vi "Laundry SLB Main.vi"() -> ()   [LabVIEW 2014]
uses:
  type defs/DAQ_States.ctl
  <resource>/objmgr/daqmx.rc
  Utility/Labview GEA2 Toolkit v2.1/GExplorer Support/typedefs/GExplorer_Data_Cluster.ctl
  type defs/ERD_Data_Loop_Control.ctl
  type defs/Error_Command.ctl
  type defs/ERD_Loop_Control_Command.ctl
  <vilib>/DAQmx/write.llb/DAQmx Write (Digital 1D Bool NChan 1Samp 1Line).vi
  <vilib>/DAQmx/write.llb/DAQmx Write (Analog 1D DBL NChan 1Samp).vi
  <vilib>/DAQmx/create/channels.llb/DAQmx Create Channel (CI-Count Edges).vi
  <vilib>/DAQmx/read.llb/DAQmx Read (Counter U32 1Chan 1Samp).vi
  type defs/Cont_Send_States.ctl
  type defs/Cont_Send_Loop_Control_Command.ctl
  type defs/DAQ_Control_Command.ctl
  type defs/GEA2_Control_Command.ctl
  Utility/Labview GEA2 Toolkit v2.1/GEA2 Script/typedefs/Script Info.ctl
  <vilib>/DAQmx/create/channels.llb/DAQmx Create Channel (DO-Digital Output).vi
  <vilib>/DAQmx/create/channels.llb/DAQmx Create Channel (DI-Digital Input).vi
  <vilib>/DAQmx/write.llb/DAQmx Write (Digital Bool 1Line 1Point).vi
  type defs/Fault_Buffer_Status.ctl
  Utility/Save File/Public/Type Definitions/Save File File Paths.ctl
  Utility/Save File/Save File.lvlib
  user32.dll
  Utility/Labview GEA2 Toolkit v2.1/library/GEA2_Toolkit.lvlib
  <vilib>/event_ctls.llb/lveventtype.ctl
  Type Definitions/HCC Program Type.ctl
  Utility/Labview GEA2 Toolkit v2.1/type defs/ERD Write Data In.ctl
  Utility/Labview GEA2 Toolkit v2.1/type defs/ERD Read Data In.ctl
  Utility/Labview GEA2 Toolkit v2.1/type defs/Data In.ctl
  Utility/Labview GEA2 Toolkit v2.1/type defs/Data Out.ctl
  <vilib>/DAQmx/read.llb/DAQmx Read (Digital 1D Bool NChan 1Samp 1Line).vi
  <vilib>/DAQmx/read.llb/DAQmx Read (Digital 1D U8 1Chan NSamp).vi
  <vilib>/DAQmx/configure/timing.llb/DAQmx Timing (Implicit).vi
  <vilib>/DAQmx/create/channels.llb/DAQmx Create Channel (AO-Voltage-Basic).vi
  <vilib>/DAQmx/create/channels.llb/DAQmx Create Channel (CO-Pulse Generation-Frequency).vi
  <vilib>/DAQmx/configure/timing.llb/DAQmx Timing (Sample Clock).vi
  C:/Technology Lab/NI-2010/Trunk/Washer HCC/Washer HCC NEWFI/Washer Soft Load Box/build/data/GeaCommunication.dll
  build/data/GeaCommunication.dll
  type defs/ERD_Always_Show.ctl
  type defs/Cycle_Information.ctl
  type defs/Algorithms.ctl
  type defs/Version.ctl
  type defs/Programming.ctl
  type defs/Select Graph.ctl
  type defs/Motor Control.ctl
  type defs/Cycle Control.ctl
  type defs/MotorProfile.ctl
  type defs/OOB_Kicks.ctl
  type defs/Valves.ctl
  type defs/Redundant.ctl
  <vilib>/Platform/fileVersionInfo.llb/FileVersionInformation.ctl
  Utility/Labview GEA2 Toolkit v2.1/type defs/Source_Destination.ctl
  Utility/Labview GEA2 Toolkit v2.1/type defs/ERD Read Data Out.ctl
  type defs/ERD_Graph.ctl
  type defs/ERD_Graph_All.ctl
  type defs/ATC_Data.ctl
  type defs/Fault_Table_Info.ctl
  type defs/Relays.ctl
  Utility/Save File/Public/Type Definitions/Save File Washer.ctl
  Type Definitions/2015 Program/2015 Cycle Stats.ctl
  Utility/Save File/Public/Type Definitions/Save File Washer Details DOE.ctl
  Utility/Save File/Public/Type Definitions/Save File Unit Type.ctl
  Utility/Save File/Public/Type Definitions/Save File Software Version.ctl
panel:
  in  "Minimize":bool
  in  "Low Power OFF":bool
  out "ERD Data":T1
  out "Timer 2":dbl format="%<%H:%M:%S>t"
  in  "Tab Control 2":enum32{"Page 1", "ERD Read"}(tab)
  out "Washer Details.Serial Number:":string
  out "Washer Details.TR Number:":string
  out "Washer Details.Lab ID:":string
  out "ERD Data Out":T2[](array[typedef]) {"ERD Number" format="%.0x"}
  out "Raw Data Out":string[](array[string])
  in  "Verify ERD Response?":bool
  out "State":enum16{"Run", "Shutdown"}(ring)
  out "Cycle Timer":dbl format="%<%H:%M:%S>t"
  in  "Read Timeout (ms)":u32=5000
  in  "Disable Write":bool
  in  "Disable Read Previous":bool
  in  "Expected Command 2":string=".*"
  in  "Disable Expected Data":bool
  in  "Expected Data 2":string=".*"
  in  "2015 Cycle Stats":T3
  out "Washer In":T4 {"Current" format="%.2f"; "Day Cycle Count" format="%04d"}
  out "New File?":bool
  out "UI Loop":i32
  out "Description 4":string
  out "Exit from SLB":bool
  out "Handle":dbl
  out "Error":i32
  out "Start Save Routine":bool
  in  "Open Lid":bool
  in  "Sample Rate (ms)":u32=1000 min=400 step=100
  in  "Save Log":bool
  in  "Clear Button":bool
  out "Counter":dbl
  in  "Filter Data":bool=TRUE
  in  "UI Launch Button":bool
  in  "Stop":bool
  in  "Data ON":bool=TRUE
  in  "Tab Control":T9(tab)
  out "GEA2 Msg Log":string
  in  "GEA2 Send":T10={"Source"=245, "Destination"=35, "Command"=0, "Message"=""} {"Command" format="%02x"; "Destination" format="%02x"; "Source" format="%02x"}
  in  "Send Button":bool
  out "Version":T11
  in  "Programming":T12 {"Result" items=["InvalidImage", "ImageRejected", "BoardNotFound", "UnableToGetGeaConfiguration", "WriteToFlashNotAllowed", "ImageDownloadedSuccessfully", "ImagePresent", "WriteToFlashFailed", "EraseFailed", "CrcFailed", ""]}
  in  "Start Send":bool
  in  "Msg Rate (ms)":u32=1000 min=50 step=50
  in  "Board Index":i32
  out "Board ID":string
  out "Front Panel Station Label":string
  in  "Number of Cycles/ File":i32=1
  in  "Read ERD":bool
  in  "Write ERD":bool
  in  "ERD Write Data In":T13 {"ERD Number" format="%.0x"}
  in  "GEA Inputs":T14={"Source"=228, "Destination"=35} {"Destination" format="%.0x"; "Source" format="%.0x"}
  out "ERD Output":T15 {"ERD Number" format="%.0x"}
  in  "ERD Read Data In":T16 {"ERD Number" format="%.0x"}
  out "Pressure 2":dbl(graph)
  out "Temp":dbl(graph)
  out "Tub Gallons":dbl(graph)
  in  "Select Graph":T17=enum."Basket Speed (RPM)"
  out "Basket Speed":u16(graph)
  out "Motor Current":dbl(graph)
  out "ERD 3":dbl(graph)
  out "ERD 2":dbl(graph)
  out "ERD 1":dbl(graph)
  in  "Disable Graphs":bool=TRUE
  in  "ERD Graph Cntrl":T18={"ERD 3"={"ERD #"=62250, "Scaler"=32, "Data Type"=enum."uint16_t"}, "ERD 2"={"ERD #"=62250, "Scaler"=32, "Data Type"=enum."uint16_t"}, "ERD 1"={"ERD #"=62250, "Scaler"=32, "Data Type"=enum."uint16_t"}} {"ERD 1"."Scaler" min=1; "ERD 1"."ERD #" format="%.0x"; "ERD 2"."Scaler" min=1; "ERD 2"."ERD #" format="%.0x"; "ERD 3"."Scaler" min=1; "ERD 3"."ERD #" format="%.0x"}
  out "ERD Graph  Ind":T20
  in  "Relays":T21
  in  "Motor Profile":T22
  in  "Test Mode":cluster{"Exit Test Mode":bool}
  in  "LED Control":T23
  in  "Motor Control":T24 {"Amplitude (%)\n-CCW +CW" min=-100 max=100 step=5; "Acceleration" min=-400 max=400 step=10; "Motor Profile Mode" items=["Closed Loop", "Not Implemented", "Open Loop ", "Open Loop Angle ", "Coasting", "Braking", "Idle"]; "Speed (RPM)" min=-800 max=800 step=10}
  in  "Mode Shift":T25
  in  "Recirculation Pump":T26
  in  "Drain Pump":T27
  in  "Lid Lock":T28
  in  "Cycle Control":T29
  in  "Valve Control":T30
  out "Table Buffer Status":T31
  in  "Clear Fault Table":bool
  in  "Get Table Status":bool
  in  "Clear Seq":bool
  in  "Get Faults":bool
  out "Fault Entry 4":T32
  out "Fault Entry 3":T32
  out "Fault Entry 2":T32
  out "Fault Entry 1":T32
  out "Fault Entry 0":T32
  out "Seq Buffer Status":T31
  in  "Clear Fault Buffer":bool
  in  "Get Status":bool
  out "Fault Sequence Buffer":string
  out "Redundant Micro":T33
  in  "Cycle Info Button":bool
  out "Cycle Information":T34
  in  "OOB Kicks":T35
  out "Algorithm Data":T36
  out "ATC Data":T37
  in  "Script Log Path":path
  in  "Script":bool
  out "Script Pass/Fail?":bool
  out "Script Report Text":string
  in  "stop":bool
  in  "Script Path":path
  out "Script Info":T38 {"Overall Script File Progress" scale=0.0..1.0; "Elapsed time (s)" format="%#.1f"; "Current Script Progress" scale=0.0..1.0}
  out "Script Error Out":errorcluster
  in  "LL (M - A)":bool=TRUE
  in  "Lid Lock Feedback":bool
  in  "MS (M - A)":bool=TRUE
  out "DAQ Status":string
  in  "ADC Info Button":bool
  out "Motor Current ADC":u16
  out "Pressure ADC":u16
  out "Drain Pump":bool
  out "Mode Shift":bool
  out "Recirc Pump":bool
  out "Cold Valve":bool
  out "Hot Valve":bool
  out "Spray/Rinse Valve":bool
  out "Fabric SoftValve":bool
  in  "AC Power":bool=TRUE
  in  "Mode Shift FB":bool
  in  "Lid Status":bool=TRUE
  in  "Pressure":dbl(slide) min=0.0 max=5.0 step=0.5 scale=0.0..5.0 scale format="%#_3g"
  in  "Motor Current":dbl(slide)=2.5 min=0.0 max=5.0 step=0.5 scale=0.0..5.0 scale format="%#_3g"
  in  "Turn On DAQ":bool=TRUE
  out "DAQ On?":bool
  in  "Basket RPM":dbl=1.0 min=1.0 max=800.0 step=5.0
  in  "Temperature":dbl(slide)=2.5 min=0.0 max=5.0 step=0.5 scale=0.0..5.0 scale format="%#_3g"
  out "Triac CW":bool
  out "Traic CCW":bool
  out "Temp ADC":u16
  out "CCW":u32
  out "CW":u32
  out "Exe Path":path
  in  "Record Current Status":bool
  out "Error Out":errorcluster
  in  "Error In":errorcluster
  in  "File Locations":T39
  in  "Configuration Path Main":path=path "C:/Newfi Exe/Newfi Exe Locations.ini"
  in  "FileVersionInfo":T6
  out "FileVersionInfo Out":T6
  in  "Robocopy Location Command":string="C:\\Newfi Exe\\Robocopy Update.bat"
  in  "Network Variable Update Rate":u32=1000
  # "Software Version"
  # "Critical Version"
  # "Non-Critical"
  # "XML Crit Ver"
  # "XML Non-Crit"
  # "Daily Build"
  # "Must input a valid ERD# and Data Type\nDO NOT Leave Blank \nIf no scaler use value of 01"
  # "UI"
  # "Wet Load Size"
  # "Dry Load Size"
  # "OOB"
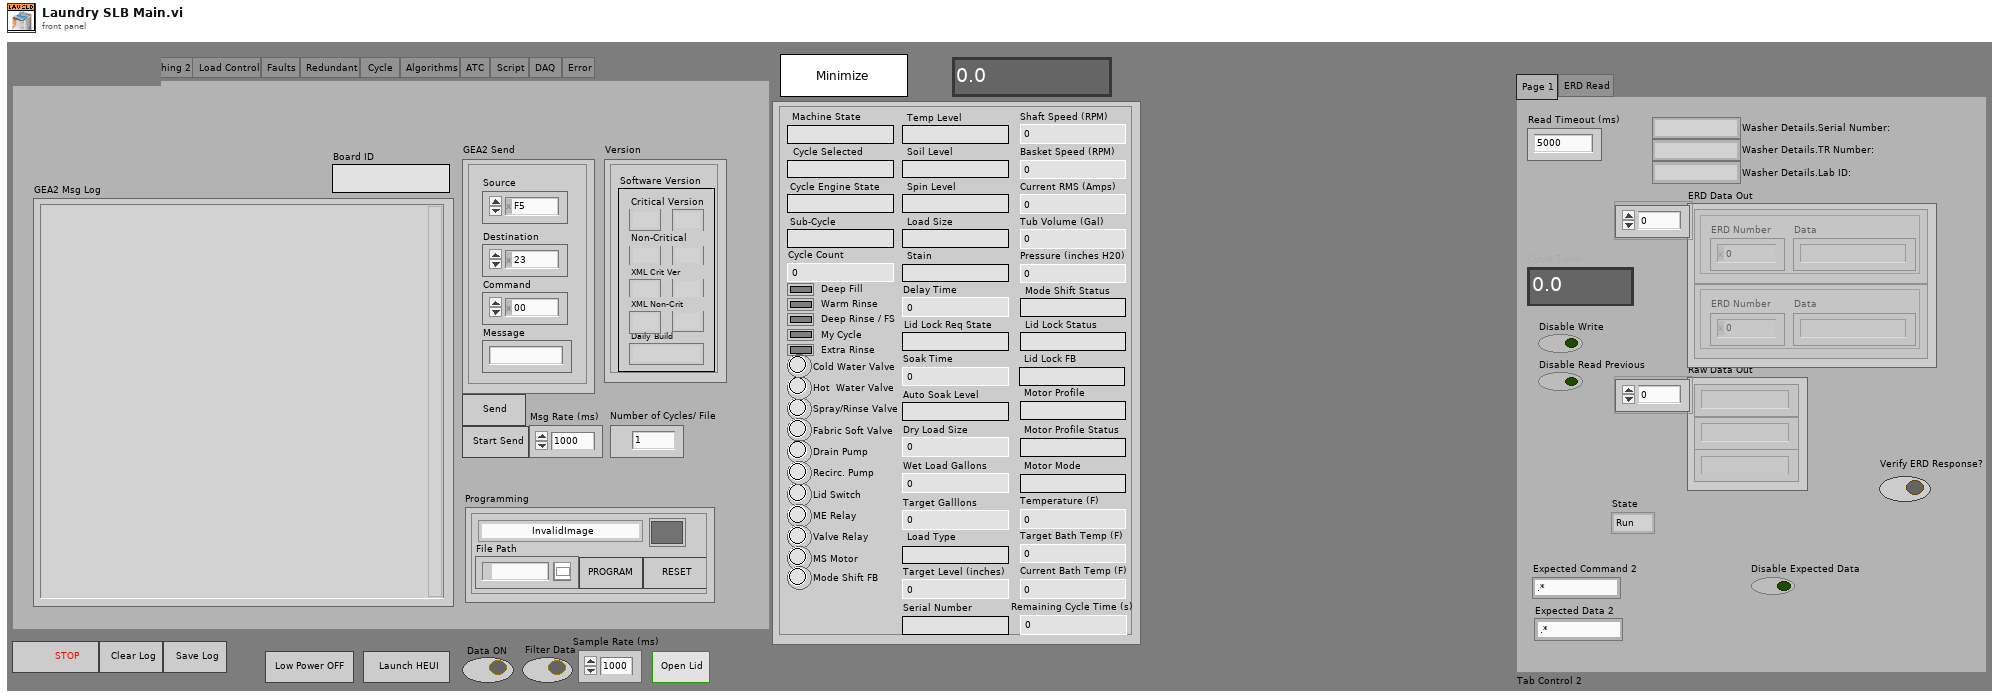
[diagram p1: front panel]
types:
  T1 = typedef "ERD_Always_Show.ctl" = cluster{"Basket Speed (RPM)":u16, "Machine State":string, "Tub Volume (Gal)":dbl, "Pressure (inches H20)":dbl, "Lid Switch ":bool, "Current RMS (Amps)":dbl, "Cycle Selected":string, "Lid Lock Status":string, "Mode Shift Status":string, "Spray/Rinse Valve":bool, "Fabric Soft Valve":bool, "Drain Pump":bool, "Recirc. Pump":bool, "Cycle Engine State":string, "Hot  Water Valve":bool, "Cold Water Valve":bool, "Motor Profile":string, "Motor Profile Status":string, "Motor Mode":string, "ME Relay":bool, "Cycle Count":u32, "Deep Rinse / FS":bool, "My Cycle":bool, "Soil Level":string, "Spin Level":string, "Stain":string, "Temp Level":string, "Load Size":string, "Delay Time":u16, "Soak Time":u16, "Deep Fill":bool, "Warm Rinse":bool, "Auto Soak Level":string, "Extra Rinse":bool, "Wet Load Gallons":dbl, "Target Galllons":dbl, "Sub-Cycle":string, "Load Type":string, "Target Level (inches)":u32, "Valve Relay":bool, "Dry Load Size":dbl, "Shaft Speed (RPM) ":u16, "MS Motor":bool, "Mode Shift FB":bool, "Target Bath Temp (F)":dbl, "Temperature (F)":dbl, "Current Bath Temp (F)":dbl, "Lid Lock FB":string, "Lid Lock Req State":string, "Remaining Cycle Time (s)":dbl, "Serial Number":string}
  T2 = typedef "GEA2_Toolkit.lvlib/ERD Read Data Out.ctl" = cluster{"ERD Number":u16, "Data":string}
  T3 = typedef "2015 Cycle Stats.ctl" = cluster{"Cycle Time (Minutes)":dbl, "Max Temp":dbl, "Max Basket Speed":dbl, "Max Motor Current":dbl, "Max Tub Volume":dbl, "Max Pressure (H2O)":dbl, "Cycle Count":dbl, "Max Shaft Speed ":dbl, "Max Red. Pressure":dbl, "Max. Red Shaft Speed":dbl}
  T4 = typedef "Save File.lvlib/Save File Washer.ctl" = cluster{"Serial Number Display":string, "Day Cycle Count":i32, "Station Label":string, "Status Color":u32, "Current Run Start Time":dbl, "Error?":bool, "Washer Details":T5, "Board ID":string, "Boolean":bool, "RPM":u32, "Current":dbl, "Current Path":path, "Saving":bool, "Unit Type":T7, "Software Version":T8, "Total Time On":dbl}
  T5 = typedef "Save File.lvlib/Save File Washer Details DOE.ctl" = cluster{"Engineer:":string, "Model Number:":string, "Serial Number:":string, "Comments:":string, "Station ID:":string, "Technician:":string, "TR Number:":string, "Lab ID:":string, "Supply Voltage":string, "Water Pressure (PSI):":string, "File Path":path, "Hot Water Temperature (Fahrenheit)":string, "Cold Water Temperature (Fahrenheit)":string, "Capacity (cu.ft)":dbl, "Initial Cloth Weight:":dbl, "Cloth Lot:":i32, "Model Family":string, "Program Name":string, "Cycle Selection":string, "Wash Temperature":string, "Rinse Temperature":string, "Load Size":string, "FileVersionInfo":T6, "Test Date":string, "Computer Name":string, "IP Address":string, "Test Station":string, "Engineer":string, "Test Name":string, "Ambient RH:":string, "Supply Voltage":string, "Frequency:":string, "Build:":string}
  T6 = typedef "FileVersionInformation.ctl" = cluster{"FileVersion":string, "ProductName":string, "InternalName":string, "CompanyName":string, "LegalCopyright":string, "FileDescription":string}
  T7 = typedef "Save File.lvlib/Save File Unit Type.ctl" = enum32{"", "Viper", "Hawk", "2015", "Other"}
  T8 = typedef "Save File.lvlib/Save File Software Version.ctl" = cluster{"Critical Major SW Version":string, "Critical Minor SW Version":string, "Major SW Version":string, "Minor SW Version":string, "Parametric Data Ver. Major":string, "Parametric Data Ver. Minor":string, "Diagnostics Data Ver. Major":string, "Diagnostics Data Ver. Minor":string, "Current Personality Setting":string}
  T9 = enum32{"GEA2", "ERD", "Graphing", "Graphing 2", "Load Control", "Faults", "Redundant", "Cycle ", "Algorithms", "ATC", "Script", "DAQ", "Error"}
  T10 = typedef "GEA2_Toolkit.lvlib/Data In.ctl" = cluster{"Source":u8, "Destination":u8, "Command":u8, "Message":string}
  T11 = typedef "Version.ctl" = cluster{"Critical Major":string, "Critical Minor":string, "Non-Critical Minor":string, "Non-Critical Major":string, "XML Crit Minor":string, "XMLCrit Major":string, "Daily Rev":string, "XML Non-crit Minor":string, "Xml Non-crit Major":string}
  T12 = typedef "Programming.ctl" = cluster{"Program":bool, "File Path":path, "Program Ind":bool, "Result":i32, "Reset Board":bool}
  T13 = cluster{"ERD Number":u16, "Data Type":enum16{"string", "boolean", "uint8_t", "uint16_t", "uint32_t"}, "Data":string}
  T14 = typedef "GEA2_Toolkit.lvlib/Source_Destination.ctl" = cluster{"Source":u8, "Destination":u8}
  T15 = cluster{"ERD Number":u16, "   00 01 02 03 04 05 06 07 08 09 10 11 12 13 14 15 16 17 18 19 ":string}
  T16 = typedef "GEA2_Toolkit.lvlib/ERD Read Data In.ctl" = cluster{"ERD Number":u16, "Data Type":enum16{"string", "boolean", "uint8_t", "uint16_t", "uint32_t", "uint64_t"}}
  T17 = typedef "Select Graph.ctl" = enum16{"Temperature (F)", "Basket Speed (RPM)", "Tub Volume (Gal)", "Pressure (in H2O)", "Current RMS (Amps)", "ERD 1", "ERD 2", "ERD 3"}
  T18 = typedef "ERD_Graph_All.ctl" = cluster{"ERD 3":T19, "ERD 2":T19, "ERD 1":T19}
  T19 = typedef "ERD_Graph.ctl" = cluster{"ERD #":u16, "Scaler":u32, "Data Type":enum16{"string", "boolean", "uint8_t", "uint16_t", "uint32_t"}}
  T20 = cluster{"ERD Value 1":dbl, "ERD Value 2":dbl, "ERD Value 3":dbl}
  T21 = typedef "Relays.ctl" = cluster{"Relays ON":bool, "Relays OFF":bool}
  T22 = typedef "MotorProfile.ctl" = cluster{"Start Profile":bool, "Profile Selection":u8, "Stop Profile":bool, "Pause Profile":bool, "Resume Profile":bool, "Select Profile":bool}
  T23 = cluster{"ALL LEDs ON":bool, "ALL LEDs OFF":bool, "Reset LEDs":bool}
  T24 = typedef "Motor Control.ctl" = cluster{"Speed (RPM)":i16, "Motor Profile Mode":u16, "Acceleration":i16, "Angle (Degrees)":i16, "Amplitude (%)\n-CCW +CW":i16, "Start Motor":bool, "Stop Motor":bool}
  T25 = cluster{"Shift to Agitate":bool, "Shift to Spin":bool, "Disable":bool}
  T26 = cluster{"Recirc Pump ON":bool, "Recirc Pump OFF":bool, "Reset Recirc Pump":bool}
  T27 = cluster{"Dain Pump ON":bool, "Drain Pump OFF":bool, "Reset Drain Pump":bool}
  T28 = cluster{"Lock Lid":bool, "Unlock Lid":bool, "Reset Lock":bool}
  T29 = typedef "Cycle Control.ctl" = cluster{"Start Cycle":bool, "Cycle Selection":u8, "Stop Cycle":bool, "Pause Cycle":bool, "Resume Cycle":bool, "Select Cycle":bool}
  T30 = typedef "Valves.ctl" = cluster{"Cold Valve":bool, "SprayRinse Valve":bool, "FabricSoftener Valve":bool, "Valves ON":bool, "Valves OFF":bool, "Hot Valve ":bool}
  T31 = typedef "Fault_Buffer_Status.ctl" = cluster{"Current Index":u16, "Count":u16, "Overwrite Count":u16}
  T32 = typedef "Fault_Table_Info.ctl" = cluster{"Cycle Count":u32, " Runtime (min) ":u32, "Fault Status":string, "Fault ID":string, "Fault Count":u16}
  T33 = typedef "Redundant.ctl" = cluster{"Version":string, "Personality":u8, "Pressure ":dbl, "Shaft Speed":u16, "Modeshift Feedback":string, "Lid Switch":bool, "Lid Lock":bool, "Triac Enable":bool, "Drain Pump":bool, "Lid Lock Motor Speed Safety Interlock":bool, "Flood Condition State":bool, "Lid Open Fault State":bool, "Access To Moving Parts State":bool, "Heartbeat":bool, "Motor Enable":bool, "Lid Unlock Fault State":bool}
  T34 = typedef "Cycle_Information.ctl" = cluster{"MyCycle":bool, "Delay":bool, "Extra Rinse":bool, "Deep Fill":bool, "AutoSoak":bool, "Deep Rinse":bool, "Warm Rinse":bool, "Delay Time":string, "Stain":string, "Autosoak Time":string, "Cycle Selection":string, "Stain":bool}
  T35 = typedef "OOB_Kicks.ctl" = cluster{"OOB in Accel":bool, "OOB in S-S":bool, "Redist Req":bool}
  T36 = typedef "Algorithms.ctl" = cluster{"Wet Load Gal":dbl, "Target Gallons":dbl, "Load Type":string, "Load Size":string, "Coast Time":u16, "Ramp Time":u16, "Ramp  Speed":u16, "Ramp Avg Current":dbl, "OOB Redist Req":bool, "OOB Detected in S-S":bool, "Max Accel in Accel":i32, "Max Jerk in Accel":i32, "Max Jerk in S-S":i32, "OOB Detected in Accel":bool, "Partial Coast Time":u16, "Dry Load Size":dbl, "Ramp Line Voltage ":dbl, "Coast Line Voltage":dbl}
  T37 = typedef "ATC_Data.ctl" = cluster{"Current Tub Gallons":dbl, "Hot Gallons":dbl, "Cold Gallons":dbl, "Target Gallons":dbl, "Current Water Temp":dbl, "Target Level":u32, "Target Bath Temp":dbl, "Current Bath Temp ":dbl, "Cold Inlet Temp":dbl, "Hot Inlet Temp":dbl, "Warm Inlet Temp":dbl, "Hot Seg Valve Time":u16, "Cold Seg Valve Time ":u16, "User Temp Level":string, "Segment Gallons":dbl}
  T38 = typedef "Script Info.ctl" = cluster{"Overall Script File Progress":dbl, "Current Script Progress":dbl, "Script":string, "Test":string, "Elapsed time (s)":dbl, "Done?":bool}
  T39 = typedef "Save File.lvlib/Save File File Paths.ctl" = cluster{"Log Debug File":path, "Log Inverter File":path, "Summary File":path, "Bus File":path, "Current (Amps) File":path}
  T40 = typedef "GEA2_Toolkit.lvlib/ERD Write Data In.ctl" = cluster{"ERD Number":u16, "Data Type":enum16{"string", "boolean", "uint8_t", "uint16_t", "uint32_t"}, "Data":string}
  T41 = typedef "HCC Program Type.ctl" = enum16{"Viper Hawk", "2015"}
  T42 = typedef "Cont_Send_States.ctl" = enum16{"Run", "Shutdown"}
  T43 = typedef "DAQ_States.ctl" = enum16{"Wait for Init", "Verify Hardware", "Initialize", "Run", "Shutdown", "Exit"}
  T44 = typedef "ERD_Data_Loop_Control.ctl" = cluster{"Data":variant, "State":enum16{"Run", "Shutdown"}}
  T45 = typedef "GEA2_Toolkit.lvlib/Data Out.ctl" = cluster{"Source":u8, "Destination":u8, "Command":u8, "Length":u8, "CRC":u16, "Message":string}
  T46 = typedef "GExplorer_Data_Cluster.ctl" = cluster{"Data":variant, "State":enum16{"Add to Log", "Clear", "Shutdown"}}
  T47 = typedef "ViperHawk Data.ctl" = cluster{"Message Count":dbl, "ReceivedData":u8[], "Partial Message String":string, "Full Message to Save":string, "Data to send":u8[], "Command":u8, "logData":T48, "Number of Messages":i32, "Debug":string[][], "Washer In":T4, "Configuration File Path out":path}
  T48 = typedef "ViperHawk logData.ctl" = cluster{"IGBT Temp (Deg C)":u8, "Speed":u32, "Load Size":u32, "Temperature":u8, "Water Pressure":u32, "Detergent":u32, "Fabric Softener":u32, "Direction":string, "Det":bool, "FS":bool, "Recirc":bool, "Drain":bool, "Hot":bool, "Cold":bool, "LidClosed":bool, "LidLocked":bool, "Motor Speed":u16, "Latched Out Of Balance":u16, "Raw Out Of Balance":u16, "Plaster Status":u8, "Inverter Power (Watts)":u16, "Profiler Status":string, "Profiler CRC":u16, "Current Inverter Action":string, "Target Speed (BRPM)":u16, "Latched Agitate Motor Temp (Deg C)":u8, "Current Motor Temp (Deg C)":u8, "Error Codes 1":string}
  T49 = typedef "ViperHawk Timers.ctl" = cluster{"Cycle Timer":dbl, "Timer":dbl}
  T50 = typedef "Save File.lvlib/Save File FileName Control.ctl" = cluster{"Debug File DIR":string, "Inverter And MC File DIR":string}
  T51 = typedef "ViperHawk Search Control.ctl" = cluster{"Pause":string[], "Run":string[], "EOC":string[], "Error Codes":string[]}
  T52 = typedef "ViperHawk Diagnostic Data.ctl" = cluster{"Cycle Buffer Index":string, "Page Number":string, "Total Cycle Count":u32, "Delay Start Time":u32, "Stain Selected":string, "Selected Cycle":u32, "eWash":string, "Soil Level":string, "Temperature":string, "Overnight Ready":string, "Spin Setting":string, "Control Lock Status":string, "Stain Remover":string, "Steam Assist":string, "My Cycle":string, "PreWash":string, "Debug Log Enabled":string, "Rinse":string, "Signal Level":string, "PreSoak":string, "Speed (RPM)":u32, "Load Size":u32, "Temperature":u32, "Water Pressure":u32, "Detergent":u32, "Fabric Softener":u32, "Tub Direction":string, "Detergent Valve":bool, "Fabric Softener Valve":bool, "Recirculating Pump":bool, "Drain Valve":bool, "Hot Valve":bool, "Cold Valve":bool, "Lid Closed Status":string, "Lid Lock Status":string, "Error Count":u32, "IGBT Temperature (Deg C)":u32, "Motor Speed":u32, "Latched OOB":u32, "Raw OOB":u32, "Plaster Status":u32, "Inverter Power (W)":u32, "Target Speed(BRPM)":u32, "Latched Agitate Motor Temp (Deg C)":u32, "Current Motor Temp (Deg C)":u32, "Profiler Status":string, "Current Inverter Action":string, "Error Codes":string, "Total Cycle Time (Min)":u32, "Total Cycle Count (Current)":u16, "Total Error Count":u16, "Machine Error History":u32, "Washer UI History":u32, "Inverter Error History":u32, "Cycle Storage Limit":u8, "Error Storage Limit":u8, "Cycle Pages Supported":u8, "Error Pages Supported":u8, "Inverter Reset Count":u16}
  T53 = cluster{"Initialize":T47, "Timers":T49, "Configuration Startup Directorys":T50, "Debug Search Parameters":T51, "Log Debug and Inv? Startup":bool, "Board Index Startup":i32, "File Locations":T39, "GeaCommunication.GeaBus":refnum<k24>, "GEA2 Event Registration":refnum<event-registration>, "New Summary Created":bool, "Files Already Exist":bool, "Diagnostic":T52}
  T54 = typedef "LabVIEW_GEA2_Toolkit.lvlibp/Data In.ctl" = cluster{"Source":u8, "Destination":u8, "Command":u8, "Message":string}
  T55 = enum8{"Enabled", "Disabled", "Disabled and Grayed Out"}
  T56 = typedef "GEA2_Control_Command.ctl" = enum16{"Initialize", "Shutdown"}
  T57 = typedef "DAQ_Control_Command.ctl" = enum16{"Initialize", "Shutdown"}
  T58 = typedef "Cont_Send_Loop_Control_Command.ctl" = enum16{"Initialize", "Shutdown"}
  T59 = typedef "ERD_Loop_Control_Command.ctl" = enum16{"Initialize", "Shutdown"}
  T60 = cluster{"ERD Number":u16, "Data Type":enum16{"string", "boolean", "uint8_t", "uint16_t", "uint32_t"}, "Data":string}[]
  T61 = enum32{"Invalid", "Standard", "Closed", "Hidden", "Minimized", "Maximized"}
  T62 = enum32{"invalid app kind", "Development System", "Run Time System", "Student Edition", "Embedded LabVIEW", "Evaluation", "Custom"}
  T63 = enum16{"Read Viper", "Write Viper", "Read 2015", "Write 2015"}
  T64 = cluster{"Core":cluster{"Current VI Reference":refnum<vi>, "Close Panel on Exit?":bool}, "File Locations":T39, "Washer In":T4, "File Refnum":refnum<file>, "FileVersionInfo":T6, "2015 Cycle Stats":T3, "ERD Data Save":T1}
  T65 = cluster{"Current VI Reference":refnum<vi>, "Close Panel on Exit?":bool}
  T66 = typedef "lveventtype.ctl" = enum32{"Null", "Timeout", "Annotation Menu Selection", "Annotation Menu Selection?", "App Instance Close", "App Instance Close?", "Autoscale Range Change", "Bookmark Info Change", "Cell Edit", "Cell Edit?", "Cursor Grab", "Cursor Grab?", "Cursor Menu Selection", "Cursor Menu Selection?", "Cursor Move", "Cursor Release", "Data Change", "Direction Change", "Display State Change", "Drag Ended", "Drag Enter", "Drag Leave", "Drag Over", "Drag Source Update", "Drag Starting", "Drag Starting?", "Drop", "Exec State Change", "Key Down", "Key Down?", "Key Repeat", "Key Repeat?", "Key Up", "Listbox Double Click", "Menu Activation?", "Menu Selection (App)", "Menu Selection? (App)", "Menu Selection (User)", "Mouse Down", "Mouse Down?", "Mouse Enter", "Mouse Leave", "Mouse Move", "Mouse Up", "Mouse Wheel", "NI Security User Change (App)", "Pane Size", "Panel Close", "Panel Close?", "Panel Resize", "Plot Attribute Change", "Scale Range Change", "Shortcut Menu Activation?", "Shortcut Menu Selection (App)", "Shortcut Menu Selection? (App)", "Shortcut Menu Selection (User)", "Tree Double Click", "Tree Drag", "Tree Drag?", "Tree Drop", "Tree Drop?", "Tree Item Close", "Tree Item Close?", "Tree Item Open", "Tree Item Open?", "User Event", "Value Change"}
  T67 = typedef "Error_Command.ctl" = enum16{"Initialize", "Handle Errors", "Report Errors"}
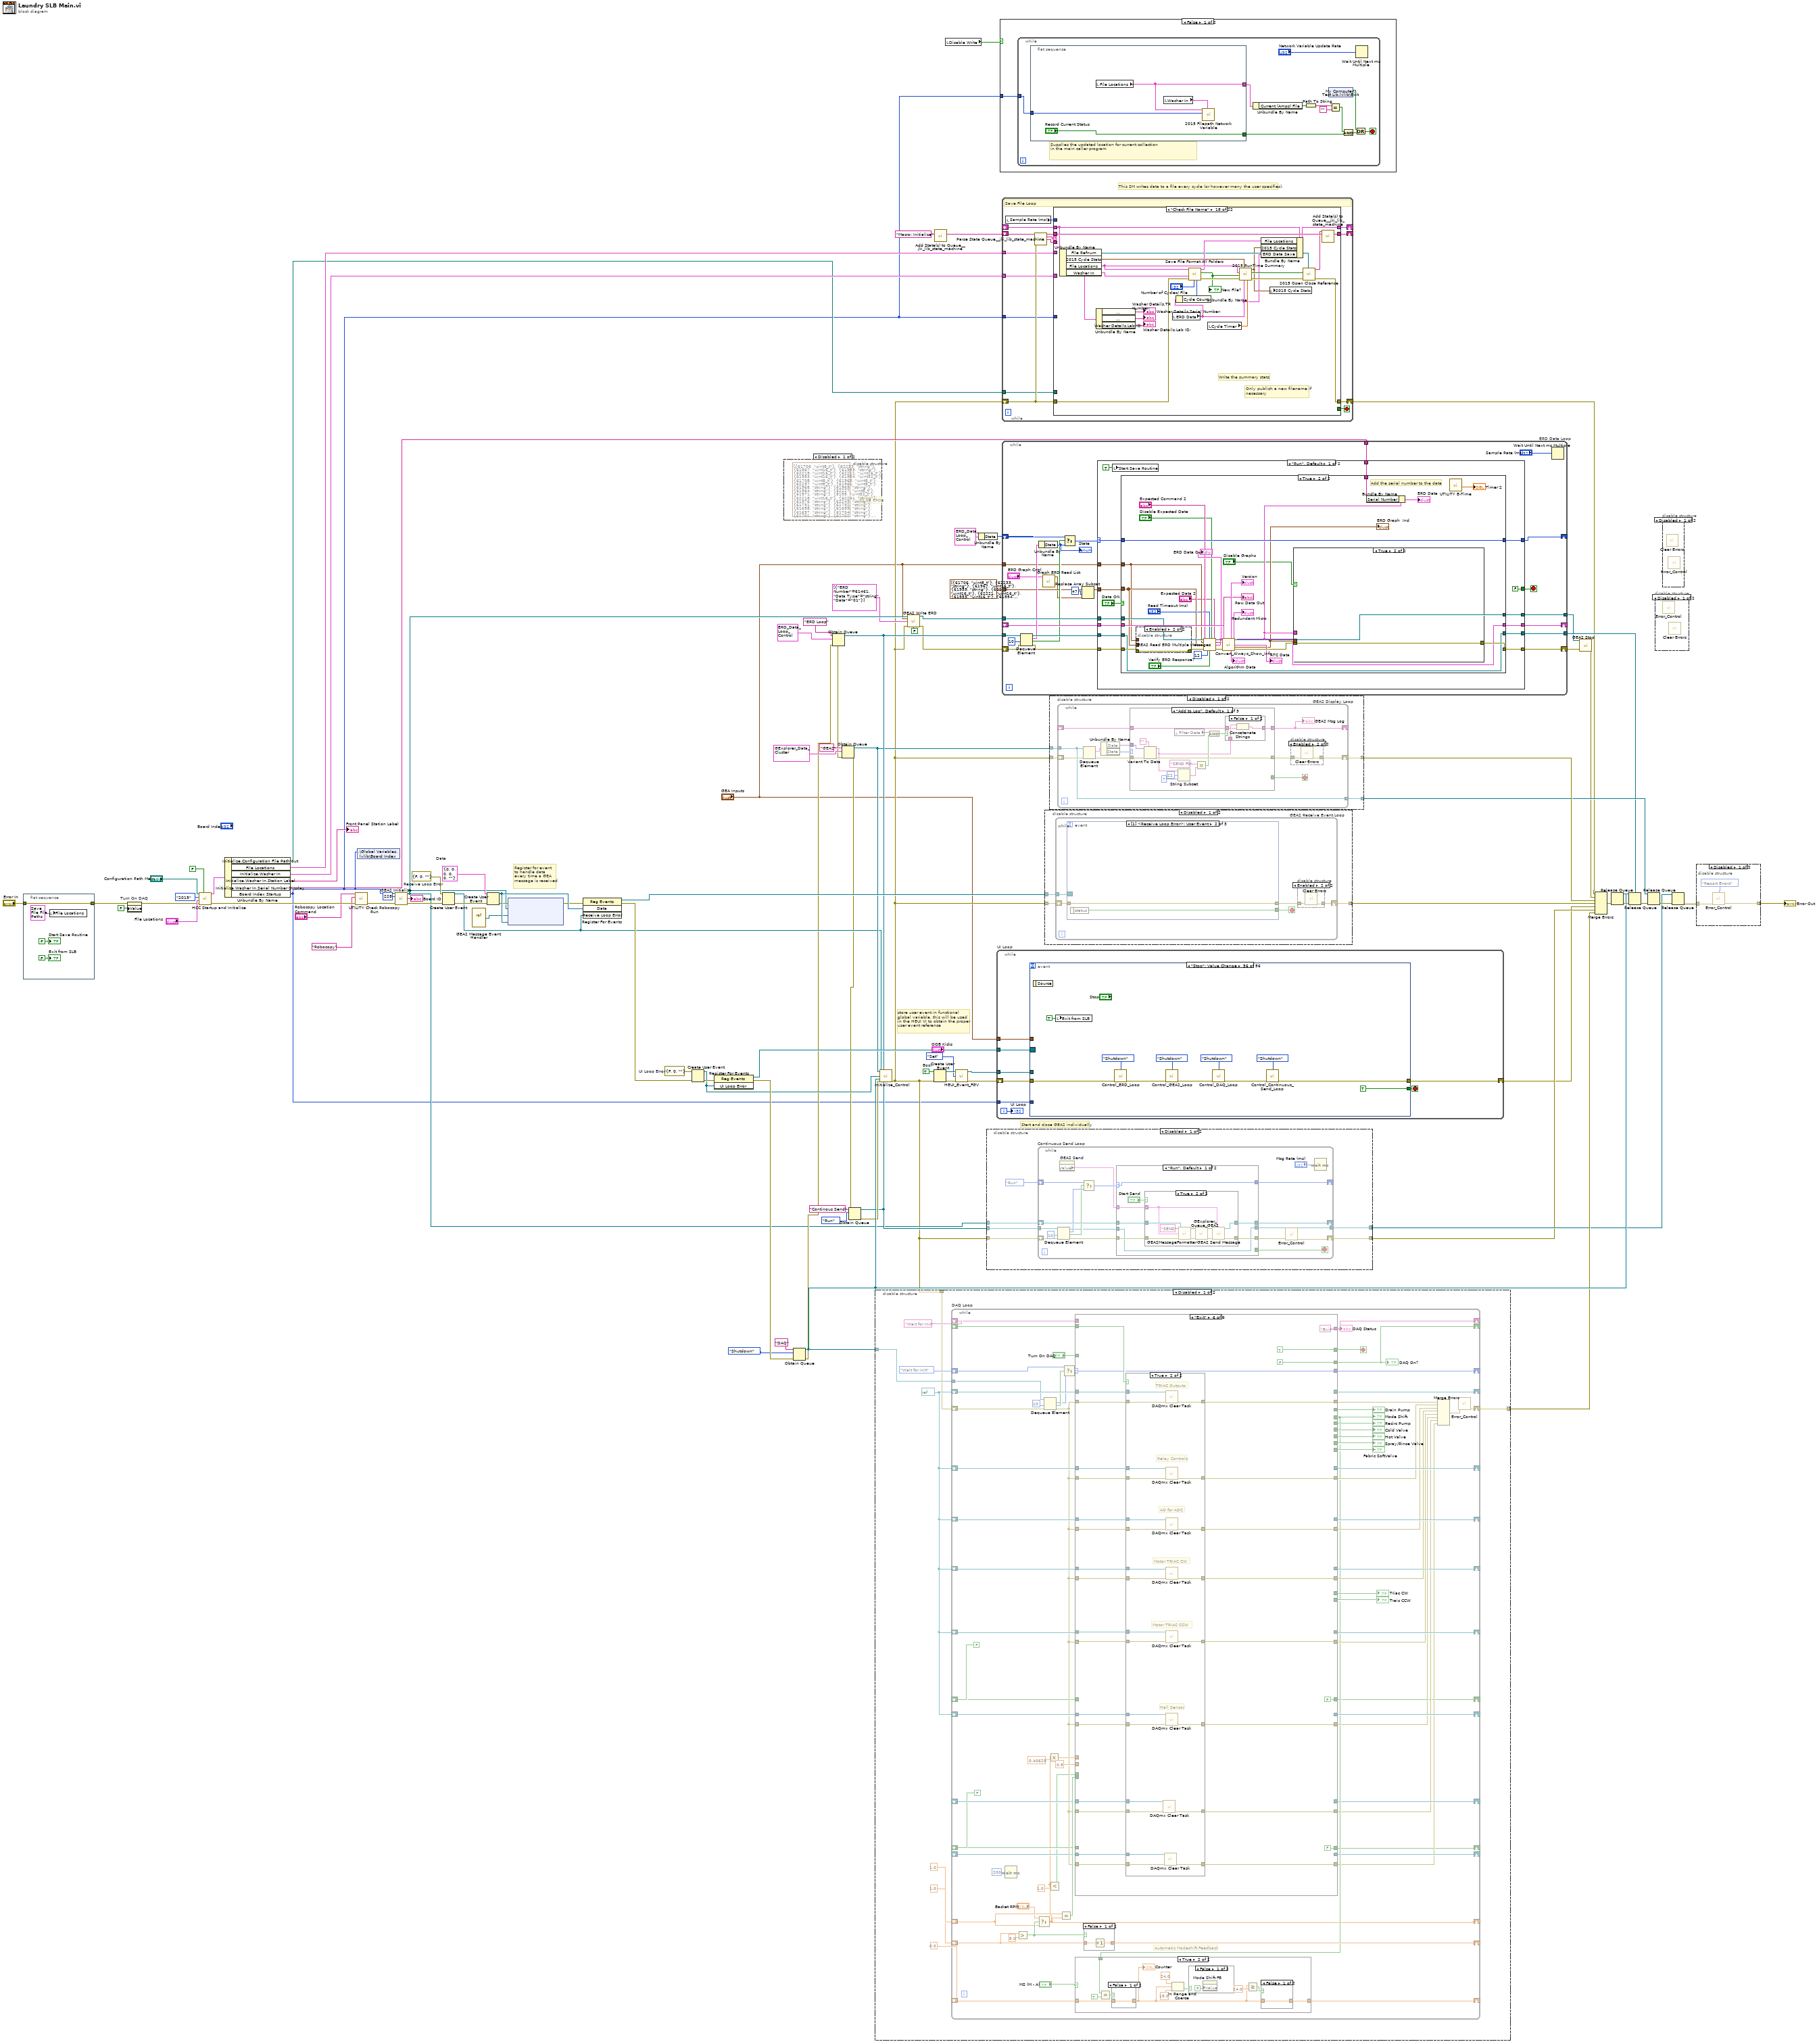
[diagram p0: block diagram]
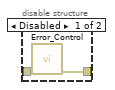
[diagram p6: hidden frame]
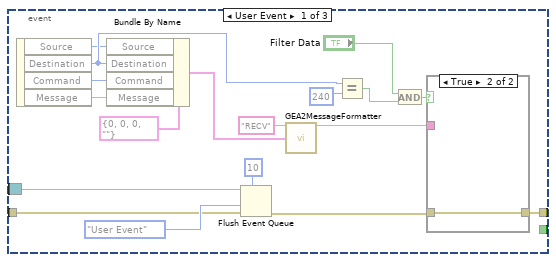
[diagram p7: hidden frame]
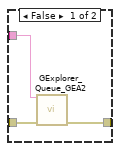
[diagram p8: hidden frame]
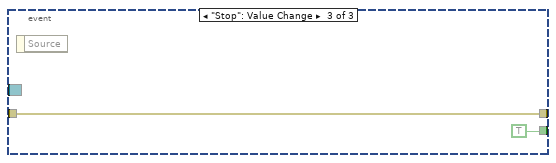
[diagram p9: hidden frame]
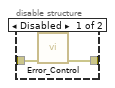
[diagram p11: hidden frame]
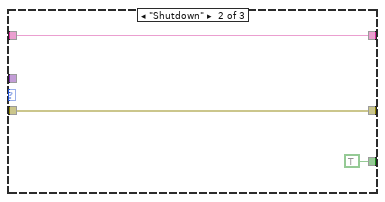
[diagram p13: hidden frame]
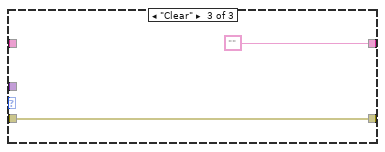
[diagram p14: hidden frame]
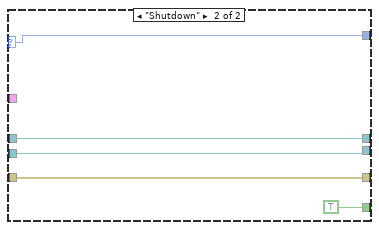
[diagram p18: hidden frame]
diagram:
  w42 = TRUE  # Bool
  w70 = errorcluster {"status"=FALSE, "code"=0, "source"=""}  # UI Loop Error
  w71 = errorcluster {"status"=FALSE, "code"=0, "source"=""}  # Receive Loop Error
  w75 = T45 {"Source"=0, "Destination"=0, "Command"=0, "Length"=0, "CRC"=0, "Message"=""}  # Data
  # "Start and close GEA2 individually"
  # "This SM writes data to a file every cycle (or however many the user specifies)."
  # "store user event in functional\nglobal variable, this will be used\nin the HEUI VI to obtain the proper\nuser event reference"
  # "Register for event\nto handle data\nevery time a GEA\nmessage is received"
  n1 = flat-sequence {
    tunnel: "Error In" -> [w93]
    tunnel: [w93] -> w30
    frame #0 {
      n2 = local write "File Locations"(T39 {"Log Debug File"=path "", "Log Inverter File"=path "", "Summary File"=path "", "Bus File"=path "", "Current (Amps) File"=path ""} ("File Locations")) -> ()
      "Start Save Routine" <- FALSE ("Start Save Routine")
      "Exit from SLB" <- FALSE ("Exit from SLB")
    }
  }
  n3 = property on="Turn On DAQ" class="Bool (strict)"(error in=w30, "Value"=FALSE ("Turn On DAQ")) -> (error out=w29:errorcluster)  [unwired: 1 in, 1 out]
  n4 = call "HCC Startup and Initialize.vi"("Debug"=FALSE, "error in (no error)"=w29, "File Locations"="File Locations", "Program"=HCC_Program_Type."2015", "Configuration Path Main"="Configuration Path Main") -> ("error out"=w7:errorcluster, "Initialization"=w35:T53)  [unwired: 5 in]
  n5 = Unbundle By Name(w35) -> ("Initialize.Configuration File Path out"=w23:path, "File Locations"=w25:T39, "Initialize.Washer In"=w26:T4, "Initialize.Washer In.Station Label"=→"Front Panel Station Label":string, "Initialize.Washer In.Serial Number Display"=w32:string, "Board Index Startup"=w3:i32)
  n6 = call "UTILITY Check Robocopy Run.vi"("error in (no error)"=w7, "Refresh Programs Named"="Robocopy", "Robocopy Location Command"="Robocopy Location Command") -> ("error out"=w6:errorcluster)  [unwired: 8 in]
  n7 = shared-variable ".\\Global Variables.lvlib\\Board Index"(w3) -> ()  [unwired: 1 in, 1 out]
  n8 = call "GEA2 Initialize.vi"("Board Index"=w3, "Source Address"=u8 228, "error in"=w6) -> ("GeaCommunication.GeaBus"=w15:refnum<k24>, "Board ID"=→"Board ID":string, "error out"=w73:errorcluster)  [unwired: 10 in]
  n9 = Create User Event(user event datatype=w71, error in=w73) -> (user event=w58:refnum<user-event>, error out=w72:errorcluster)
  n10 = vi-ref "GEA2 Message Event Handler.vi"() -> (w24:refnum<vi>)
  n11 = Create User Event(user event datatype=w75, error in=w72) -> (user event=w78:refnum<user-event>, error out=w77:errorcluster)
  n12 = node(w77, w15, w24, w78) -> (w76:errorcluster)  [unwired: 1 in, 1 out]
  n13 = register-events(error in=w76, w78, w58) -> (reference out=w74:refnum<event-registration>, error out=w66:errorcluster)  [unwired: 1 in]
  n14 = Create User Event(user event datatype=w70, error in=w66) -> (user event=w57:refnum<user-event>, error out=w69:errorcluster)
  n15 = register-events(error in=w69, w57) -> (reference out=w68:refnum<event-registration>, error out=w67:errorcluster)  [unwired: 1 in]
  n16 = disable-structure shown="Disabled" {
    frame Disabled {
      (unwired) T16[] [{"ERD Number"=61706, "Data Type"=enum."uint8_t"}, {"ERD Number"=62233, "Data Type"=enum."string"}, {"ERD Number"=61967, "Data Type"=enum."uint16_t"}, {"ERD Number"=61959, "Data Type"=enum."string"}, {"ERD Number"=62219, "Data Type"=enum."uint16_t"}, {"ERD Number"=62221, "Data Type"=enum."uint16_t"}, {"ERD Number"=61953, "Data Type"=enum."uint16_t"}, {"ERD Number"=61954, "Data Type"=enum."uint32_t"}, {"ERD Number"=61708, "Data Type"=enum."uint8_t"}, {"ERD Number"=61963, "Data Type"=enum."uint8_t"}, {"ERD Number"=62237, "Data Type"=enum."uint8_t"}, {"ERD Number"=61961, "Data Type"=enum."uint8_t"}, {"ERD Number"=61968, "Data Type"=enum."string"}, {"ERD Number"=61969, "Data Type"=enum."string"}, {"ERD Number"=61964, "Data Type"=enum."string"}, {"ERD Number"=62227, "Data Type"=enum."uint8_t"}, {"ERD Number"=61971, "Data Type"=enum."string"}, {"ERD Number"=8195, "Data Type"=enum."uint32_t"}, {"ERD Number"=62218, "Data Type"=enum."uint16_t"}, {"ERD Number"=62241, "Data Type"=enum."string"}, {"ERD Number"=61976, "Data Type"=enum."string"}, {"ERD Number"=62243, "Data Type"=enum."string"}, {"ERD Number"=61731, "Data Type"=enum."string"}, {"ERD Number"=61732, "Data Type"=enum."string"}, {"ERD Number"=61698, "Data Type"=enum."string"}, {"ERD Number"=61699, "Data Type"=enum."string"}, {"ERD Number"=61697, "Data Type"=enum."string"}, {"ERD Number"=61704, "Data Type"=enum."string"}, {"ERD Number"=61701, "Data Type"=enum."string"}, {"ERD Number"=61702, "Data Type"=enum."string"}, {"ERD Number"=61705, "Data Type"=enum."string"}, {"ERD Number"=61703, "Data Type"=enum."string"}, {"ERD Number"=61709, "Data Type"=enum."uint16_t"}, {"ERD Number"=61710, "Data Type"=enum."uint16_t"}, {"ERD Number"=61726, "Data Type"=enum."string"}, {"ERD Number"=62213, "Data Type"=enum."uint16_t"}, {"ERD Number"=61952, "Data Type"=enum."uint16_t"}, {"ERD Number"=61957, "Data Type"=enum."uint16_t"}, {"ERD Number"=61958, "Data Type"=enum."string"}, {"ERD Number"=61973, "Data Type"=enum."uint32_t"}, {"ERD Number"=62242, "Data Type"=enum."string"}, {"ERD Number"=256, "Data Type"=enum."string"}, {"ERD Number"=61441, "Data Type"=enum."string"}, {"ERD Number"=61457, "Data Type"=enum."string"}, {"ERD Number"=61984, "Data Type"=enum."uint16_t"}, {"ERD Number"=61985, "Data Type"=enum."uint16_t"}] ("Read ERD List")
      # "v1.16 ERDs"
    }
    frame Enabled {
    }
  }
  n17 = Obtain Queue(name (unnamed)="DAQ", element data type=DAQ_States."Shutdown" ("t"), error in (no error)=w67) -> (queue out=w56:refnum<queue>, error out=w19:errorcluster)  [unwired: 2 in, 1 out]
  n18 = Obtain Queue(name (unnamed)="ERD Loop", element data type=T44 {"Data"=variant, "State"=enum."Run"} ("Data"), error in (no error)=w19) -> (queue out=w60:refnum<queue>, error out=w61:errorcluster)  [unwired: 2 in, 1 out]
  n19 = Obtain Queue(name (unnamed)="GEA2", element data type=T46 {"Data"=variant, "State"=enum."Add to Log"} ("Data"), error in (no error)=w61) -> (queue out=w59:refnum<queue>, error out=w51:errorcluster)  [unwired: 2 in, 1 out]
  n20 = Obtain Queue(name (unnamed)="Continous Send", element data type=Cont_Send_States."Run" ("State"), error in (no error)=w51) -> (queue out=w45:refnum<queue>, error out=w50:errorcluster)  [unwired: 2 in, 1 out]
  n21 = call "Initialize_Control.vi"("GEA2"=w59, "ERD Loop"=w60, "Receive Loop Error"=w58, "UI Loop Error"=w57, "DAQ"=w56, "Error In"=w50, "Cont Send"=w45) -> ("Error Out"=w12:errorcluster)  [unwired: 8 in]
  n22 = disable-structure shown="Disabled" {
    disable-tunnel: w56 -> [w104 _]
    disable-tunnel: [w100 _] -> w53
    disable-tunnel: w12 -> [w96 _]
    frame Disabled {
      w98 = refnum<k21> refnum ("task out")
      n23 = while "DAQ Loop" {
        tunnel: w104 -> [w169]
        shift-right: [w154] -> w100
        shift-left: w96 -> [w170]
        shift-right: [w144] -> _
        shift-left: w98 -> [w176]
        shift-right: [w173] -> _
        shift-left: w98 -> [w174]
        shift-right: [w171] -> _
        shift-left: w98 -> [w172]
        shift-right: [w124] -> _
        shift-left: DAQ_States."Wait for Init" ("States") -> [w160]
        shift-right: [w165] -> _
        shift-left: w98 -> [w166]
        shift-right: [w163] -> _
        shift-left: w98 -> [w164]
        shift-right: [w125] -> _
        shift-left: _ -> [w153]
        shift-right: [w107] -> _
        shift-left: 1.0 -> [w130]
        shift-right: [w142] -> _
        shift-left: 0.0 -> [w143]
        shift-right: [w138] -> _
        shift-left: w98 -> [w137]
        shift-right: [w134] -> _
        shift-left: 1.0 -> [w132]
        shift-right: [w128] -> _
        shift-left: "Wait for Init" ("Report Text") -> [w127]
        shift-right: [w123] -> _
        shift-left: _ -> [w118]
        shift-right: [w120] -> _
        shift-left: _ -> [w117]
        shift-right: [w115] -> _
        shift-left: FALSE -> [w116]
        shift-right: [w109] -> _
        shift-left: FALSE -> [w110]
        stop <- w145 stop-if-true
        # "Automatic Modeshift Feedback"
        n24 = Wait (ms)(milliseconds to wait=u32 200) -> ()  [unwired: 1 out]
        n25 = Greater?(x=w132, y=5.0 ("x")) -> (0:w133:bool)
        n26 = Select(t="Basket RPM", s=w133, f=w130) -> (s? t:f=w107:dbl)
        n27 = Dequeue Element(queue=w169, timeout in ms (-1)=10, error in (no error)=w170) -> (element=w156:T43, timed out?=w161:bool, error out=w121:errorcluster)  [unwired: 1 out]
        n28 = Multiply(x=w107, y=0.40625) -> (x*y=w106:dbl)
        n29 = Less?(x=w107, y=1.0) -> (x < y?=w111:bool)
        n30 = Equal?(x=w130, y=w107) -> (x = y?=w152:bool)
        n31 = Select(t=w160, s=w161, f=w156) -> (s? t:f=w168:T43)
        n32 = case shown="\"Exit\"" w168 {
          selector: w168 -> [_ _ _ _ _ w584]
          tunnel: w176 -> [w217 w233 _ w461 w566 w598]
          tunnel: [w217 w233 w340 w460 _ _] -> w144
          tunnel: [w222 w230 w341 w458 w565 w587] -> w159
          tunnel: w174 -> [w220 w240 _ w457 w557 w597]
          tunnel: [w220 w240 w346 w452 _ _] -> w173
          tunnel: w172 -> [w218 w243 _ w451 w552 w583]
          tunnel: [w218 w243 w351 w448 _ _] -> w171
          tunnel: w121 -> [w222 w239 w342 w447 w567 w599]
          tunnel: w121 -> [w221 w241 w347 w446 w556 w578]
          tunnel: w121 -> [w219 w242 w289 w445 w553 w595]
          tunnel: [w219 w242 w350 w444 w529 w589] -> w157
          tunnel: [w221 w241 w345 w443 w536 w588] -> w158
          tunnel: [w209 w236 DAQ_States."Run" ("t") w414 DAQ_States."Wait for Init" ("States") w584] -> w124
          tunnel: [FALSE FALSE TRUE TRUE FALSE FALSE] -> w125
          tunnel: w166 -> [w215 w247 _ w396 w563 w592]
          tunnel: w121 -> [w216 w249 w306 w395 w562 w593]
          tunnel: [w216 w249 w336 w440 w545 w591] -> w139
          tunnel: [w215 w247 w337 w441 _ _] -> w165
          tunnel: w152 -> [_ _ _ w389 _ _]
          tunnel: 0.5 ("Duty Cycle") -> [_ _ w338 w383 _ _]
          tunnel: w121 -> [w214 w248 w313 w431 w561 w594]
          tunnel: [w214 w248 w297 w429 w528 w590] -> w140
          tunnel: w164 -> [w213 w246 _ w428 w560 w582]
          tunnel: [w213 w246 w302 w430 _ _] -> w163
          tunnel: [_ _ _ _ FALSE TRUE] -> w145
          tunnel: w153 -> [_ _ _ _ _ w596]
          tunnel: [_ _ _ w438 _ _] -> w151
          tunnel: [_ _ _ w432 _ _] -> w129
          tunnel: [_ _ _ w437 _ _] -> w150
          tunnel: [_ _ _ w436 _ _] -> w149
          tunnel: [_ _ _ w435 _ _] -> w148
          tunnel: [_ _ _ w434 _ _] -> w147
          tunnel: [_ _ _ w433 _ _] -> w146
          tunnel: w121 -> [w212 w244 w317 w427 w527 w581]
          tunnel: [w212 w244 w294 w426 w525 w579] -> w141
          tunnel: [w211 w245 w291 w424 _ _] -> w138
          tunnel: w137 -> [w211 w245 _ w425 w526 w580]
          tunnel: [_ _ _ w423 _ _] -> w136
          tunnel: [_ _ _ w419 _ _] -> w135
          tunnel: [w210 w232 "Initialize" ("Report Text") "Running" ("Report Text") "Wait for Init" ("Report Text") "Exit" ("Report Text")] -> w128
          tunnel: w127 -> [w210 _ _ _ _ _]
          tunnel: "Turn On DAQ" -> [w208 _ _ w415 _ _]
          tunnel: [w203 w227 w274 w405 w517 w574] -> w122
          tunnel: [w204 w228 w271 w404 _ _] -> w123
          tunnel: w121 -> [w203 w227 w270 w407 w518 w575]
          tunnel: w121 -> [w200 w224 w268 w400 w514 w572]
          tunnel: [w202 w226 w267 w402 _ _] -> w120
          tunnel: [w200 w224 w266 w403 w516 w571] -> w119
          tunnel: w118 -> [w204 w228 _ w406 w519 w576]
          tunnel: w117 -> [w202 w226 _ w401 w513 w573]
          tunnel: w116 -> [w201 w225 w265 w399 _ _]
          tunnel: [w201 w225 w265 w398 FALSE FALSE] -> w115
          tunnel: w111 -> [_ _ _ w388 _ _]
          tunnel: w110 -> [_ _ _ w392 _ _]
          tunnel: [FALSE FALSE FALSE w384 FALSE FALSE] -> w109
          tunnel: w106 -> [_ _ w254 w382 _ _]
          frame "Wait for Init", Default {
            # "Hall Sensor"
            # "Motor TRIAC CCW"
            # "Motor TRIAC CW"
            # "Relay Controls"
            # "TRIAC Outputs"
            # "AO for ADC"
            n33 = Select(t=DAQ_States."Verify Hardware", s=w208, f=DAQ_States."Wait for Init" ("States")) -> (s? t:f=w209:T43)
          }
          frame "Verify Hardware" {
            n34 = call "DeviceListCheck.vi"("Device List"=string[] ["9481_1", "9435_1", "9435_2", "9401_1", "9269_1"], "Error In"=w239) -> ("Devices Present?"=w229:bool, "Report Text"=w232:string, "Error Out"=w231:errorcluster)  [unwired: 11 in]
            n35 = case shown="True" w229 {
              selector: w229 -> [w250 _]
              tunnel: w231 -> [w252 w253]
              tunnel: [w251 w253] -> w230
              frame False {
                n36 = property on="Turn On DAQ" class="Bool (strict)"(error in=w252, "Value"=w250) -> (error out=w251:errorcluster)  [unwired: 1 in, 1 out]
              }
              frame True {
              }
            }
            n37 = Select(t=DAQ_States."Initialize" ("f"), s=w229, f=DAQ_States."Wait for Init") -> (s? t:f=w236:T43)
          }
          frame "Initialize" {
            w259 = 4 items=["verify"=2, "reserve"=4, "commit"=3, "unreserve"=5, "abort"=6] ("action")
            w278 = 10123 items=["Finite Samples"=10178, "Continuous Samples"=10123, "Hardware Timed Single Point"=12522] ("sample mode")
            w281 = 4 items=["verify"=2, "reserve"=4, "commit"=3, "unreserve"=5, "abort"=6] ("action")
            w318 = 4 items=["verify"=2, "reserve"=4, "commit"=3, "unreserve"=5, "abort"=6] ("action")
            w319 = 4 items=["verify"=2, "reserve"=4, "commit"=3, "unreserve"=5, "abort"=6] ("action")
            w333 = 10123 items=["Finite Samples"=10178, "Continuous Samples"=10123, "Hardware Timed Single Point"=12522] ("sample mode")
            w343 = 0 items=["one channel for each line", "one channel for all lines"] ("line grouping")
            w349 = 0 items=["one channel for each line", "one channel for all lines"] ("line grouping")
            w352 = 0.0  # minimum value
            w353 = 5.0  # maximum value
            # "Hall Sensor"
            # "Motor TRIAC CCW"
            # "Motor TRIAC CW"
            # "Relay Controls"
            # "TRIAC Outputs"
            # "AO for ADC"
            n38 = call <vilib>:"DAQmx Create Task.vi"("auto cleanup"=TRUE, "error in"=w306) -> ("task out"=w304:refnum<k21>, "error out"=w305:errorcluster)  [unwired: 12 in]
            n39 = call <vilib>:"DAQmx Create Task.vi"("auto cleanup"=TRUE, "error in"=w270) -> ("task out"=w277:refnum<k21>, "error out"=w276:errorcluster)  [unwired: 12 in]
            n40 = call <vilib>:"DAQmx Create Task.vi"("auto cleanup"=TRUE, "error in"=w317) -> ("task out"=w314:refnum<k21>, "error out"=w315:errorcluster)  [unwired: 12 in]
            n41 = call <vilib>:"DAQmx Create Task.vi"("auto cleanup"=TRUE, "error in"=w313) -> ("task out"=w311:refnum<k21>, "error out"=w312:errorcluster)  [unwired: 12 in]
            n42 = call-poly <vilib>:"DAQmx Create Virtual Channel.vi"("task in"=w304, "frequency"=w254, "duty cycle"=w338, "counter"=tag "9401_1/ctr2", "error in"=w305) -> ("task out"=w308:refnum<k21>, "error out"=w339:errorcluster)  [unwired: 9 in]
            n43 = call-poly <vilib>:"DAQmx Create Virtual Channel.vi"("task in"=w314, "counter"=tag "9401_1/ctr0", "error in"=w315) -> ("task out"=w328:refnum<k21>, "error out"=w324:errorcluster)  [unwired: 11 in]
            n44 = call-poly <vilib>:"DAQmx Create Virtual Channel.vi"("task in"=w311, "counter"=tag "9401_1/ctr1", "error in"=w312) -> ("task out"=w327:refnum<k21>, "error out"=w326:errorcluster)  [unwired: 11 in]
            n45 = call-poly <vilib>:"DAQmx Create Virtual Channel.vi"("task in"=w277, "lines"=tag "9401_1/port0/line2", "error in"=w276) -> ("task out"=w283:refnum<k21>, "error out"=w284:errorcluster)  [unwired: 11 in]
            n46 = property class="DAQmx Channel"(reference=w308, error in=w339, "CO.Pulse.Term"=tag "/9401_1/PFI4") -> (reference out=w335:refnum<k21>, error out=w334:errorcluster)
            n47 = call-poly <vilib>:"DAQmx Create Virtual Channel.vi"("lines"=tag "9481_1/port0/line3", "error in"=w268) -> ("task out"=w267:refnum<k21>, "error out"=w266:errorcluster)  [unwired: 12 in]
            n48 = property class="DAQmx Channel"(reference=w328, error in=w324, "CI.CountEdges.Term"=tag "/9401_1/PFI0") -> (reference out=w323:refnum<k21>, error out=w322:errorcluster)
            n49 = property class="DAQmx Channel"(reference=w327, error in=w326, "CI.CountEdges.Term"=tag "/9401_1/PFI1") -> (reference out=w321:refnum<k21>, error out=w320:errorcluster)
            n50 = call-poly <vilib>:"DAQmx Create Virtual Channel.vi"("lines"=tag "9481_1/port0/line0:2", "name to assign"="Relay Outputs", "line grouping"=w349, "error in"=w347) -> ("task out"=w346:refnum<k21>, "error out"=w345:errorcluster)  [unwired: 10 in]
            n51 = call-poly <vilib>:"DAQmx Create Virtual Channel.vi"("lines"=tag "9435_1/port0/line0:2, 9435_2/port0/line0:3", "name to assign"="Outputs", "line grouping"=w343, "error in"=w342) -> ("task out"=w340:refnum<k21>, "error out"=w341:errorcluster)  [unwired: 10 in]
            n52 = call-poly <vilib>:"DAQmx Create Virtual Channel.vi"("maximum value"=w353, "minimum value"=w352, "physical channels"=tag "9269_1/ao0:2" ("lines"), "name to assign"="AO for ADC", "error in"=w289) -> ("task out"=w351:refnum<k21>, "error out"=w350:errorcluster)  [unwired: 9 in]
            n53 = call-poly <vilib>:"DAQmx Timing.vi"("task/channels in"=w283, "sample mode"=w278, "rate"=1000.0, "error in"=w284) -> ("task out"=w279:refnum<k21>, "error out"=w280:errorcluster)  [unwired: 10 in]
            n54 = call-poly <vilib>:"DAQmx Timing.vi"("task/channels in"=w335, "sample mode"=w333, "error in"=w334) -> ("task out"=w258:refnum<k21>, "error out"=w255:errorcluster)  [unwired: 11 in]
            n55 = call <vilib>:"DAQmx Control Task.vi"("task/channels in"=w323, "action"=w318, "error in"=w322) -> ("task out"=w293:refnum<k21>, "error out"=w296:errorcluster)  [unwired: 11 in]
            n56 = call <vilib>:"DAQmx Control Task.vi"("task/channels in"=w321, "action"=w319, "error in"=w320) -> ("task out"=w301:refnum<k21>, "error out"=w299:errorcluster)  [unwired: 11 in]
            n57 = call <vilib>:"DAQmx Control Task.vi"("task/channels in"=w258, "action"=w259, "error in"=w255) -> ("task out"=w257:refnum<k21>, "error out"=w256:errorcluster)  [unwired: 11 in]
            n58 = call <vilib>:"DAQmx Control Task.vi"("task/channels in"=w279, "action"=w281, "error in"=w280) -> ("task out"=w272:refnum<k21>, "error out"=w273:errorcluster)  [unwired: 11 in]
            n59 = flat-sequence {
              tunnel: w257 -> [w357]
              tunnel: w256 -> [w356]
              tunnel: w301 -> [w365]
              tunnel: [w365] -> w300
              tunnel: w299 -> [w364]
              tunnel: [w364] -> w298
              tunnel: w296 -> [w363]
              tunnel: [w363] -> w295
              tunnel: w293 -> [w362]
              tunnel: [w362] -> w292
              tunnel: w273 -> [w360]
              tunnel: w272 -> [w361]
              tunnel: [w359] -> w263
              tunnel: [w358] -> w262
              tunnel: [w357] -> w261
              tunnel: [w356] -> w260
              tunnel: [w369] -> w336
              tunnel: [w368] -> w337
              tunnel: [w379] -> w302
              tunnel: w300 -> [w378]
              tunnel: w298 -> [w377]
              tunnel: [w376] -> w297
              tunnel: w295 -> [w375]
              tunnel: [w374] -> w294
              tunnel: w292 -> [w373]
              tunnel: [w372] -> w291
              tunnel: [w371] -> w274
              tunnel: [w370] -> w271
              tunnel: w263 -> [w371]
              tunnel: w262 -> [w370]
              tunnel: w261 -> [w367]
              tunnel: w260 -> [w366]
              frame #0 {
                n60 = call <vilib>:"DAQmx Start Task.vi"("task/channels in"=w361, "error in"=w360) -> ("task out"=w358:refnum<k21>, "error out"=w359:errorcluster)  [unwired: 12 in]
              }
              frame #1 {
                n61 = call <vilib>:"DAQmx Start Task.vi"("task/channels in"=w373, "error in"=w375) -> ("task out"=w372:refnum<k21>, "error out"=w374:errorcluster)  [unwired: 12 in]
                n62 = call <vilib>:"DAQmx Start Task.vi"("task/channels in"=w378, "error in"=w377) -> ("task out"=w379:refnum<k21>, "error out"=w376:errorcluster)  [unwired: 12 in]
                n63 = call <vilib>:"DAQmx Start Task.vi"("task/channels in"=w367, "error in"=w366) -> ("task out"=w368:refnum<k21>, "error out"=w369:errorcluster)  [unwired: 12 in]
              }
            }
          }
          frame "Run" {
            # "Is the task stopped?"
            # "Hall Sensor"
            # "Motor TRIAC CCW"
            # "Motor TRIAC CW"
            # "AO for ADC"
            # "Relay Controls"
            # "TRIAC Outputs"
            n64 = case shown="True" w388 {
              tunnel: w396 -> [w495 w499]
              tunnel: w395 -> [w494 w500]
              tunnel: [w495 w498] -> w393
              tunnel: [w494 w497] -> w394
              tunnel: w392 -> [w493 _]
              tunnel: [w493 TRUE] -> w385
              frame False {
              }
              frame True {
                n65 = call <vilib>:"DAQmx Stop Task.vi"("task/channels in"=w499, "error in"=w500) -> ("task out"=w498:refnum<k21>, "error out"=w497:errorcluster)  [unwired: 12 in]
              }
            }
            n66 = call-poly <vilib>:"DAQmx Read.vi"("task/channels in"=w406, "number of samples per channel"=-1, "timeout"=10.0, "error in"=w407) -> ("task out"=w404:refnum<k21>, "data"=w411:u8[], "error out"=w405:errorcluster)  [unwired: 9 in]
            n67 = Compound Arithmetic op=AND(w385, invert w388) -> (w387:bool)
            n68 = case shown="True" w387 {
              tunnel: w394 -> [w485 w489]
              tunnel: w393 -> [w486 w488]
              tunnel: [w486 w492] -> w391
              tunnel: [w485 w491] -> w390
              tunnel: w385 -> [w484 _]
              tunnel: [w484 FALSE] -> w384
              frame False {
              }
              frame True {
                n69 = call <vilib>:"DAQmx Start Task.vi"("task/channels in"=w488, "error in"=w489) -> ("task out"=w492:refnum<k21>, "error out"=w491:errorcluster)  [unwired: 12 in]
                n70 = Wait (ms)(milliseconds to wait=u32 1200) -> ()  [unwired: 1 out]
              }
            }
            n71 = Build Array("AC Power", "Mode Shift FB", "Lid Status") -> (w453:bool[])
            n72 = Build Array("Pressure", "Motor Current", "Temperature") -> (w449:dbl[])
            n73 = Search 1D Array(1D array=w411, element=u8 4) -> (index of element=w409:i32)  [unwired: 1 in]
            n74 = Equal?(x=w409, y=-1) -> (x = y?=w397:bool)
            n75 = Compound Arithmetic op=OR(w388, w389) -> (w386:bool)
            n76 = call-poly <vilib>:"DAQmx Read.vi"("task/channels in"=w461, "error in"=w447) -> ("task out"=w460:refnum<k21>, "data"=w459:bool[], "error out"=w458:errorcluster)  [unwired: 11 in]
            n77 = call-poly <vilib>:"DAQmx Write.vi"("task/channels in"=w457, "data"=w453, "error in"=w446) -> ("task out"=w452:refnum<k21>, "error out"=w443:errorcluster)  [unwired: 10 in, 1 out]
            n78 = call-poly <vilib>:"DAQmx Write.vi"("task/channels in"=w451, "data"=w449, "error in"=w445) -> ("task out"=w448:refnum<k21>, "error out"=w444:errorcluster)  [unwired: 10 in, 1 out]
            n79 = call-poly <vilib>:"DAQmx Read.vi"("task/channels in"=w425, "error in"=w427) -> ("task out"=w424:refnum<k21>, "data"=w422:u32, "error out"=w426:errorcluster)  [unwired: 11 in]
            "CW" <- w422
            n80 = call-poly <vilib>:"DAQmx Read.vi"("task/channels in"=w428, "error in"=w431) -> ("task out"=w430:refnum<k21>, "data"=w421:u32, "error out"=w429:errorcluster)  [unwired: 11 in]
            "CCW" <- w421
            n81 = case shown="True" "LL (M - A)" {
              tunnel: [w463 w474] -> w403
              tunnel: [w464 w473] -> w402
              tunnel: w401 -> [w466 w472]
              tunnel: w400 -> [w467 w471]
              tunnel: w399 -> [w462 w470]
              tunnel: [w462 w469] -> w398
              tunnel: w397 -> [_ w468]
              tunnel: "Lid Lock Feedback" -> [w465 _]
              frame False {
                n82 = call-poly <vilib>:"DAQmx Write.vi"("task/channels in"=w466, "data"=w465, "error in"=w467) -> ("task out"=w464:refnum<k21>, "error out"=w463:errorcluster)  [unwired: 10 in, 1 out]
              }
              frame True {
                # "Automatic Lid Lock feedback"
                n83 = case shown="False" w468 {
                  tunnel: w472 -> [w480 w483]
                  tunnel: w470 -> [w475 w481]
                  tunnel: [w479 w482] -> w474
                  tunnel: [w478 w483] -> w473
                  tunnel: w471 -> [w477 w482]
                  tunnel: [w476 w481] -> w469
                  frame False {
                    n84 = Not(x=w475) -> (.not. x?=w476:bool)
                    n85 = call-poly <vilib>:"DAQmx Write.vi"("task/channels in"=w480, "data"=w476, "error in"=w477) -> ("task out"=w478:refnum<k21>, "error out"=w479:errorcluster)  [unwired: 10 in, 1 out]
                  }
                  frame True {
                  }
                }
              }
            }
            n86 = Index Array(array=w459) -> (element #1=w438:bool, element #2=w432:bool, element #3=w437:bool, element #4=w436:bool, element #5=w435:bool, element #6=w434:bool, element #7=w433:bool)  [unwired: 7 in]
            n87 = call "Counts to Triac Direction.vi"("CCW ctr"=w421, "CW ctr"=w422) -> ("CW"=w419:bool, "CCW"=w423:bool)  [unwired: 8 in]
            n88 = case shown="False" w386 {
              tunnel: w391 -> [w506 w508]
              tunnel: w390 -> [w505 w507]
              tunnel: [w504 w508] -> w441
              tunnel: [w503 w507] -> w440
              tunnel: w383 -> [w502 _]
              tunnel: w382 -> [w501 _]
              frame False {
                n89 = property class="DAQmx Channel"(reference=w506, error in=w505, "CO.Pulse.Freq"=w501, "CO.Pulse.DutyCyc"=w502) -> (reference out=w504:refnum<k21>, error out=w503:errorcluster)
              }
              frame True {
              }
            }
            n90 = Select(t=DAQ_States."Run" ("States"), s=w415, f=DAQ_States."Shutdown" ("States")) -> (s? t:f=w414:T43)
          }
          frame "Shutdown" {
            w524 = 0.0
            w520 = FALSE ("element")
            # "Hall Sensor"
            # "Motor TRIAC CCW"
            # "Motor TRIAC CW"
            # "Relay Controls"
            # "TRIAC Outputs"
            # "AO for ADC"
            n91 = local read "AC Power"() -> (w522:bool)
            n92 = Build Array(w522, w520, w520) -> (w558:bool[])
            n93 = Build Array(w524, w524, w524) -> (w523:dbl[])
            n94 = call-poly <vilib>:"DAQmx Write.vi"("task/channels in"=w557, "data"=w558, "error in"=w556) -> ("task out"=w548:refnum<k21>, "error out"=w550:errorcluster)  [unwired: 10 in, 1 out]
            n95 = call-poly <vilib>:"DAQmx Write.vi"("task/channels in"=w513, "data"=FALSE, "error in"=w514) -> ("task out"=w512:refnum<k21>, "error out"=w511:errorcluster)  [unwired: 10 in, 1 out]
            n96 = call-poly <vilib>:"DAQmx Write.vi"("task/channels in"=w552, "data"=w523, "error in"=w553) -> ("task out"=w555:refnum<k21>, "error out"=w554:errorcluster)  [unwired: 10 in, 1 out]
            n97 = call "Time Delay"("error in (no error)"=w550, "Delay Time (s)"=2.0) -> ("error out"=w541:errorcluster)  [unwired: 9 in]
            n98 = call <vilib>:"DAQmx Clear Task.vi"("task in"=w519, "error in"=w518) -> ("error out"=w517:errorcluster)  [unwired: 13 in]
            n99 = call <vilib>:"DAQmx Clear Task.vi"("task in"=w566, "error in"=w567) -> ("error out"=w565:errorcluster)  [unwired: 13 in]
            n100 = call <vilib>:"DAQmx Clear Task.vi"("task in"=w548, "error in"=w541) -> ("error out"=w544:errorcluster)  [unwired: 13 in]
            n101 = call <vilib>:"DAQmx Clear Task.vi"("task in"=w555, "error in"=w554) -> ("error out"=w530:errorcluster)  [unwired: 13 in]
            n102 = call <vilib>:"DAQmx Clear Task.vi"("task in"=w526, "error in"=w527) -> ("error out"=w525:errorcluster)  [unwired: 13 in]
            n103 = call <vilib>:"DAQmx Clear Task.vi"("task in"=w560, "error in"=w561) -> ("error out"=w528:errorcluster)  [unwired: 13 in]
            n104 = call <vilib>:"DAQmx Clear Task.vi"("task in"=w563, "error in"=w562) -> ("error out"=w546:errorcluster)  [unwired: 13 in]
            n105 = call <vilib>:"DAQmx Clear Task.vi"("task in"=w512, "error in"=w511) -> ("error out"=w516:errorcluster)  [unwired: 13 in]
            n106 = property on="Motor Current" class="Slide (strict)"(error in=w530, "Value"=0.0 ("Motor Current")) -> (error out=w532:errorcluster)  [unwired: 1 in, 1 out]
            n107 = property on="Turn On DAQ" class="Bool (strict)"(error in=w544, "Value"=FALSE ("Turn On DAQ")) -> (error out=w543:errorcluster)  [unwired: 1 in, 1 out]
            n108 = property on="Basket RPM" class="DigNum (strict)"(error in=w546, "Value"=10.0 ("Basket RPM")) -> (error out=w545:errorcluster)  [unwired: 1 in, 1 out]
            n109 = property on="AC Power" class="Bool (strict)"(error in=w543, "Value"=FALSE ("AC Power")) -> (error out=w538:errorcluster)  [unwired: 1 in, 1 out]
            n110 = property on="Temperature" class="Slide (strict)"(error in=w532, "Value"=0.0 ("Temperature")) -> (error out=w531:errorcluster)  [unwired: 1 in, 1 out]
            n111 = property on="Mode Shift FB" class="Bool (strict)"(error in=w538, "Value"=FALSE ("Mode Shift FB")) -> (error out=w537:errorcluster)  [unwired: 1 in, 1 out]
            n112 = property on="Pressure" class="Slide (strict)"(error in=w531, "Value"=0.0 ("Pressure")) -> (error out=w529:errorcluster)  [unwired: 1 in, 1 out]
            n113 = property on="Lid Status" class="Bool (strict)"(error in=w537, "Value"=FALSE ("Lid Status")) -> (error out=w536:errorcluster)  [unwired: 1 in, 1 out]
          }
          frame "Exit" {
            n114 = case shown="True" w596 {
              tunnel: w599 -> [w607 w631]
              tunnel: w598 -> [_ w630]
              tunnel: w597 -> [_ w629]
              tunnel: w578 -> [w606 w628]
              tunnel: w595 -> [w605 w627]
              tunnel: w594 -> [w604 w626]
              tunnel: w593 -> [w603 w625]
              tunnel: w592 -> [_ w624]
              tunnel: [w603 w623] -> w591
              tunnel: [w604 w622] -> w590
              tunnel: [w605 w621] -> w589
              tunnel: [w606 w620] -> w588
              tunnel: [w607 w619] -> w587
              tunnel: w583 -> [_ w618]
              tunnel: w582 -> [_ w617]
              tunnel: w581 -> [w602 w616]
              tunnel: w580 -> [_ w615]
              tunnel: [w602 w614] -> w579
              tunnel: w576 -> [_ w613]
              tunnel: w575 -> [w601 w612]
              tunnel: [w601 w611] -> w574
              tunnel: w573 -> [_ w610]
              tunnel: w572 -> [w600 w609]
              tunnel: [w600 w608] -> w571
              frame False {
              }
              frame True {
                # "Hall Sensor"
                # "Motor TRIAC CCW"
                # "Motor TRIAC CW"
                # "Relay Controls"
                # "TRIAC Outputs"
                # "AO for ADC"
                n115 = call <vilib>:"DAQmx Clear Task.vi"("task in"=w613, "error in"=w612) -> ("error out"=w611:errorcluster)  [unwired: 13 in]
                n116 = call <vilib>:"DAQmx Clear Task.vi"("task in"=w610, "error in"=w609) -> ("error out"=w608:errorcluster)  [unwired: 13 in]
                n117 = call <vilib>:"DAQmx Clear Task.vi"("task in"=w630, "error in"=w631) -> ("error out"=w619:errorcluster)  [unwired: 13 in]
                n118 = call <vilib>:"DAQmx Clear Task.vi"("task in"=w629, "error in"=w628) -> ("error out"=w620:errorcluster)  [unwired: 13 in]
                n119 = call <vilib>:"DAQmx Clear Task.vi"("task in"=w618, "error in"=w627) -> ("error out"=w621:errorcluster)  [unwired: 13 in]
                n120 = call <vilib>:"DAQmx Clear Task.vi"("task in"=w615, "error in"=w616) -> ("error out"=w614:errorcluster)  [unwired: 13 in]
                n121 = call <vilib>:"DAQmx Clear Task.vi"("task in"=w617, "error in"=w626) -> ("error out"=w622:errorcluster)  [unwired: 13 in]
                n122 = call <vilib>:"DAQmx Clear Task.vi"("task in"=w624, "error in"=w625) -> ("error out"=w623:errorcluster)  [unwired: 13 in]
              }
            }
          }
        }
        "DAQ On?" <- w125
        "Cold Valve" <- w149
        "Drain Pump" <- w151
        "Mode Shift" <- w129
        "Recirc Pump" <- w150
        "Hot Valve" <- w148
        "Spray/Rinse Valve" <- w147
        "Fabric SoftValve" <- w146
        "Triac CW" <- w136
        "Traic CCW" <- w135
        "DAQ Status" <- w128
        n123 = case shown="True" "MS (M - A)" {
          tunnel: w143 -> [w177 w188]
          tunnel: [w177 w187] -> w142
          tunnel: w129 -> [_ w178]
          frame False {
          }
          frame True {
            n124 = Equal?(x=w178, y=TRUE) -> (x = y?=w185:bool)
            n125 = case shown="False" w185 {
              tunnel: w188 -> [w193 w195]
              tunnel: [w193 w194] -> w180
              frame False {
              }
              frame True {
                n126 = Increment(x=w195) -> (x+1=w194:dbl)
              }
            }
            "Counter" <- w180
            n127 = In Range and Coerce(upper limit=24.0, x=w180, lower limit=15.0) -> (In Range?=w182:bool)  [unwired: 1 out]
            n128 = case shown="False" w182 {
              frame False {
                n129 = property on="Mode Shift FB" class="Bool (strict)"("Value"=FALSE ("Mode Shift FB")) -> ()  [unwired: 2 in, 2 out]
              }
              frame True {
                n130 = property on="Mode Shift FB" class="Bool (strict)"("Value"=TRUE ("Mode Shift FB")) -> ()  [unwired: 2 in, 2 out]
              }
            }
            n131 = Greater Or Equal?(x=w180, y=24.0) -> (x >= y?=w179:bool)
            n132 = case shown="False" w179 {
              tunnel: w180 -> [w189 _]
              tunnel: [w189 0.0] -> w187
              frame False {
              }
              frame True {
              }
            }
          }
        }
        n133 = case shown="False" w133 {
          tunnel: w132 -> [w197 _]
          tunnel: [w196 0.0] -> w134
          frame False {
            n134 = Increment(x=w197) -> (x+1=w196:dbl)
          }
          frame True {
          }
        }
        n135 = Merge Errors(w159, w158, w157, w141, w140, w139, w122, w119) -> (w155:errorcluster)
        n136 = call "Error_Control.vi"("Error In"=w155) -> ("Error Out"=w154:errorcluster)  [unwired: 14 in]
      }
    }
    frame Enabled {
    }
  }
  n137 = call "GEA2 Write ERD.vi"("GEA2 Reference In"=w15, "GEA Inputs"="GEA Inputs", "Write ERD List"=T40[] [{"ERD Number"=61461, "Data Type"=enum."string", "Data"="01"}], "Error In"=w12, "Verify ERD Response?"=FALSE) -> ("GEA2 Reference Out"=w14:refnum<k24>, "Error Out"=w11:errorcluster)  [unwired: 8 in, 1 out]
  n138 = Create User Event(user event datatype=w42, error in=w12) -> (user event=w39:refnum<user-event>, error out=w41:errorcluster)
  n139 = call <vilib>:"Add State(s) to Queue__jki_lib_state_machine.vi"("State(s) in (\"\")"="Macro: Initialize") -> ("States Out"=w28:string)  [unwired: 14 in]
  n140 = local read "Disable Write"() -> (w2:bool)
  n141 = call "HEUI_Event_FGV.vi"("Event In"=w39, "Action"=enum16{"Get", "Set"}."Set", "Error In"=w41) -> ("Event Out"=w37:refnum<user-event>, "Error Out"=w40:errorcluster)  [unwired: 11 in]
  n142 = Unbundle By Name(T44 {"Data"=variant, "State"=enum."Run"} ("Data")) -> ("State"=w63:enum16{"Run", "Shutdown"})
  n143 = disable-structure shown="Disabled" {
    disable-tunnel: [w637 _] -> w48
    disable-tunnel: w45 -> [w635 _]
    disable-tunnel: w15 -> [w634 _]
    disable-tunnel: [w633 _] -> w44
    disable-tunnel: w12 -> [w632 _]
    frame Disabled {
      n144 = while "Continuous Send Loop" {
        shift-right: [w654] -> _
        shift-left: w634 -> [w655]
        shift-right: [w649] -> _
        shift-left: Cont_Send_States."Run" ("State") -> [w648]
        tunnel: w635 -> [w650]
        tunnel: [w642] -> w637
        shift-right: [w639] -> w633
        shift-left: w632 -> [w653]
        stop <- w651 stop-if-true
        n145 = Dequeue Element(queue=w650, timeout in ms (-1)=10, error in (no error)=w653) -> (queue out=w643:refnum<queue>, element=w646:T42, timed out?=w644:bool, error out=w652:errorcluster)
        n146 = property on="GEA2 Send" class="Clust (strict)"() -> ("Value"=w638:T54)  [unwired: 2 in, 2 out]
        n147 = Select(t=w648, s=w644, f=w646) -> (s? t:f=w647:T42)
        n148 = case shown="\"Run\", Default" w647 {
          selector: w647 -> [w658 w676]
          tunnel: w652 -> [w663 w679]
          tunnel: w655 -> [w662 w678]
          tunnel: [w661 w678] -> w654
          tunnel: [w660 w679] -> w640
          tunnel: [_ TRUE] -> w651
          tunnel: [w658 w676] -> w649
          tunnel: w643 -> [w657 w675]
          tunnel: [w657 w675] -> w642
          tunnel: w638 -> [w656 _]
          frame "Run", Default {
            n149 = case shown="True" "Start Send" {
              tunnel: w663 -> [w665 w673]
              tunnel: w662 -> [w664 w670]
              tunnel: [w664 w669] -> w661
              tunnel: [w665 w668] -> w660
              tunnel: w656 -> [_ w666]
              frame False {
              }
              frame True {
                n150 = call "GEA2MessageFormatter.vi"("Prefix(Send/Recv)"="SEND", "GEA2 Data In"=w666, "Error In"=w673) -> ("Output String"=w667:string, "Error Out"=w674:errorcluster)  [unwired: 11 in]
                n151 = call "GExplorer_Queue_GEA2.vi"("Output String"=w667, "error in (no error)"=w674) -> ("error out"=w671:errorcluster)  [unwired: 13 in]
                n152 = call "GEA2 Send Message.vi"("GEA2 Reference In"=w670, "Input Data"=w666, "Error In"=w671) -> ("GEA2 Reference Out"=w669:refnum<k24>, "Error Out"=w668:errorcluster)  [unwired: 11 in]
              }
            }
          }
          frame "Shutdown" {
          }
        }
        n153 = call "Error_Control.vi"("Error In"=w640) -> ("Error Out"=w639:errorcluster)  [unwired: 14 in]
        n154 = Wait (ms)(milliseconds to wait="Msg Rate (ms)") -> ()  [unwired: 1 out]
      }
    }
    frame Enabled {
    }
  }
  n155 = while "UI Loop" {
    shift-right: [w681] -> w18
    shift-left: w40 -> [w687]
    tunnel: w68 -> [w686]
    tunnel: w37 -> [w684]
    tunnel: w3 -> [w683]
    tunnel: "GEA Inputs" -> [w682]
    i -> [w680]
    stop <- w685 stop-if-true
    n156 = event shown="[55] \"Stop\": Value Change" {
      selector: w686 -> [_ _ _ _ _ _ _ _ _ _ _ _ _ _ _ _ _ _ _ _ _ _ _ _ _ _ _ _ _ _ _ _ _ _ _ _ _ _ _ _ _ _ _ _ _ _ _ _ _ _ _ _ _ _ _ _]
      dyn-events: _ -> [_ _ _ _ _ _ _ _ _ _ _ _ _ _ _ _ _ _ _ _ _ _ _ _ _ _ _ _ _ _ _ _ _ _ _ _ _ _ _ _ _ _ _ _ _ _ _ _ _ _ _ _ _ _ _ _]
      timeout: _ -> [_ _ _ _ _ _ _ _ _ _ _ _ _ _ _ _ _ _ _ _ _ _ _ _ _ _ _ _ _ _ _ _ _ _ _ _ _ _ _ _ _ _ _ _ _ _ _ _ _ _ _ _ _ _ _ _]
      tunnel: [w688 w689 w705 w713 w760 w764 w769 w805 w821 w833 w855 w873 w891 w917 w942 w967 w991 w1013 w1016 w1072 w1085 w1150 w1172 w1196 w1213 w1232 w1254 w1275 w1295 w1315 w1335 w1377 w1386 w1437 w1472 w1493 w1513 w1533 w1565 w1583 w1605 w1623 w1649 w1674 w1700 w1725 w1749 w1800 w1805 w1808 w1856 w1900 w1920 w1939 w1955 w1977] -> w681
      tunnel: w687 -> [w688 w693 w706 w717 w763 w767 w775 w810 w831 w838 w858 w877 w896 w921 w946 w971 w995 w1013 w1021 w1076 w1089 w1155 w1175 w1193 w1218 w1238 w1259 w1280 w1301 w1320 w1340 w1368 w1387 w1442 w1478 w1496 w1519 w1538 w1570 w1589 w1609 w1629 w1655 w1679 w1704 w1729 w1754 w1802 w1806 w1814 w1862 w1906 w1926 w1945 w1961 w1978]
      tunnel: [_ _ _ _ _ _ _ _ _ _ _ _ _ _ _ _ _ TRUE _ _ _ _ _ _ _ _ _ _ _ _ _ _ _ _ _ _ _ _ _ _ _ _ _ _ _ _ _ _ _ _ _ _ _ _ _ TRUE] -> w685
      tunnel: w682 -> [_ _ w702 _ _ _ _ _ _ w832 w851 w870 w889 w914 w939 w964 w989 _ _ _ w1083 w1148 w1169 w1189 w1210 w1231 w1252 w1273 w1293 w1313 w1333 w1360 _ w1435 w1471 w1491 w1511 w1531 w1573 w1594 w1602 w1622 w1647 w1672 w1697 w1722 w1747 w1798 _ w1807 w1855 w1899 w1919 w1938 w1954 _]
      tunnel: w684 -> [_ _ _ _ _ _ _ _ _ _ _ _ _ _ _ _ _ _ w1025 _ _ _ _ _ _ _ _ _ _ _ _ _ _ _ _ _ _ _ _ _ _ _ _ _ _ _ _ _ _ _ _ _ _ _ _ _]
      tunnel: w683 -> [_ w695 w703 w718 _ _ w773 w807 _ w839 w852 w875 w894 w919 w944 w969 _ _ w1019 _ w1090 w1153 _ w1191 w1217 w1237 w1258 w1278 w1298 w1318 w1338 w1365 _ w1440 w1476 w1497 w1516 w1536 w1568 w1587 w1603 w1627 w1652 w1677 w1698 w1723 w1751 w1801 _ w1812 w1860 w1905 w1925 w1944 w1960 _]
      event Timeout {
        n157 = event-data() -> ()  [unwired: 1 in, 3 out]
      }
      event "Send Button": Value Change {
        n158 = event-data() -> ()  [unwired: 1 in, 6 out]
        n159 = call "GEA2 Initialize.vi"("Board Index"=w695, "Source Address"=u8 228, "error in"=w693) -> ("GeaCommunication.GeaBus"=w694:refnum<k24>, "error out"=w692:errorcluster)  [unwired: 10 in, 1 out]
        n160 = call "GEA2MessageFormatter.vi"("Prefix(Send/Recv)"="SEND", "GEA2 Data In"="GEA2 Send", "Error In"=w692) -> ("Output String"=w698:string, "Error Out"=w701:errorcluster)  [unwired: 11 in]
        n161 = call "GExplorer_Queue_GEA2.vi"("Output String"=w698, "error in (no error)"=w701) -> ("error out"=w699:errorcluster)  [unwired: 13 in]
        n162 = call "GEA2 Send Message.vi"("GEA2 Reference In"=w694, "Input Data"="GEA2 Send", "Error In"=w699) -> ("GEA2 Reference Out"=w691:refnum<k24>, "Error Out"=w690:errorcluster)  [unwired: 11 in]
        n163 = call "GEA2 Stop.vi"("GEA2 Reference In"=w691, "Error In"=w690) -> ("Error Out"=w689:errorcluster)  [unwired: 13 in]
      }
      event "Low Power OFF": Value Change {
        n164 = event-data() -> ()  [unwired: 1 in, 6 out]
        n165 = call "GEA2 Initialize.vi"("Board Index"=w703, "Source Address"=u8 228, "error in"=w706) -> ("GeaCommunication.GeaBus"=w709:refnum<k24>, "error out"=w708:errorcluster)  [unwired: 10 in, 1 out]
        n166 = call "GEA2 Write ERD.vi"("GEA2 Reference In"=w709, "GEA Inputs"=w702, "Write ERD List"=T40[] [{"ERD Number"=61461, "Data Type"=enum."string", "Data"="01"}], "Error In"=w708) -> ("GEA2 Reference Out"=w704:refnum<k24>, "Error Out"=w711:errorcluster)  [unwired: 9 in, 1 out]
        n167 = call "GEA2 Stop.vi"("GEA2 Reference In"=w704, "Error In"=w711) -> ("Error Out"=w705:errorcluster)  [unwired: 13 in]
      }
      event "Script": Value Change {
        w736 = T38 {"Overall Script File Progress"=0.0, "Current Script Progress"=0.0, "Script"="", "Test"="", "Elapsed time (s)"=0.0, "Done?"=FALSE}  # Script Info
        w726 = T10 {"Source"=228, "Destination"=35, "Command"=1, "Message"=""}  # Version Query (for log header)
        n168 = event-data() -> ()  [unwired: 1 in, 1 out]
        n169 = call "GEA2 Initialize.vi"("Board Index"=w718, "Source Address"=u8 228, "error in"=w717) -> ("GeaCommunication.GeaBus"=w715:refnum<k24>, "error out"=w716:errorcluster)  [unwired: 10 in, 1 out]
        n170 = Obtain Queue(name (unnamed)="Script_Stop", element data type=FALSE, error in (no error)=w716) -> (queue out=w732:refnum<queue>, error out=w735:errorcluster)  [unwired: 2 in, 1 out]
        n171 = Obtain Queue(name (unnamed)="Script_Info", element data type=w736, error in (no error)=w735) -> (queue out=w738:refnum<queue>, error out=w729:errorcluster)  [unwired: 2 in, 1 out]
        n172 = while {
          tunnel: w738 -> [w750]
          shift-right: [w742] -> w721
          shift-left: w729 -> [w745]
          tunnel: [w749] -> w737
          tunnel: w732 -> [w746]
          tunnel: [w741] -> w730
          stop <- w747 stop-if-true
          n173 = Dequeue Element(queue=w750, error in (no error)=w745) -> (queue out=w749:refnum<queue>, element=w748:T38, error out=w744:errorcluster)  [unwired: 1 in, 1 out]
          "Script Info" <- w748
          n174 = Unbundle By Name(w748) -> ("Done?"=w747:bool)
          n175 = case shown="False" "stop" {
            selector: "stop" -> [_ w753]
            tunnel: w746 -> [w752 w757]
            tunnel: w745 -> [w751 w756]
            tunnel: [w751 w755] -> w743
            tunnel: [w752 w754] -> w741
            frame False {
            }
            frame True {
              n176 = Enqueue Element(queue=w757, element=w753, error in (no error)=w756) -> (queue out=w754:refnum<queue>, error out=w755:errorcluster)  [unwired: 1 in, 1 out]
            }
          }
          n177 = Merge Errors(w743, w744) -> (w742:errorcluster)
        }
        n178 = call "GEA2 Script Test SLB.vi"("GEA2 Reference In"=w715, "Version Query (for log header)"=w726, "Enqueue Sends?"=TRUE, "Standalone"=FALSE, "Script path"="Script Path", "Log File Path (empty for prompt)"="Script Log Path", "Error In"=w729) -> ("GEA2 Reference Out"=w712:refnum<k24>, "Pass/Fail?"=→"Script Pass/Fail?":bool, "Report Text"=→"Script Report Text":string, "Error Out"=→"Script Error Out":errorcluster)  [unwired: 5 in]
        n179 = Release Queue(queue=w737, error in (no error)=w721) -> (error out=w731:errorcluster)  [unwired: 1 in, 2 out]
        n180 = Release Queue(queue=w730, error in (no error)=w731) -> (error out=w714:errorcluster)  [unwired: 1 in, 2 out]
        n181 = call "GEA2 Stop.vi"("GEA2 Reference In"=w712, "Error In"=w714) -> ("Error Out"=w713:errorcluster)  [unwired: 13 in]
      }
      event "Clear Button": Value Change {
        w758 = T46 {"Data"=variant, "State"=enum."Clear"} ("Data")
        n182 = event-data() -> ()  [unwired: 1 in, 6 out]
        n183 = Obtain Queue(name (unnamed)="GEA2", element data type=w758, error in (no error)=w763) -> (queue out=w759:refnum<queue>, error out=w761:errorcluster)  [unwired: 2 in, 1 out]
        n184 = Enqueue Element(queue=w759, element=w758, error in (no error)=w761) -> (error out=w760:errorcluster)  [unwired: 1 in, 2 out]
      }
      event "Save Log": Value Change {
        n185 = event-data() -> ()  [unwired: 1 in, 6 out]
        n186 = property on="GEA2 Msg Log" class="Str"(error in=w767) -> (error out=w766:errorcluster, "Value"=w765:string)  [unwired: 1 in, 1 out]
        n187 = Write to Text File(prompt (Choose or enter file path)="Choose filename and path to save txt file to ", text=w765, error in=w766) -> (error out=w764:errorcluster)  [unwired: 1 in, 2 out]
      }
      event "ADC Info Button": Value Change {
        w778 = u16 0 ("Motor Current ADC")
        w783 = 2 ("length (rest)")
        w800 = T10 {"Source"=228, "Destination"=35, "Command"=240, "Message"="03F309F204F203"}  # ADC ERD
        # "Ex. 03 50 09 02 DD 0F 40 04 02 E3 0F 40 03 02 E3 0F"
        n188 = event-data() -> ()  [unwired: 1 in, 6 out]
        n189 = call "GEA2 Initialize.vi"("Board Index"=w773, "Source Address"=u8 228, "error in"=w775) -> ("GeaCommunication.GeaBus"=w772:refnum<k24>, "error out"=w774:errorcluster)  [unwired: 10 in, 1 out]
        n190 = call "GEA2MessageFormatter.vi"("Prefix(Send/Recv)"="SEND", "GEA2 Data In"=w800, "Error In"=w774) -> ("Output String"=w799:string, "Error Out"=w802:errorcluster)  [unwired: 11 in]
        n191 = call "GExplorer_Queue_GEA2.vi"("Output String"=w799, "error in (no error)"=w802) -> ("error out"=w801:errorcluster)  [unwired: 13 in]
        n192 = call "GEA2 Send and Receive Message.vi"("GeaCommunication.GeaBus"=w772, "Input Data"=w800, "Error In"=w801) -> ("GeaCommunication.GeaBus"=w770:refnum<k24>, "Converted Data Out"=w798:T45, "Error Out"=w771:errorcluster)  [unwired: 9 in, 1 out]
        n193 = Unbundle By Name(w798) -> ("Message"=w782:string)
        n194 = String Subset(string=w782, offset (0)=12, length (rest)=w783) -> (substring=w792:string)
        n195 = String Subset(string=w782, offset (0)=15, length (rest)=w783) -> (substring=w791:string)
        n196 = String Subset(string=w782, offset (0)=27, length (rest)=w783) -> (substring=w789:string)
        n197 = String Subset(string=w782, offset (0)=30, length (rest)=w783) -> (substring=w786:string)
        n198 = String Subset(string=w782, offset (0)=42, length (rest)=w783) -> (substring=w780:string)
        n199 = String Subset(string=w782, offset (0)=45, length (rest)=w783) -> (substring=w781:string)
        n200 = Concatenate Strings(w792, w791) -> (w795:string)
        n201 = Concatenate Strings(w789, w786) -> (w790:string)
        n202 = Concatenate Strings(w780, w781) -> (w779:string)
        n203 = Hexadecimal String To Number(string=w795, default (0uL)=w778) -> (number=→"Motor Current ADC":u16)  [unwired: 1 in, 1 out]
        n204 = Hexadecimal String To Number(string=w790, default (0uL)=w778) -> (number=→"Temp ADC":u16)  [unwired: 1 in, 1 out]
        n205 = Hexadecimal String To Number(string=w779, default (0uL)=w778) -> (number=→"Pressure ADC":u16)  [unwired: 1 in, 1 out]
        n206 = call "GEA2 Stop.vi"("GEA2 Reference In"=w770, "Error In"=w771) -> ("Error Out"=w769:errorcluster)  [unwired: 13 in]
      }
      event "Cycle Info Button": Value Change {
        w816 = T10 {"Source"=245, "Destination"=35, "Command"=240, "Message"="09F123F101F102F103F124F107F10DF10EF10C"}  # Cycle ERD
        n207 = event-data() -> ()  [unwired: 1 in, 6 out]
        n208 = call "GEA2 Initialize.vi"("Board Index"=w807, "Source Address"=u8 228, "error in"=w810) -> ("GeaCommunication.GeaBus"=w808:refnum<k24>, "error out"=w809:errorcluster)  [unwired: 10 in, 1 out]
        n209 = call "GEA2MessageFormatter.vi"("Prefix(Send/Recv)"="SEND", "GEA2 Data In"=w816, "Error In"=w809) -> ("Output String"=w815:string, "Error Out"=w818:errorcluster)  [unwired: 11 in]
        n210 = call "GExplorer_Queue_GEA2.vi"("Output String"=w815, "error in (no error)"=w818) -> ("error out"=w817:errorcluster)  [unwired: 13 in]
        n211 = call "GEA2 Send and Receive Message.vi"("GeaCommunication.GeaBus"=w808, "Input Data"=w816, "Error In"=w817) -> ("GeaCommunication.GeaBus"=w804:refnum<k24>, "Converted Data Out"=w813:T45, "Error Out"=w814:errorcluster)  [unwired: 9 in, 1 out]
        n212 = call "Convert_Cycle_Info.vi"("Converted Data In"=w813, "Error In"=w814) -> ("Cycle Information"=→"Cycle Information":T34, "Error Out"=w806:errorcluster)  [unwired: 12 in]
        n213 = call "GEA2 Stop.vi"("GEA2 Reference In"=w804, "Error In"=w806) -> ("Error Out"=w805:errorcluster)  [unwired: 13 in]
      }
      event "UI Launch Button": Value Change {
        w827 = 128  # options
        n214 = event-data() -> ()  [unwired: 1 in, 1 out]
        n215 = Current VI's Path() -> (path=w830:path)
        n216 = Strip Path(path=w830) -> (stripped path=w829:path)  [unwired: 1 out]
        n217 = Build Path(base path=w829, name or relative path="HEUI.vi") -> (appended path=w825:path)
        n218 = Open VI Reference(type specifier VI Refnum (for type only)=refnum<vi> refnum ("reference"), vi path=w825, options=w827, error in (no error)=w831) -> (vi reference=w823:refnum<vi>, error out=w826:errorcluster)  [unwired: 2 in]
        n219 = call-by-ref "Start Asynchronous Call"(reference=w823, error in=w826) -> (reference out=w820:refnum<vi>, error out=w822:errorcluster)  [unwired: 14 in, 2 out]
        n220 = Close Reference(reference=w820, error in (no error)=w822) -> (error out=w821:errorcluster)
      }
      event Value Change {
        n221 = event-data() -> ()  [unwired: 1 in, 6 out]
        n222 = call "GEA2 Initialize.vi"("Board Index"=w839, "Source Address"=u8 228, "error in"=w838) -> ("GeaCommunication.GeaBus"=w836:refnum<k24>, "error out"=w837:errorcluster)  [unwired: 10 in, 1 out]
        n223 = Bundle By Name(cluster=T40 {"ERD Number"=62229, "Data Type"=enum."string", "Data"=""} ("ERD Read Data In"), "Data"="01") -> (w842:T40)
        n224 = Build Array(w842) -> (w848:T40[])
        n225 = call "Convert Write ERD List to Message.vi"("GEA Inputs"=w832, "Write ERD List"=w848, "Error In"=w837) -> ("GEA Message"=w846:T10, "Error Out"=w845:errorcluster)  [unwired: 11 in]
        n226 = call "GEA2MessageFormatter.vi"("Prefix(Send/Recv)"="SEND", "GEA2 Data In"=w846, "Error In"=w845) -> ("Output String"=w844:string, "Error Out"=w843:errorcluster)  [unwired: 11 in]
        n227 = call "GExplorer_Queue_GEA2.vi"("Output String"=w844, "error in (no error)"=w843) -> ("error out"=w847:errorcluster)  [unwired: 13 in]
        n228 = call "GEA2 Write ERD.vi"("GEA2 Reference In"=w836, "GEA Inputs"=w832, "Write ERD List"=w848, "Error In"=w847) -> ("GEA2 Reference Out"=w835:refnum<k24>, "Error Out"=w834:errorcluster)  [unwired: 9 in, 1 out]
        n229 = call "GEA2 Stop.vi"("GEA2 Reference In"=w835, "Error In"=w834) -> ("Error Out"=w833:errorcluster)  [unwired: 13 in]
      }
      event Value Change {
        n230 = event-data() -> ()  [unwired: 1 in, 6 out]
        n231 = call "GEA2 Initialize.vi"("Board Index"=w852, "Source Address"=u8 228, "error in"=w858) -> ("GeaCommunication.GeaBus"=w853:refnum<k24>, "error out"=w857:errorcluster)  [unwired: 10 in, 1 out]
        n232 = Bundle By Name(cluster=T40 {"ERD Number"=62230, "Data Type"=enum."string", "Data"=""} ("ERD Read Data In"), "Data"="01") -> (w868:T40)
        n233 = Build Array(w868) -> (w862:T40[])
        n234 = call "Convert Write ERD List to Message.vi"("GEA Inputs"=w851, "Write ERD List"=w862, "Error In"=w857) -> ("GEA Message"=w864:T10, "Error Out"=w865:errorcluster)  [unwired: 11 in]
        n235 = call "GEA2MessageFormatter.vi"("Prefix(Send/Recv)"="SEND", "GEA2 Data In"=w864, "Error In"=w865) -> ("Output String"=w866:string, "Error Out"=w867:errorcluster)  [unwired: 11 in]
        n236 = call "GExplorer_Queue_GEA2.vi"("Output String"=w866, "error in (no error)"=w867) -> ("error out"=w863:errorcluster)  [unwired: 13 in]
        n237 = call "GEA2 Write ERD.vi"("GEA2 Reference In"=w853, "GEA Inputs"=w851, "Write ERD List"=w862, "Error In"=w863) -> ("GEA2 Reference Out"=w854:refnum<k24>, "Error Out"=w856:errorcluster)  [unwired: 9 in, 1 out]
        n238 = call "GEA2 Stop.vi"("GEA2 Reference In"=w854, "Error In"=w856) -> ("Error Out"=w855:errorcluster)  [unwired: 13 in]
      }
      event Value Change {
        n239 = event-data() -> ()  [unwired: 1 in, 6 out]
        n240 = call "GEA2 Initialize.vi"("Board Index"=w875, "Source Address"=u8 228, "error in"=w877) -> ("GeaCommunication.GeaBus"=w871:refnum<k24>, "error out"=w876:errorcluster)  [unwired: 10 in, 1 out]
        n241 = Bundle By Name(cluster=T40 {"ERD Number"=62231, "Data Type"=enum."string", "Data"=""} ("ERD Read Data In"), "Data"="01") -> (w887:T40)
        n242 = Build Array(w887) -> (w881:T40[])
        n243 = call "Convert Write ERD List to Message.vi"("GEA Inputs"=w870, "Write ERD List"=w881, "Error In"=w876) -> ("GEA Message"=w883:T10, "Error Out"=w884:errorcluster)  [unwired: 11 in]
        n244 = call "GEA2MessageFormatter.vi"("Prefix(Send/Recv)"="SEND", "GEA2 Data In"=w883, "Error In"=w884) -> ("Output String"=w885:string, "Error Out"=w886:errorcluster)  [unwired: 11 in]
        n245 = call "GExplorer_Queue_GEA2.vi"("Output String"=w885, "error in (no error)"=w886) -> ("error out"=w882:errorcluster)  [unwired: 13 in]
        n246 = call "GEA2 Write ERD.vi"("GEA2 Reference In"=w871, "GEA Inputs"=w870, "Write ERD List"=w881, "Error In"=w882) -> ("GEA2 Reference Out"=w872:refnum<k24>, "Error Out"=w874:errorcluster)  [unwired: 9 in, 1 out]
        n247 = call "GEA2 Stop.vi"("GEA2 Reference In"=w872, "Error In"=w874) -> ("Error Out"=w873:errorcluster)  [unwired: 13 in]
      }
      event Value Change {
        n248 = event-data() -> ()  [unwired: 1 in, 6 out]
        n249 = call "GEA2 Initialize.vi"("Board Index"=w894, "Source Address"=u8 228, "error in"=w896) -> ("GeaCommunication.GeaBus"=w893:refnum<k24>, "error out"=w895:errorcluster)  [unwired: 10 in, 1 out]
        n250 = property on="Cycle Selection" class="DigNum (strict)"(error in=w895) -> (error out=w898:errorcluster, "Value"=w899:u8)  [unwired: 1 in, 1 out]
        n251 = Number To Hexadecimal String(1:i16 2 ("width (-)"), 2:w899) -> (0:w913:string)
        n252 = Concatenate Strings("01" ("string"), w913, "01" ("string")) -> (w911:string)
        n253 = Bundle By Name(cluster=T40 {"ERD Number"=61965, "Data Type"=enum."string", "Data"=""} ("ERD Read Data In"), "Data"=w911) -> (w909:T40)
        n254 = Build Array(w909) -> (w901:T40[])
        n255 = call "Convert Write ERD List to Message.vi"("GEA Inputs"=w889, "Write ERD List"=w901, "Error In"=w898) -> ("GEA Message"=w907:T10, "Error Out"=w903:errorcluster)  [unwired: 11 in]
        n256 = call "GEA2MessageFormatter.vi"("Prefix(Send/Recv)"="SEND", "GEA2 Data In"=w907, "Error In"=w903) -> ("Output String"=w905:string, "Error Out"=w904:errorcluster)  [unwired: 11 in]
        n257 = call "GExplorer_Queue_GEA2.vi"("Output String"=w905, "error in (no error)"=w904) -> ("error out"=w902:errorcluster)  [unwired: 13 in]
        n258 = call "GEA2 Write ERD.vi"("GEA2 Reference In"=w893, "GEA Inputs"=w889, "Write ERD List"=w901, "Error In"=w902) -> ("GEA2 Reference Out"=w890:refnum<k24>, "Error Out"=w892:errorcluster)  [unwired: 9 in, 1 out]
        n259 = call "GEA2 Stop.vi"("GEA2 Reference In"=w890, "Error In"=w892) -> ("Error Out"=w891:errorcluster)  [unwired: 13 in]
      }
      event Value Change {
        n260 = event-data() -> ()  [unwired: 1 in, 6 out]
        n261 = call "GEA2 Initialize.vi"("Board Index"=w919, "Source Address"=u8 228, "error in"=w921) -> ("GeaCommunication.GeaBus"=w915:refnum<k24>, "error out"=w920:errorcluster)  [unwired: 10 in, 1 out]
        n262 = property on="Cycle Selection" class="DigNum (strict)"(error in=w920) -> (error out=w923:errorcluster, "Value"=w924:u8)  [unwired: 1 in, 1 out]
        n263 = Number To Hexadecimal String(1:i16 2 ("width (-)"), 2:w924) -> (0:w938:string)
        n264 = Concatenate Strings("01" ("string"), w938, "02" ("string")) -> (w936:string)
        n265 = Bundle By Name(cluster=T40 {"ERD Number"=61965, "Data Type"=enum."string", "Data"=""} ("ERD Read Data In"), "Data"=w936) -> (w934:T40)
        n266 = Build Array(w934) -> (w926:T40[])
        n267 = call "Convert Write ERD List to Message.vi"("GEA Inputs"=w914, "Write ERD List"=w926, "Error In"=w923) -> ("GEA Message"=w932:T10, "Error Out"=w928:errorcluster)  [unwired: 11 in]
        n268 = call "GEA2MessageFormatter.vi"("Prefix(Send/Recv)"="SEND", "GEA2 Data In"=w932, "Error In"=w928) -> ("Output String"=w930:string, "Error Out"=w929:errorcluster)  [unwired: 11 in]
        n269 = call "GExplorer_Queue_GEA2.vi"("Output String"=w930, "error in (no error)"=w929) -> ("error out"=w927:errorcluster)  [unwired: 13 in]
        n270 = call "GEA2 Write ERD.vi"("GEA2 Reference In"=w915, "GEA Inputs"=w914, "Write ERD List"=w926, "Error In"=w927) -> ("GEA2 Reference Out"=w916:refnum<k24>, "Error Out"=w918:errorcluster)  [unwired: 9 in, 1 out]
        n271 = call "GEA2 Stop.vi"("GEA2 Reference In"=w916, "Error In"=w918) -> ("Error Out"=w917:errorcluster)  [unwired: 13 in]
      }
      event Value Change {
        n272 = event-data() -> ()  [unwired: 1 in, 6 out]
        n273 = call "GEA2 Initialize.vi"("Board Index"=w944, "Source Address"=u8 228, "error in"=w946) -> ("GeaCommunication.GeaBus"=w940:refnum<k24>, "error out"=w945:errorcluster)  [unwired: 10 in, 1 out]
        n274 = property on="Cycle Selection" class="DigNum (strict)"(error in=w945) -> (error out=w948:errorcluster, "Value"=w949:u8)  [unwired: 1 in, 1 out]
        n275 = Number To Hexadecimal String(1:i16 2 ("width (-)"), 2:w949) -> (0:w963:string)
        n276 = Concatenate Strings("01" ("string"), w963, "03" ("string")) -> (w961:string)
        n277 = Bundle By Name(cluster=T40 {"ERD Number"=61965, "Data Type"=enum."string", "Data"=""} ("ERD Read Data In"), "Data"=w961) -> (w959:T40)
        n278 = Build Array(w959) -> (w951:T40[])
        n279 = call "Convert Write ERD List to Message.vi"("GEA Inputs"=w939, "Write ERD List"=w951, "Error In"=w948) -> ("GEA Message"=w957:T10, "Error Out"=w953:errorcluster)  [unwired: 11 in]
        n280 = call "GEA2MessageFormatter.vi"("Prefix(Send/Recv)"="SEND", "GEA2 Data In"=w957, "Error In"=w953) -> ("Output String"=w955:string, "Error Out"=w954:errorcluster)  [unwired: 11 in]
        n281 = call "GExplorer_Queue_GEA2.vi"("Output String"=w955, "error in (no error)"=w954) -> ("error out"=w952:errorcluster)  [unwired: 13 in]
        n282 = call "GEA2 Write ERD.vi"("GEA2 Reference In"=w940, "GEA Inputs"=w939, "Write ERD List"=w951, "Error In"=w952) -> ("GEA2 Reference Out"=w941:refnum<k24>, "Error Out"=w943:errorcluster)  [unwired: 9 in, 1 out]
        n283 = call "GEA2 Stop.vi"("GEA2 Reference In"=w941, "Error In"=w943) -> ("Error Out"=w942:errorcluster)  [unwired: 13 in]
      }
      event Value Change {
        n284 = event-data() -> ()  [unwired: 1 in, 6 out]
        n285 = call "GEA2 Initialize.vi"("Board Index"=w969, "Source Address"=u8 228, "error in"=w971) -> ("GeaCommunication.GeaBus"=w965:refnum<k24>, "error out"=w970:errorcluster)  [unwired: 10 in, 1 out]
        n286 = property on="Cycle Selection" class="DigNum (strict)"(error in=w970) -> (error out=w973:errorcluster, "Value"=w974:u8)  [unwired: 1 in, 1 out]
        n287 = Number To Hexadecimal String(1:i16 2 ("width (-)"), 2:w974) -> (0:w988:string)
        n288 = Concatenate Strings("01" ("string"), w988, "04" ("string")) -> (w986:string)
        n289 = Bundle By Name(cluster=T40 {"ERD Number"=61965, "Data Type"=enum."string", "Data"=""} ("ERD Read Data In"), "Data"=w986) -> (w984:T40)
        n290 = Build Array(w984) -> (w976:T40[])
        n291 = call "Convert Write ERD List to Message.vi"("GEA Inputs"=w964, "Write ERD List"=w976, "Error In"=w973) -> ("GEA Message"=w982:T10, "Error Out"=w978:errorcluster)  [unwired: 11 in]
        n292 = call "GEA2MessageFormatter.vi"("Prefix(Send/Recv)"="SEND", "GEA2 Data In"=w982, "Error In"=w978) -> ("Output String"=w980:string, "Error Out"=w979:errorcluster)  [unwired: 11 in]
        n293 = call "GExplorer_Queue_GEA2.vi"("Output String"=w980, "error in (no error)"=w979) -> ("error out"=w977:errorcluster)  [unwired: 13 in]
        n294 = call "GEA2 Write ERD.vi"("GEA2 Reference In"=w965, "GEA Inputs"=w964, "Write ERD List"=w976, "Error In"=w977) -> ("GEA2 Reference Out"=w966:refnum<k24>, "Error Out"=w968:errorcluster)  [unwired: 9 in, 1 out]
        n295 = call "GEA2 Stop.vi"("GEA2 Reference In"=w966, "Error In"=w968) -> ("Error Out"=w967:errorcluster)  [unwired: 13 in]
      }
      event Value Change {
        n296 = event-data() -> ()  [unwired: 1 in, 6 out]
        n297 = call "GEA2 Initialize.vi"("Source Address"=u8 228, "error in"=w995) -> ("GeaCommunication.GeaBus"=w993:refnum<k24>, "error out"=w994:errorcluster)  [unwired: 11 in, 1 out]
        n298 = property on="Cycle Selection" class="DigNum (strict)"(error in=w994) -> (error out=w997:errorcluster, "Value"=w998:u8)  [unwired: 1 in, 1 out]
        n299 = Number To Hexadecimal String(1:i16 2 ("width (-)"), 2:w998) -> (0:w1012:string)
        n300 = Concatenate Strings("01" ("string"), w1012, "05" ("string")) -> (w1010:string)
        n301 = Bundle By Name(cluster=T40 {"ERD Number"=61965, "Data Type"=enum."string", "Data"=""} ("ERD Read Data In"), "Data"=w1010) -> (w1008:T40)
        n302 = Build Array(w1008) -> (w1000:T40[])
        n303 = call "Convert Write ERD List to Message.vi"("GEA Inputs"=w989, "Write ERD List"=w1000, "Error In"=w997) -> ("GEA Message"=w1006:T10, "Error Out"=w1002:errorcluster)  [unwired: 11 in]
        n304 = call "GEA2MessageFormatter.vi"("Prefix(Send/Recv)"="SEND", "GEA2 Data In"=w1006, "Error In"=w1002) -> ("Output String"=w1004:string, "Error Out"=w1003:errorcluster)  [unwired: 11 in]
        n305 = call "GExplorer_Queue_GEA2.vi"("Output String"=w1004, "error in (no error)"=w1003) -> ("error out"=w1001:errorcluster)  [unwired: 13 in]
        n306 = call "GEA2 Write ERD.vi"("GEA2 Reference In"=w993, "GEA Inputs"=w989, "Write ERD List"=w1000, "Error In"=w1001) -> ("GEA2 Reference Out"=w990:refnum<k24>, "Error Out"=w992:errorcluster)  [unwired: 9 in, 1 out]
        n307 = call "GEA2 Stop.vi"("GEA2 Reference In"=w990, "Error In"=w992) -> ("Error Out"=w991:errorcluster)  [unwired: 13 in]
      }
      event User Event {
        n308 = event-data() -> ()  [unwired: 1 in, 7 out]
      }
      event Value Change {
        n309 = event-data() -> ()  [unwired: 1 in, 1 out]
        n310 = call "GEA2 Initialize.vi"("Board Index"=w1019, "Source Address"=u8 228, "error in"=w1021) -> ("GeaCommunication.GeaBus"=w1018:refnum<k24>, "error out"=w1020:errorcluster)  [unwired: 10 in, 1 out]
        n311 = Unbundle By Name("Programming") -> ("File Path"=w1030:path)
        n312 = Generate User Event(user event=w1025, event data cluster=TRUE ("event data"), error in=w1020) -> (error out=w1024:errorcluster)  [unwired: 1 in, 1 out]
        n313 = Not Equal?(x=w1030, y=path "") -> (x != y?=w1032:bool)
        n314 = property on="Data ON" class="Bool (strict)"(error in=w1024, "Value"=FALSE ("Data On")) -> (error out=w1028:errorcluster)  [unwired: 1 in, 1 out]
        n315 = case shown="True" w1032 {
          tunnel: w1028 -> [w1035 w1036]
          tunnel: [w1035 w1037] -> w1026
          tunnel: w1018 -> [w1034 w1046]
          tunnel: w1030 -> [_ w1045]
          tunnel: [w1034 w1038] -> w1015
          frame False {
          }
          frame True {
            n316 = flat-sequence {
              tunnel: w1045 -> [w1052]
              tunnel: w1046 -> [w1053]
              tunnel: [w1049] -> w1044
              tunnel: [w1053] -> w1043
              tunnel: [w1052] -> w1042
              tunnel: w1036 -> [w1047]
              tunnel: w1044 -> [w1064]
              tunnel: w1043 -> [w1062]
              tunnel: w1042 -> [w1058]
              tunnel: [w1063] -> w1041
              tunnel: [w1056] -> w1040
              tunnel: [w1055] -> w1039
              tunnel: [w1069] -> w1037
              tunnel: w1041 -> [w1068]
              tunnel: w1040 -> [w1066]
              tunnel: [w1065] -> w1038
              tunnel: w1039 -> [w1065]
              frame #0 {
                w1048 = TRUE ("Blinking")
                w1051 = 10 items=["InvalidImage", "ImageRejected", "BoardNotFound", "UnableToGetGeaConfiguration", "WriteToFlashNotAllowed", "ImageDownloadedSuccessfully", "ImagePresent", "WriteToFlashFailed", "EraseFailed", "CrcFailed", " "] ("Result")
                n317 = property on="Result" class="Ring (strict)"(error in=w1047, "Value"=w1051) -> (error out=w1050:errorcluster)  [unwired: 1 in, 1 out]
                n318 = property on="Program Ind" class="Bool (strict)"(error in=w1050, "Blinking"=w1048, "Value"=w1048) -> (error out=w1049:errorcluster)  [unwired: 1 in, 1 out]
              }
              frame #1 {
                n319 = call "GEA2 Flash APL.vi"("GEA2 Reference In"=w1062, "Force Update?"=TRUE, "Source Address"=u8 228, "Destination Address"=u8 35, "File Path"=w1058, "Error In"=w1064, "Broadcast"=TRUE, "Reset?"=FALSE ("Reset Board?")) -> ("GEA2 Reference Out"=w1055:refnum<k24>, "Result"=w1056:i32, "Error Out"=w1063:errorcluster)  [unwired: 3 in, 2 out]
              }
              frame #2 {
                w1070 = FALSE ("Blinking")
                n320 = property on="Result" class="Ring (strict)"(error in=w1068, "Value"=w1066) -> (error out=w1067:errorcluster)  [unwired: 1 in, 1 out]
                n321 = property on="Program Ind" class="Bool (strict)"(error in=w1067, "Blinking"=w1070, "Value"=w1070) -> (error out=w1069:errorcluster)  [unwired: 1 in, 1 out]
              }
            }
          }
        }
        n322 = property on="Data ON" class="Bool (strict)"(error in=w1026, "Value"=FALSE ("Data ON")) -> (error out=w1017:errorcluster)  [unwired: 1 in, 1 out]
        n323 = call "GEA2 Stop.vi"("GEA2 Reference In"=w1015, "Error In"=w1017) -> ("Error Out"=w1016:errorcluster)  [unwired: 13 in]
      }
      event Value Change {
        w1080 = T10 {"Source"=245, "Destination"=35, "Command"=221, "Message"="F401"} ("Input Data")
        n324 = event-data() -> ()  [unwired: 1 in, 6 out]
        n325 = call "GEA2 Initialize.vi"("Source Address"=u8 228, "error in"=w1076) -> ("GeaCommunication.GeaBus"=w1074:refnum<k24>, "error out"=w1075:errorcluster)  [unwired: 11 in, 1 out]
        n326 = call "GEA2 Send Message.vi"("GEA2 Reference In"=w1074, "Input Data"=w1080, "Error In"=w1075) -> ("GEA2 Reference Out"=w1071:refnum<k24>, "Error Out"=w1082:errorcluster)  [unwired: 11 in]
        n327 = call "GEA2MessageFormatter.vi"("Prefix(Send/Recv)"="SEND", "GEA2 Data In"=w1080, "Error In"=w1082) -> ("Output String"=w1079:string, "Error Out"=w1078:errorcluster)  [unwired: 11 in]
        n328 = call "GExplorer_Queue_GEA2.vi"("Output String"=w1079, "error in (no error)"=w1078) -> ("error out"=w1073:errorcluster)  [unwired: 13 in]
        n329 = call "GEA2 Stop.vi"("GEA2 Reference In"=w1071, "Error In"=w1073) -> ("Error Out"=w1072:errorcluster)  [unwired: 13 in]
      }
      event "Lid Lock.Lock Lid", "Lid Lock.Unlock Lid", "Lid Lock.Reset Lock": Value Change {
        n330 = event-data() -> ("CtlRef"=w1096:refnum<vi>)  [unwired: 1 in]
        n331 = call "GEA2 Initialize.vi"("Board Index"=w1090, "Source Address"=u8 228, "error in"=w1089) -> ("GeaCommunication.GeaBus"=w1087:refnum<k24>, "error out"=w1088:errorcluster)  [unwired: 10 in, 1 out]
        n332 = property class="Bool"(reference=w1096, error in=w1088) -> (reference out=w1093:refnum<vi>, error out=w1094:errorcluster, "Label.Text"=w1095:string)
        n333 = Close Reference(reference=w1093, error in (no error)=w1094) -> (error out=w1092:errorcluster)
        n334 = case shown="\"Unlock Lid\"" w1095 {
          tunnel: [w1098 w1115 w1142] -> w1086
          tunnel: w1087 -> [w1100 w1117 w1141]
          tunnel: [w1099 w1116 w1140] -> w1084
          tunnel: w1092 -> [w1101 w1118 w1132]
          tunnel: w1083 -> [w1097 w1114 w1131]
          frame "Unlock Lid" {
            n335 = Concatenate Strings("01" ("string"), "00" ("string")) -> (w1112:string)
            n336 = Bundle By Name(cluster=T40 {"ERD Number"=61962, "Data Type"=enum."string", "Data"=""} ("ERD Read Data In"), "Data"=w1112) -> (w1110:T40)
            n337 = Build Array(w1110) -> (w1103:T40[])
            n338 = call "Convert Write ERD List to Message.vi"("GEA Inputs"=w1097, "Write ERD List"=w1103, "Error In"=w1101) -> ("GEA Message"=w1105:T10, "Error Out"=w1106:errorcluster)  [unwired: 11 in]
            n339 = call "GEA2MessageFormatter.vi"("Prefix(Send/Recv)"="SEND", "GEA2 Data In"=w1105, "Error In"=w1106) -> ("Output String"=w1107:string, "Error Out"=w1108:errorcluster)  [unwired: 11 in]
            n340 = call "GExplorer_Queue_GEA2.vi"("Output String"=w1107, "error in (no error)"=w1108) -> ("error out"=w1104:errorcluster)  [unwired: 13 in]
            n341 = call "GEA2 Write ERD.vi"("GEA2 Reference In"=w1100, "GEA Inputs"=w1097, "Write ERD List"=w1103, "Error In"=w1104) -> ("GEA2 Reference Out"=w1099:refnum<k24>, "Error Out"=w1098:errorcluster)  [unwired: 9 in, 1 out]
          }
          frame "Reset Lid", Default {
            n342 = Concatenate Strings("00" ("string"), "00" ("string")) -> (w1129:string)
            n343 = Bundle By Name(cluster=T40 {"ERD Number"=61962, "Data Type"=enum."string", "Data"=""} ("ERD Read Data In"), "Data"=w1129) -> (w1127:T40)
            n344 = Build Array(w1127) -> (w1120:T40[])
            n345 = call "Convert Write ERD List to Message.vi"("GEA Inputs"=w1114, "Write ERD List"=w1120, "Error In"=w1118) -> ("GEA Message"=w1122:T10, "Error Out"=w1123:errorcluster)  [unwired: 11 in]
            n346 = call "GEA2MessageFormatter.vi"("Prefix(Send/Recv)"="SEND", "GEA2 Data In"=w1122, "Error In"=w1123) -> ("Output String"=w1124:string, "Error Out"=w1125:errorcluster)  [unwired: 11 in]
            n347 = call "GExplorer_Queue_GEA2.vi"("Output String"=w1124, "error in (no error)"=w1125) -> ("error out"=w1121:errorcluster)  [unwired: 13 in]
            n348 = call "GEA2 Write ERD.vi"("GEA2 Reference In"=w1117, "GEA Inputs"=w1114, "Write ERD List"=w1120, "Error In"=w1121) -> ("GEA2 Reference Out"=w1116:refnum<k24>, "Error Out"=w1115:errorcluster)  [unwired: 9 in, 1 out]
          }
          frame "Lock Lid" {
            n349 = Concatenate Strings("01" ("string"), "01" ("string")) -> (w1146:string)
            n350 = Bundle By Name(cluster=T40 {"ERD Number"=61962, "Data Type"=enum."string", "Data"=""} ("ERD Read Data In"), "Data"=w1146) -> (w1144:T40)
            n351 = Build Array(w1144) -> (w1134:T40[])
            n352 = call "Convert Write ERD List to Message.vi"("GEA Inputs"=w1131, "Write ERD List"=w1134, "Error In"=w1132) -> ("GEA Message"=w1136:T10, "Error Out"=w1137:errorcluster)  [unwired: 11 in]
            n353 = call "GEA2MessageFormatter.vi"("Prefix(Send/Recv)"="SEND", "GEA2 Data In"=w1136, "Error In"=w1137) -> ("Output String"=w1138:string, "Error Out"=w1139:errorcluster)  [unwired: 11 in]
            n354 = call "GExplorer_Queue_GEA2.vi"("Output String"=w1138, "error in (no error)"=w1139) -> ("error out"=w1135:errorcluster)  [unwired: 13 in]
            n355 = call "GEA2 Write ERD.vi"("GEA2 Reference In"=w1141, "GEA Inputs"=w1131, "Write ERD List"=w1134, "Error In"=w1135) -> ("GEA2 Reference Out"=w1140:refnum<k24>, "Error Out"=w1142:errorcluster)  [unwired: 9 in, 1 out]
          }
        }
        n356 = call "GEA2 Stop.vi"("GEA2 Reference In"=w1084, "Error In"=w1086) -> ("Error Out"=w1085:errorcluster)  [unwired: 13 in]
      }
      event "Drain Pump.Dain Pump ON": Value Change {
        n357 = event-data() -> ()  [unwired: 1 in, 6 out]
        n358 = call "GEA2 Initialize.vi"("Board Index"=w1153, "Source Address"=u8 228, "error in"=w1155) -> ("GeaCommunication.GeaBus"=w1152:refnum<k24>, "error out"=w1154:errorcluster)  [unwired: 10 in, 1 out]
        n359 = Concatenate Strings("01" ("string"), "01" ("string")) -> (w1167:string)
        n360 = Bundle By Name(cluster=T40 {"ERD Number"=61968, "Data Type"=enum."string", "Data"=""} ("ERD Read Data In"), "Data"=w1167) -> (w1165:T40)
        n361 = Build Array(w1165) -> (w1158:T40[])
        n362 = call "Convert Write ERD List to Message.vi"("GEA Inputs"=w1148, "Write ERD List"=w1158, "Error In"=w1154) -> ("GEA Message"=w1160:T10, "Error Out"=w1161:errorcluster)  [unwired: 11 in]
        n363 = call "GEA2MessageFormatter.vi"("Prefix(Send/Recv)"="SEND", "GEA2 Data In"=w1160, "Error In"=w1161) -> ("Output String"=w1162:string, "Error Out"=w1163:errorcluster)  [unwired: 11 in]
        n364 = call "GExplorer_Queue_GEA2.vi"("Output String"=w1162, "error in (no error)"=w1163) -> ("error out"=w1159:errorcluster)  [unwired: 13 in]
        n365 = call "GEA2 Write ERD.vi"("GEA2 Reference In"=w1152, "GEA Inputs"=w1148, "Write ERD List"=w1158, "Error In"=w1159) -> ("GEA2 Reference Out"=w1149:refnum<k24>, "Error Out"=w1151:errorcluster)  [unwired: 9 in, 1 out]
        n366 = call "GEA2 Stop.vi"("GEA2 Reference In"=w1149, "Error In"=w1151) -> ("Error Out"=w1150:errorcluster)  [unwired: 13 in]
      }
      event "Drain Pump.Drain Pump OFF": Value Change {
        n367 = event-data() -> ()  [unwired: 1 in, 6 out]
        n368 = call "GEA2 Initialize.vi"("Source Address"=u8 228, "error in"=w1175) -> ("GeaCommunication.GeaBus"=w1170:refnum<k24>, "error out"=w1174:errorcluster)  [unwired: 11 in, 1 out]
        n369 = Concatenate Strings("01" ("string"), "00" ("string")) -> (w1187:string)
        n370 = Bundle By Name(cluster=T40 {"ERD Number"=61968, "Data Type"=enum."string", "Data"=""} ("ERD Read Data In"), "Data"=w1187) -> (w1185:T40)
        n371 = Build Array(w1185) -> (w1178:T40[])
        n372 = call "Convert Write ERD List to Message.vi"("GEA Inputs"=w1169, "Write ERD List"=w1178, "Error In"=w1174) -> ("GEA Message"=w1180:T10, "Error Out"=w1181:errorcluster)  [unwired: 11 in]
        n373 = call "GEA2MessageFormatter.vi"("Prefix(Send/Recv)"="SEND", "GEA2 Data In"=w1180, "Error In"=w1181) -> ("Output String"=w1182:string, "Error Out"=w1183:errorcluster)  [unwired: 11 in]
        n374 = call "GExplorer_Queue_GEA2.vi"("Output String"=w1182, "error in (no error)"=w1183) -> ("error out"=w1179:errorcluster)  [unwired: 13 in]
        n375 = call "GEA2 Write ERD.vi"("GEA2 Reference In"=w1170, "GEA Inputs"=w1169, "Write ERD List"=w1178, "Error In"=w1179) -> ("GEA2 Reference Out"=w1171:refnum<k24>, "Error Out"=w1173:errorcluster)  [unwired: 9 in, 1 out]
        n376 = call "GEA2 Stop.vi"("GEA2 Reference In"=w1171, "Error In"=w1173) -> ("Error Out"=w1172:errorcluster)  [unwired: 13 in]
      }
      event "Drain Pump.Reset Drain Pump": Value Change {
        n377 = event-data() -> ()  [unwired: 1 in, 6 out]
        n378 = call "GEA2 Initialize.vi"("Board Index"=w1191, "Source Address"=u8 228, "error in"=w1193) -> ("GeaCommunication.GeaBus"=w1190:refnum<k24>, "error out"=w1192:errorcluster)  [unwired: 10 in, 1 out]
        n379 = Concatenate Strings("00" ("string"), "00" ("string")) -> (w1208:string)
        n380 = Bundle By Name(cluster=T40 {"ERD Number"=61968, "Data Type"=enum."string", "Data"=""} ("ERD Read Data In"), "Data"=w1208) -> (w1206:T40)
        n381 = Build Array(w1206) -> (w1199:T40[])
        n382 = call "Convert Write ERD List to Message.vi"("GEA Inputs"=w1189, "Write ERD List"=w1199, "Error In"=w1192) -> ("GEA Message"=w1201:T10, "Error Out"=w1202:errorcluster)  [unwired: 11 in]
        n383 = call "GEA2MessageFormatter.vi"("Prefix(Send/Recv)"="SEND", "GEA2 Data In"=w1201, "Error In"=w1202) -> ("Output String"=w1203:string, "Error Out"=w1204:errorcluster)  [unwired: 11 in]
        n384 = call "GExplorer_Queue_GEA2.vi"("Output String"=w1203, "error in (no error)"=w1204) -> ("error out"=w1200:errorcluster)  [unwired: 13 in]
        n385 = call "GEA2 Write ERD.vi"("GEA2 Reference In"=w1190, "GEA Inputs"=w1189, "Write ERD List"=w1199, "Error In"=w1200) -> ("GEA2 Reference Out"=w1195:refnum<k24>, "Error Out"=w1197:errorcluster)  [unwired: 9 in, 1 out]
        n386 = call "GEA2 Stop.vi"("GEA2 Reference In"=w1195, "Error In"=w1197) -> ("Error Out"=w1196:errorcluster)  [unwired: 13 in]
      }
      event "Recirculation Pump.Recirc Pump ON": Value Change {
        n387 = event-data() -> ()  [unwired: 1 in, 6 out]
        n388 = call "GEA2 Initialize.vi"("Board Index"=w1217, "Source Address"=u8 228, "error in"=w1218) -> ("GeaCommunication.GeaBus"=w1215:refnum<k24>, "error out"=w1216:errorcluster)  [unwired: 10 in, 1 out]
        n389 = Concatenate Strings("01" ("string"), "01" ("string")) -> (w1229:string)
        n390 = Bundle By Name(cluster=T40 {"ERD Number"=61969, "Data Type"=enum."string", "Data"=""} ("ERD Read Data In"), "Data"=w1229) -> (w1227:T40)
        n391 = Build Array(w1227) -> (w1220:T40[])
        n392 = call "Convert Write ERD List to Message.vi"("GEA Inputs"=w1210, "Write ERD List"=w1220, "Error In"=w1216) -> ("GEA Message"=w1222:T10, "Error Out"=w1223:errorcluster)  [unwired: 11 in]
        n393 = call "GEA2MessageFormatter.vi"("Prefix(Send/Recv)"="SEND", "GEA2 Data In"=w1222, "Error In"=w1223) -> ("Output String"=w1224:string, "Error Out"=w1225:errorcluster)  [unwired: 11 in]
        n394 = call "GExplorer_Queue_GEA2.vi"("Output String"=w1224, "error in (no error)"=w1225) -> ("error out"=w1221:errorcluster)  [unwired: 13 in]
        n395 = call "GEA2 Write ERD.vi"("GEA2 Reference In"=w1215, "GEA Inputs"=w1210, "Write ERD List"=w1220, "Error In"=w1221) -> ("GEA2 Reference Out"=w1212:refnum<k24>, "Error Out"=w1214:errorcluster)  [unwired: 9 in, 1 out]
        n396 = call "GEA2 Stop.vi"("GEA2 Reference In"=w1212, "Error In"=w1214) -> ("Error Out"=w1213:errorcluster)  [unwired: 13 in]
      }
      event "Recirculation Pump.Recirc Pump OFF": Value Change {
        n397 = event-data() -> ()  [unwired: 1 in, 6 out]
        n398 = call "GEA2 Initialize.vi"("Board Index"=w1237, "Source Address"=u8 228, "error in"=w1238) -> ("GeaCommunication.GeaBus"=w1235:refnum<k24>, "error out"=w1236:errorcluster)  [unwired: 10 in, 1 out]
        n399 = Concatenate Strings("01" ("string"), "00" ("string")) -> (w1250:string)
        n400 = Bundle By Name(cluster=T40 {"ERD Number"=61969, "Data Type"=enum."string", "Data"=""} ("ERD Read Data In"), "Data"=w1250) -> (w1248:T40)
        n401 = Build Array(w1248) -> (w1241:T40[])
        n402 = call "Convert Write ERD List to Message.vi"("GEA Inputs"=w1231, "Write ERD List"=w1241, "Error In"=w1236) -> ("GEA Message"=w1243:T10, "Error Out"=w1244:errorcluster)  [unwired: 11 in]
        n403 = call "GEA2MessageFormatter.vi"("Prefix(Send/Recv)"="SEND", "GEA2 Data In"=w1243, "Error In"=w1244) -> ("Output String"=w1245:string, "Error Out"=w1246:errorcluster)  [unwired: 11 in]
        n404 = call "GExplorer_Queue_GEA2.vi"("Output String"=w1245, "error in (no error)"=w1246) -> ("error out"=w1242:errorcluster)  [unwired: 13 in]
        n405 = call "GEA2 Write ERD.vi"("GEA2 Reference In"=w1235, "GEA Inputs"=w1231, "Write ERD List"=w1241, "Error In"=w1242) -> ("GEA2 Reference Out"=w1234:refnum<k24>, "Error Out"=w1233:errorcluster)  [unwired: 9 in, 1 out]
        n406 = call "GEA2 Stop.vi"("GEA2 Reference In"=w1234, "Error In"=w1233) -> ("Error Out"=w1232:errorcluster)  [unwired: 13 in]
      }
      event "Recirculation Pump.Reset Recirc Pump": Value Change {
        n407 = event-data() -> ()  [unwired: 1 in, 6 out]
        n408 = call "GEA2 Initialize.vi"("Board Index"=w1258, "Source Address"=u8 228, "error in"=w1259) -> ("GeaCommunication.GeaBus"=w1256:refnum<k24>, "error out"=w1257:errorcluster)  [unwired: 10 in, 1 out]
        n409 = Concatenate Strings("00" ("string"), "00" ("string")) -> (w1271:string)
        n410 = Bundle By Name(cluster=T40 {"ERD Number"=61969, "Data Type"=enum."string", "Data"=""} ("ERD Read Data In"), "Data"=w1271) -> (w1269:T40)
        n411 = Build Array(w1269) -> (w1262:T40[])
        n412 = call "Convert Write ERD List to Message.vi"("GEA Inputs"=w1252, "Write ERD List"=w1262, "Error In"=w1257) -> ("GEA Message"=w1264:T10, "Error Out"=w1265:errorcluster)  [unwired: 11 in]
        n413 = call "GEA2MessageFormatter.vi"("Prefix(Send/Recv)"="SEND", "GEA2 Data In"=w1264, "Error In"=w1265) -> ("Output String"=w1266:string, "Error Out"=w1267:errorcluster)  [unwired: 11 in]
        n414 = call "GExplorer_Queue_GEA2.vi"("Output String"=w1266, "error in (no error)"=w1267) -> ("error out"=w1263:errorcluster)  [unwired: 13 in]
        n415 = call "GEA2 Write ERD.vi"("GEA2 Reference In"=w1256, "GEA Inputs"=w1252, "Write ERD List"=w1262, "Error In"=w1263) -> ("GEA2 Reference Out"=w1253:refnum<k24>, "Error Out"=w1255:errorcluster)  [unwired: 9 in, 1 out]
        n416 = call "GEA2 Stop.vi"("GEA2 Reference In"=w1253, "Error In"=w1255) -> ("Error Out"=w1254:errorcluster)  [unwired: 13 in]
      }
      event "Mode Shift.Shift to Agitate": Value Change {
        n417 = event-data() -> ()  [unwired: 1 in, 6 out]
        n418 = call "GEA2 Initialize.vi"("Board Index"=w1278, "Source Address"=u8 228, "error in"=w1280) -> ("GeaCommunication.GeaBus"=w1277:refnum<k24>, "error out"=w1279:errorcluster)  [unwired: 10 in, 1 out]
        n419 = Concatenate Strings("01" ("string")) -> (w1292:string)
        n420 = Bundle By Name(cluster=T40 {"ERD Number"=62238, "Data Type"=enum."string", "Data"=""} ("ERD Read Data In"), "Data"=w1292) -> (w1290:T40)
        n421 = Build Array(w1290) -> (w1283:T40[])
        n422 = call "Convert Write ERD List to Message.vi"("GEA Inputs"=w1273, "Write ERD List"=w1283, "Error In"=w1279) -> ("GEA Message"=w1285:T10, "Error Out"=w1286:errorcluster)  [unwired: 11 in]
        n423 = call "GEA2MessageFormatter.vi"("Prefix(Send/Recv)"="SEND", "GEA2 Data In"=w1285, "Error In"=w1286) -> ("Output String"=w1287:string, "Error Out"=w1288:errorcluster)  [unwired: 11 in]
        n424 = call "GExplorer_Queue_GEA2.vi"("Output String"=w1287, "error in (no error)"=w1288) -> ("error out"=w1284:errorcluster)  [unwired: 13 in]
        n425 = call "GEA2 Write ERD.vi"("GEA2 Reference In"=w1277, "GEA Inputs"=w1273, "Write ERD List"=w1283, "Error In"=w1284) -> ("GEA2 Reference Out"=w1274:refnum<k24>, "Error Out"=w1276:errorcluster)  [unwired: 9 in, 1 out]
        n426 = call "GEA2 Stop.vi"("GEA2 Reference In"=w1274, "Error In"=w1276) -> ("Error Out"=w1275:errorcluster)  [unwired: 13 in]
      }
      event "Mode Shift.Shift to Spin": Value Change {
        n427 = event-data() -> ()  [unwired: 1 in, 6 out]
        n428 = call "GEA2 Initialize.vi"("Board Index"=w1298, "Source Address"=u8 228, "error in"=w1301) -> ("GeaCommunication.GeaBus"=w1297:refnum<k24>, "error out"=w1300:errorcluster)  [unwired: 10 in, 1 out]
        n429 = Concatenate Strings("02" ("string")) -> (w1312:string)
        n430 = Bundle By Name(cluster=T40 {"ERD Number"=62238, "Data Type"=enum."string", "Data"=""} ("ERD Read Data In"), "Data"=w1312) -> (w1310:T40)
        n431 = Build Array(w1310) -> (w1303:T40[])
        n432 = call "Convert Write ERD List to Message.vi"("GEA Inputs"=w1293, "Write ERD List"=w1303, "Error In"=w1300) -> ("GEA Message"=w1305:T10, "Error Out"=w1306:errorcluster)  [unwired: 11 in]
        n433 = call "GEA2MessageFormatter.vi"("Prefix(Send/Recv)"="SEND", "GEA2 Data In"=w1305, "Error In"=w1306) -> ("Output String"=w1307:string, "Error Out"=w1308:errorcluster)  [unwired: 11 in]
        n434 = call "GExplorer_Queue_GEA2.vi"("Output String"=w1307, "error in (no error)"=w1308) -> ("error out"=w1304:errorcluster)  [unwired: 13 in]
        n435 = call "GEA2 Write ERD.vi"("GEA2 Reference In"=w1297, "GEA Inputs"=w1293, "Write ERD List"=w1303, "Error In"=w1304) -> ("GEA2 Reference Out"=w1294:refnum<k24>, "Error Out"=w1296:errorcluster)  [unwired: 9 in, 1 out]
        n436 = call "GEA2 Stop.vi"("GEA2 Reference In"=w1294, "Error In"=w1296) -> ("Error Out"=w1295:errorcluster)  [unwired: 13 in]
      }
      event "Mode Shift.Disable": Value Change {
        n437 = event-data() -> ()  [unwired: 1 in, 6 out]
        n438 = call "GEA2 Initialize.vi"("Board Index"=w1318, "Source Address"=u8 228, "error in"=w1320) -> ("GeaCommunication.GeaBus"=w1317:refnum<k24>, "error out"=w1319:errorcluster)  [unwired: 10 in, 1 out]
        n439 = Concatenate Strings("00" ("string")) -> (w1332:string)
        n440 = Bundle By Name(cluster=T40 {"ERD Number"=62238, "Data Type"=enum."string", "Data"=""} ("ERD Read Data In"), "Data"=w1332) -> (w1330:T40)
        n441 = Build Array(w1330) -> (w1323:T40[])
        n442 = call "Convert Write ERD List to Message.vi"("GEA Inputs"=w1313, "Write ERD List"=w1323, "Error In"=w1319) -> ("GEA Message"=w1325:T10, "Error Out"=w1326:errorcluster)  [unwired: 11 in]
        n443 = call "GEA2MessageFormatter.vi"("Prefix(Send/Recv)"="SEND", "GEA2 Data In"=w1325, "Error In"=w1326) -> ("Output String"=w1327:string, "Error Out"=w1328:errorcluster)  [unwired: 11 in]
        n444 = call "GExplorer_Queue_GEA2.vi"("Output String"=w1327, "error in (no error)"=w1328) -> ("error out"=w1324:errorcluster)  [unwired: 13 in]
        n445 = call "GEA2 Write ERD.vi"("GEA2 Reference In"=w1317, "GEA Inputs"=w1313, "Write ERD List"=w1323, "Error In"=w1324) -> ("GEA2 Reference Out"=w1314:refnum<k24>, "Error Out"=w1316:errorcluster)  [unwired: 9 in, 1 out]
        n446 = call "GEA2 Stop.vi"("GEA2 Reference In"=w1314, "Error In"=w1316) -> ("Error Out"=w1315:errorcluster)  [unwired: 13 in]
      }
      event Value Change {
        n447 = event-data() -> ()  [unwired: 1 in, 6 out]
        n448 = call "GEA2 Initialize.vi"("Board Index"=w1338, "Source Address"=u8 228, "error in"=w1340) -> ("GeaCommunication.GeaBus"=w1337:refnum<k24>, "error out"=w1339:errorcluster)  [unwired: 10 in, 1 out]
        n449 = Unbundle By Name("Valve Control") -> ("Hot Valve"=w1357:bool, "Cold Valve"=w1356:bool, "SprayRinse Valve"=w1355:bool, "FabricSoftener Valve"=w1354:bool)
        n450 = Build Array(w1357, w1356, w1355, w1354) -> (w1353:bool[])
        n451 = Boolean Array To Number(Boolean array=w1353) -> (number=w1351:u32)
        n452 = Number To Hexadecimal String(1:i16 2 ("width (-)"), 2:w1351) -> (0:w1350:string)
        n453 = Bundle By Name(cluster=T40 {"ERD Number"=61961, "Data Type"=enum."string", "Data"=""} ("ERD Read Data In"), "Data"=w1350) -> (w1358:T40)
        n454 = Build Array(w1358) -> (w1342:T40[])
        n455 = call "Convert Write ERD List to Message.vi"("GEA Inputs"=w1333, "Write ERD List"=w1342, "Error In"=w1339) -> ("GEA Message"=w1345:T10, "Error Out"=w1346:errorcluster)  [unwired: 11 in]
        n456 = call "GEA2MessageFormatter.vi"("Prefix(Send/Recv)"="SEND", "GEA2 Data In"=w1345, "Error In"=w1346) -> ("Output String"=w1347:string, "Error Out"=w1348:errorcluster)  [unwired: 11 in]
        n457 = call "GExplorer_Queue_GEA2.vi"("Output String"=w1347, "error in (no error)"=w1348) -> ("error out"=w1344:errorcluster)  [unwired: 13 in]
        n458 = call "GEA2 Write ERD.vi"("GEA2 Reference In"=w1337, "GEA Inputs"=w1333, "Write ERD List"=w1342, "Error In"=w1344) -> ("GEA2 Reference Out"=w1334:refnum<k24>, "Error Out"=w1336:errorcluster)  [unwired: 9 in, 1 out]
        n459 = call "GEA2 Stop.vi"("GEA2 Reference In"=w1334, "Error In"=w1336) -> ("Error Out"=w1335:errorcluster)  [unwired: 13 in]
      }
      event Value Change {
        w1376 = FALSE ("Value")
        n460 = event-data() -> ()  [unwired: 1 in, 6 out]
        n461 = call "GEA2 Initialize.vi"("Board Index"=w1365, "Source Address"=u8 228, "error in"=w1368) -> ("GeaCommunication.GeaBus"=w1361:refnum<k24>, "error out"=w1367:errorcluster)  [unwired: 10 in, 1 out]
        n462 = Bundle By Name(cluster=T40 {"ERD Number"=61961, "Data Type"=enum."string", "Data"=""} ("ERD Read Data In"), "Data"="00" ("string")) -> (w1382:T40)
        n463 = Build Array(w1382) -> (w1369:T40[])
        n464 = call "Convert Write ERD List to Message.vi"("GEA Inputs"=w1360, "Write ERD List"=w1369, "Error In"=w1367) -> ("GEA Message"=w1372:T10, "Error Out"=w1373:errorcluster)  [unwired: 11 in]
        n465 = call "GEA2MessageFormatter.vi"("Prefix(Send/Recv)"="SEND", "GEA2 Data In"=w1372, "Error In"=w1373) -> ("Output String"=w1374:string, "Error Out"=w1375:errorcluster)  [unwired: 11 in]
        n466 = call "GExplorer_Queue_GEA2.vi"("Output String"=w1374, "error in (no error)"=w1375) -> ("error out"=w1370:errorcluster)  [unwired: 13 in]
        n467 = call "GEA2 Write ERD.vi"("GEA2 Reference In"=w1361, "GEA Inputs"=w1360, "Write ERD List"=w1369, "Error In"=w1370) -> ("GEA2 Reference Out"=w1362:refnum<k24>, "Error Out"=w1364:errorcluster)  [unwired: 9 in, 1 out]
        n468 = call "GEA2 Stop.vi"("GEA2 Reference In"=w1362, "Error In"=w1364) -> ("Error Out"=w1363:errorcluster)  [unwired: 13 in]
        n469 = property on="Hot Valve" class="Bool (strict)"(error in=w1363, "Value"=w1376) -> (error out=w1380:errorcluster)  [unwired: 1 in, 1 out]
        n470 = property on="Cold Valve" class="Bool (strict)"(error in=w1380, "Value"=w1376) -> (error out=w1379:errorcluster)  [unwired: 1 in, 1 out]
        n471 = property on="SprayRinse Valve" class="Bool (strict)"(error in=w1379, "Value"=w1376) -> (error out=w1378:errorcluster)  [unwired: 1 in, 1 out]
        n472 = property on="FabricSoftener Valve" class="Bool (strict)"(error in=w1378, "Value"=w1376) -> (error out=w1377:errorcluster)  [unwired: 1 in, 1 out]
      }
      event Value Change {
        n473 = event-data() -> ()  [unwired: 1 in, 6 out]
        n474 = Unbundle By Name("Motor Control") -> ("Motor Profile Mode"=w1385:u16)
        n475 = case shown="6" w1385 {
          tunnel: w1387 -> [w1391 w1395 w1403 w1410 w1417 w1424 w1430]
          tunnel: [w1394 w1400 w1404 w1414 w1421 w1428 w1434] -> w1386
          frame 0, Default {
            w1388 = T55."Enabled" ("Disabled")
            w1392 = T55."Disabled and Grayed Out" ("Disabled")
            n476 = property on="Speed (RPM)" class="DigNum (strict)"(error in=w1391, "DisabledEnum"=w1388) -> (error out=w1390:errorcluster)  [unwired: 1 in, 1 out]
            n477 = property on="Acceleration" class="DigNum (strict)"(error in=w1390, "DisabledEnum"=w1388) -> (error out=w1389:errorcluster)  [unwired: 1 in, 1 out]
            n478 = property on="Amplitude (%)\n-CCW +CW" class="DigNum (strict)"(error in=w1389, "DisabledEnum"=w1392) -> (error out=w1393:errorcluster)  [unwired: 1 in, 1 out]
            n479 = property on="Angle (Degrees)" class="DigNum (strict)"(error in=w1393, "DisabledEnum"=w1392) -> (error out=w1394:errorcluster)  [unwired: 1 in, 1 out]
          }
          frame 1 {
            w1396 = T55."Disabled and Grayed Out" ("Disabled")
            n480 = property on="Amplitude (%)\n-CCW +CW" class="DigNum (strict)"(error in=w1395, "DisabledEnum"=w1396) -> (error out=w1398:errorcluster)  [unwired: 1 in, 1 out]
            n481 = property on="Angle (Degrees)" class="DigNum (strict)"(error in=w1398, "DisabledEnum"=w1396) -> (error out=w1397:errorcluster)  [unwired: 1 in, 1 out]
            n482 = property on="Acceleration" class="DigNum (strict)"(error in=w1397, "DisabledEnum"=w1396) -> (error out=w1399:errorcluster)  [unwired: 1 in, 1 out]
            n483 = property on="Speed (RPM)" class="DigNum (strict)"(error in=w1399, "DisabledEnum"=w1396) -> (error out=w1400:errorcluster)  [unwired: 1 in, 1 out]
          }
          frame 2 {
            w1405 = T55."Disabled and Grayed Out" ("Disabled")
            n484 = property on="Amplitude (%)\n-CCW +CW" class="DigNum (strict)"(error in=w1403, "DisabledEnum"=T55."Enabled" ("Disabled")) -> (error out=w1402:errorcluster)  [unwired: 1 in, 1 out]
            n485 = property on="Angle (Degrees)" class="DigNum (strict)"(error in=w1402, "DisabledEnum"=w1405) -> (error out=w1407:errorcluster)  [unwired: 1 in, 1 out]
            n486 = property on="Acceleration" class="DigNum (strict)"(error in=w1407, "DisabledEnum"=w1405) -> (error out=w1406:errorcluster)  [unwired: 1 in, 1 out]
            n487 = property on="Speed (RPM)" class="DigNum (strict)"(error in=w1406, "DisabledEnum"=w1405) -> (error out=w1404:errorcluster)  [unwired: 1 in, 1 out]
          }
          frame 3 {
            w1408 = T55."Enabled" ("Disabled")
            w1412 = T55."Disabled and Grayed Out" ("Disabled")
            n488 = property on="Amplitude (%)\n-CCW +CW" class="DigNum (strict)"(error in=w1410, "DisabledEnum"=w1408) -> (error out=w1409:errorcluster)  [unwired: 1 in, 1 out]
            n489 = property on="Angle (Degrees)" class="DigNum (strict)"(error in=w1409, "DisabledEnum"=w1408) -> (error out=w1411:errorcluster)  [unwired: 1 in, 1 out]
            n490 = property on="Speed (RPM)" class="DigNum (strict)"(error in=w1411, "DisabledEnum"=w1412) -> (error out=w1413:errorcluster)  [unwired: 1 in, 1 out]
            n491 = property on="Acceleration" class="DigNum (strict)"(error in=w1413, "DisabledEnum"=w1412) -> (error out=w1414:errorcluster)  [unwired: 1 in, 1 out]
          }
          frame 4 {
            w1418 = T55."Disabled and Grayed Out" ("Disabled")
            n492 = property on="Speed (RPM)" class="DigNum (strict)"(error in=w1417, "DisabledEnum"=T55."Enabled" ("Disabled")) -> (error out=w1416:errorcluster)  [unwired: 1 in, 1 out]
            n493 = property on="Amplitude (%)\n-CCW +CW" class="DigNum (strict)"(error in=w1416, "DisabledEnum"=w1418) -> (error out=w1419:errorcluster)  [unwired: 1 in, 1 out]
            n494 = property on="Angle (Degrees)" class="DigNum (strict)"(error in=w1419, "DisabledEnum"=w1418) -> (error out=w1420:errorcluster)  [unwired: 1 in, 1 out]
            n495 = property on="Acceleration" class="DigNum (strict)"(error in=w1420, "DisabledEnum"=w1418) -> (error out=w1421:errorcluster)  [unwired: 1 in, 1 out]
          }
          frame 5 {
            w1425 = T55."Disabled and Grayed Out" ("Disabled")
            n496 = property on="Speed (RPM)" class="DigNum (strict)"(error in=w1424, "DisabledEnum"=T55."Enabled" ("Disabled")) -> (error out=w1423:errorcluster)  [unwired: 1 in, 1 out]
            n497 = property on="Amplitude (%)\n-CCW +CW" class="DigNum (strict)"(error in=w1423, "DisabledEnum"=w1425) -> (error out=w1426:errorcluster)  [unwired: 1 in, 1 out]
            n498 = property on="Angle (Degrees)" class="DigNum (strict)"(error in=w1426, "DisabledEnum"=w1425) -> (error out=w1427:errorcluster)  [unwired: 1 in, 1 out]
            n499 = property on="Acceleration" class="DigNum (strict)"(error in=w1427, "DisabledEnum"=w1425) -> (error out=w1428:errorcluster)  [unwired: 1 in, 1 out]
          }
          frame 6 {
            w1429 = T55."Disabled and Grayed Out" ("Disabled")
            n500 = property on="Amplitude (%)\n-CCW +CW" class="DigNum (strict)"(error in=w1430, "DisabledEnum"=w1429) -> (error out=w1431:errorcluster)  [unwired: 1 in, 1 out]
            n501 = property on="Angle (Degrees)" class="DigNum (strict)"(error in=w1431, "DisabledEnum"=w1429) -> (error out=w1432:errorcluster)  [unwired: 1 in, 1 out]
            n502 = property on="Acceleration" class="DigNum (strict)"(error in=w1432, "DisabledEnum"=w1429) -> (error out=w1433:errorcluster)  [unwired: 1 in, 1 out]
            n503 = property on="Speed (RPM)" class="DigNum (strict)"(error in=w1433, "DisabledEnum"=w1429) -> (error out=w1434:errorcluster)  [unwired: 1 in, 1 out]
          }
        }
      }
      event Value Change {
        n504 = event-data() -> ()  [unwired: 1 in, 6 out]
        n505 = call "GEA2 Initialize.vi"("Board Index"=w1440, "Source Address"=u8 228, "error in"=w1442) -> ("GeaCommunication.GeaBus"=w1439:refnum<k24>, "error out"=w1441:errorcluster)  [unwired: 10 in, 1 out]
        n506 = property on="Amplitude (%)\n-CCW +CW" class="DigNum (strict)"() -> ("Value"=w1449:i16)  [unwired: 2 in, 2 out]
        n507 = property on="Angle (Degrees)" class="DigNum (strict)"() -> ("Value"=w1450:i16)  [unwired: 2 in, 2 out]
        n508 = property on="Motor Profile Mode" class="Ring (strict)"() -> ("Value"=w1459:u16)  [unwired: 2 in, 2 out]
        n509 = property on="Speed (RPM)" class="DigNum (strict)"() -> ("Value"=w1455:i16)  [unwired: 2 in, 2 out]
        n510 = property on="Acceleration" class="DigNum (strict)"() -> ("Value"=w1451:i16)  [unwired: 2 in, 2 out]
        n511 = Number To Hexadecimal String(1:i16 2 ("width (-)"), 2:w1459) -> (0:w1458:string)
        n512 = Number To Hexadecimal String(1:i16 4 ("width (-)"), 2:w1455) -> (0:w1457:string)
        n513 = Number To Hexadecimal String(1:i16 4 ("width (-)"), 2:w1451) -> (0:w1448:string)
        n514 = Number To Hexadecimal String(1:i16 4 ("width (-)"), 2:w1450) -> (0:w1447:string)
        n515 = Number To Hexadecimal String(1:i16 4 ("width (-)"), 2:w1449) -> (0:w1446:string)
        n516 = Concatenate Strings(w1458, "00" ("string"), w1457, w1448, w1447, "0000" ("string"), w1446) -> (w1470:string)
        n517 = Bundle By Name(cluster=T40 {"ERD Number"=62232, "Data Type"=enum."string", "Data"=""} ("ERD Read Data In"), "Data"=w1470) -> (w1468:T40)
        n518 = Build Array(w1468) -> (w1462:T40[])
        n519 = call "Convert Write ERD List to Message.vi"("GEA Inputs"=w1435, "Write ERD List"=w1462, "Error In"=w1441) -> ("GEA Message"=w1464:T10, "Error Out"=w1465:errorcluster)  [unwired: 11 in]
        n520 = call "GEA2MessageFormatter.vi"("Prefix(Send/Recv)"="SEND", "GEA2 Data In"=w1464, "Error In"=w1465) -> ("Output String"=w1466:string, "Error Out"=w1467:errorcluster)  [unwired: 11 in]
        n521 = call "GExplorer_Queue_GEA2.vi"("Output String"=w1466, "error in (no error)"=w1467) -> ("error out"=w1463:errorcluster)  [unwired: 13 in]
        n522 = call "GEA2 Write ERD.vi"("GEA2 Reference In"=w1439, "GEA Inputs"=w1435, "Write ERD List"=w1462, "Error In"=w1463) -> ("GEA2 Reference Out"=w1436:refnum<k24>, "Error Out"=w1438:errorcluster)  [unwired: 9 in, 1 out]
        n523 = call "GEA2 Stop.vi"("GEA2 Reference In"=w1436, "Error In"=w1438) -> ("Error Out"=w1437:errorcluster)  [unwired: 13 in]
      }
      event Value Change {
        n524 = event-data() -> ()  [unwired: 1 in, 6 out]
        n525 = call "GEA2 Initialize.vi"("Board Index"=w1476, "Source Address"=u8 228, "error in"=w1478) -> ("GeaCommunication.GeaBus"=w1475:refnum<k24>, "error out"=w1477:errorcluster)  [unwired: 10 in, 1 out]
        n526 = Concatenate Strings("06 00 00 00 00 00 00 00 00 00 00 00" ("string")) -> (w1490:string)
        n527 = Bundle By Name(cluster=T40 {"ERD Number"=62232, "Data Type"=enum."string", "Data"=""} ("ERD Read Data In"), "Data"=w1490) -> (w1488:T40)
        n528 = Build Array(w1488) -> (w1482:T40[])
        n529 = call "Convert Write ERD List to Message.vi"("GEA Inputs"=w1471, "Write ERD List"=w1482, "Error In"=w1477) -> ("GEA Message"=w1484:T10, "Error Out"=w1485:errorcluster)  [unwired: 11 in]
        n530 = call "GEA2MessageFormatter.vi"("Prefix(Send/Recv)"="SEND", "GEA2 Data In"=w1484, "Error In"=w1485) -> ("Output String"=w1486:string, "Error Out"=w1487:errorcluster)  [unwired: 11 in]
        n531 = call "GExplorer_Queue_GEA2.vi"("Output String"=w1486, "error in (no error)"=w1487) -> ("error out"=w1483:errorcluster)  [unwired: 13 in]
        n532 = call "GEA2 Write ERD.vi"("GEA2 Reference In"=w1475, "GEA Inputs"=w1471, "Write ERD List"=w1482, "Error In"=w1483) -> ("GEA2 Reference Out"=w1473:refnum<k24>, "Error Out"=w1474:errorcluster)  [unwired: 9 in, 1 out]
        n533 = call "GEA2 Stop.vi"("GEA2 Reference In"=w1473, "Error In"=w1474) -> ("Error Out"=w1472:errorcluster)  [unwired: 13 in]
      }
      event "LED Control.ALL LEDs ON": Value Change {
        n534 = event-data() -> ()  [unwired: 1 in, 6 out]
        n535 = call "GEA2 Initialize.vi"("Board Index"=w1497, "Source Address"=u8 228, "error in"=w1496) -> ("GeaCommunication.GeaBus"=w1495:refnum<k24>, "error out"=w1498:errorcluster)  [unwired: 10 in, 1 out]
        n536 = Concatenate Strings("0101FFFFFFFFFFFFFFFFFFFF" ("string")) -> (w1510:string)
        n537 = Bundle By Name(cluster=T40 {"ERD Number"=61724, "Data Type"=enum."string", "Data"=""} ("ERD Read Data In"), "Data"=w1510) -> (w1508:T40)
        n538 = Build Array(w1508) -> (w1501:T40[])
        n539 = call "Convert Write ERD List to Message.vi"("GEA Inputs"=w1491, "Write ERD List"=w1501, "Error In"=w1498) -> ("GEA Message"=w1503:T10, "Error Out"=w1504:errorcluster)  [unwired: 11 in]
        n540 = call "GEA2MessageFormatter.vi"("Prefix(Send/Recv)"="SEND", "GEA2 Data In"=w1503, "Error In"=w1504) -> ("Output String"=w1505:string, "Error Out"=w1506:errorcluster)  [unwired: 11 in]
        n541 = call "GExplorer_Queue_GEA2.vi"("Output String"=w1505, "error in (no error)"=w1506) -> ("error out"=w1502:errorcluster)  [unwired: 13 in]
        n542 = call "GEA2 Write ERD.vi"("GEA2 Reference In"=w1495, "GEA Inputs"=w1491, "Write ERD List"=w1501, "Error In"=w1502) -> ("GEA2 Reference Out"=w1492:refnum<k24>, "Error Out"=w1494:errorcluster)  [unwired: 9 in, 1 out]
        n543 = call "GEA2 Stop.vi"("GEA2 Reference In"=w1492, "Error In"=w1494) -> ("Error Out"=w1493:errorcluster)  [unwired: 13 in]
      }
      event "LED Control.ALL LEDs OFF": Value Change {
        n544 = event-data() -> ()  [unwired: 1 in, 6 out]
        n545 = call "GEA2 Initialize.vi"("Board Index"=w1516, "Source Address"=u8 228, "error in"=w1519) -> ("GeaCommunication.GeaBus"=w1515:refnum<k24>, "error out"=w1518:errorcluster)  [unwired: 10 in, 1 out]
        n546 = Concatenate Strings("010100000000000000000000" ("string")) -> (w1530:string)
        n547 = Bundle By Name(cluster=T40 {"ERD Number"=61724, "Data Type"=enum."string", "Data"=""} ("ERD Read Data In"), "Data"=w1530) -> (w1528:T40)
        n548 = Build Array(w1528) -> (w1521:T40[])
        n549 = call "Convert Write ERD List to Message.vi"("GEA Inputs"=w1511, "Write ERD List"=w1521, "Error In"=w1518) -> ("GEA Message"=w1523:T10, "Error Out"=w1524:errorcluster)  [unwired: 11 in]
        n550 = call "GEA2MessageFormatter.vi"("Prefix(Send/Recv)"="SEND", "GEA2 Data In"=w1523, "Error In"=w1524) -> ("Output String"=w1525:string, "Error Out"=w1526:errorcluster)  [unwired: 11 in]
        n551 = call "GExplorer_Queue_GEA2.vi"("Output String"=w1525, "error in (no error)"=w1526) -> ("error out"=w1522:errorcluster)  [unwired: 13 in]
        n552 = call "GEA2 Write ERD.vi"("GEA2 Reference In"=w1515, "GEA Inputs"=w1511, "Write ERD List"=w1521, "Error In"=w1522) -> ("GEA2 Reference Out"=w1512:refnum<k24>, "Error Out"=w1514:errorcluster)  [unwired: 9 in, 1 out]
        n553 = call "GEA2 Stop.vi"("GEA2 Reference In"=w1512, "Error In"=w1514) -> ("Error Out"=w1513:errorcluster)  [unwired: 13 in]
      }
      event "LED Control.Reset LEDs": Value Change {
        n554 = event-data() -> ()  [unwired: 1 in, 6 out]
        n555 = call "GEA2 Initialize.vi"("Board Index"=w1536, "Source Address"=u8 228, "error in"=w1538) -> ("GeaCommunication.GeaBus"=w1535:refnum<k24>, "error out"=w1537:errorcluster)  [unwired: 10 in, 1 out]
        n556 = Concatenate Strings("010100000000000000000000" ("string")) -> (w1552:string)
        n557 = Bundle By Name(cluster=T40 {"ERD Number"=61724, "Data Type"=enum."string", "Data"=""} ("ERD Read Data In"), "Data"=w1552) -> (w1550:T40)
        n558 = Build Array(w1550) -> (w1543:T40[])
        n559 = call "Convert Write ERD List to Message.vi"("GEA Inputs"=w1531, "Write ERD List"=w1543, "Error In"=w1537) -> ("GEA Message"=w1545:T10, "Error Out"=w1546:errorcluster)  [unwired: 11 in]
        n560 = call "GEA2MessageFormatter.vi"("Prefix(Send/Recv)"="SEND", "GEA2 Data In"=w1545, "Error In"=w1546) -> ("Output String"=w1547:string, "Error Out"=w1548:errorcluster)  [unwired: 11 in]
        n561 = call "GExplorer_Queue_GEA2.vi"("Output String"=w1547, "error in (no error)"=w1548) -> ("error out"=w1544:errorcluster)  [unwired: 13 in]
        n562 = call "GEA2 Write ERD.vi"("GEA2 Reference In"=w1535, "GEA Inputs"=w1531, "Write ERD List"=w1543, "Error In"=w1544) -> ("GEA2 Reference Out"=w1540:refnum<k24>, "Error Out"=w1541:errorcluster)  [unwired: 9 in, 1 out]
        n563 = Concatenate Strings("000000000000000000000000" ("string")) -> (w1563:string)
        n564 = Bundle By Name(cluster=T40 {"ERD Number"=61724, "Data Type"=enum."string", "Data"=""} ("ERD Read Data In"), "Data"=w1563) -> (w1561:T40)
        n565 = Build Array(w1561) -> (w1554:T40[])
        n566 = call "Convert Write ERD List to Message.vi"("GEA Inputs"=w1531, "Write ERD List"=w1554, "Error In"=w1541) -> ("GEA Message"=w1556:T10, "Error Out"=w1557:errorcluster)  [unwired: 11 in]
        n567 = call "GEA2MessageFormatter.vi"("Prefix(Send/Recv)"="SEND", "GEA2 Data In"=w1556, "Error In"=w1557) -> ("Output String"=w1558:string, "Error Out"=w1559:errorcluster)  [unwired: 11 in]
        n568 = call "GExplorer_Queue_GEA2.vi"("Output String"=w1558, "error in (no error)"=w1559) -> ("error out"=w1555:errorcluster)  [unwired: 13 in]
        n569 = call "GEA2 Write ERD.vi"("GEA2 Reference In"=w1540, "GEA Inputs"=w1531, "Write ERD List"=w1554, "Error In"=w1555) -> ("GEA2 Reference Out"=w1532:refnum<k24>, "Error Out"=w1534:errorcluster)  [unwired: 9 in, 1 out]
        n570 = call "GEA2 Stop.vi"("GEA2 Reference In"=w1532, "Error In"=w1534) -> ("Error Out"=w1533:errorcluster)  [unwired: 13 in]
      }
      event "Write ERD": Value Change {
        n571 = event-data() -> ()  [unwired: 1 in, 6 out]
        n572 = call "GEA2 Initialize.vi"("Board Index"=w1568, "Source Address"=u8 228, "error in"=w1570) -> ("GeaCommunication.GeaBus"=w1567:refnum<k24>, "error out"=w1569:errorcluster)  [unwired: 10 in, 1 out]
        n573 = Build Array("ERD Write Data In") -> (w1574:T60)
        n574 = call "Convert Write ERD List to Message.vi"("GEA Inputs"=w1573, "Write ERD List"=w1574, "Error In"=w1569) -> ("GEA Message"=w1577:T10, "Error Out"=w1578:errorcluster)  [unwired: 11 in]
        n575 = call "GEA2MessageFormatter.vi"("Prefix(Send/Recv)"="SEND", "GEA2 Data In"=w1577, "Error In"=w1578) -> ("Output String"=w1579:string, "Error Out"=w1580:errorcluster)  [unwired: 11 in]
        n576 = call "GExplorer_Queue_GEA2.vi"("Output String"=w1579, "error in (no error)"=w1580) -> ("error out"=w1575:errorcluster)  [unwired: 13 in]
        n577 = call "GEA2 Write ERD.vi"("GEA2 Reference In"=w1567, "GEA Inputs"=w1573, "Write ERD List"=w1574, "Error In"=w1575, "Verify ERD Response?"=FALSE) -> ("GEA2 Reference Out"=w1564:refnum<k24>, "Error Out"=w1566:errorcluster)  [unwired: 8 in, 1 out]
        n578 = call "GEA2 Stop.vi"("GEA2 Reference In"=w1564, "Error In"=w1566) -> ("Error Out"=w1565:errorcluster)  [unwired: 13 in]
      }
      event "Read ERD": Value Change {
        n579 = event-data() -> ()  [unwired: 1 in, 6 out]
        n580 = call "GEA2 Initialize.vi"("Board Index"=w1587, "Source Address"=u8 228, "error in"=w1589) -> ("GeaCommunication.GeaBus"=w1585:refnum<k24>, "error out"=w1588:errorcluster)  [unwired: 10 in, 1 out]
        n581 = Build Array("ERD Read Data In") -> (w1595:T16[])
        n582 = call "Convert Read ERD List to Message.vi"("GEA Inputs"=w1594, "Read ERD List"=w1595, "Error In"=w1588) -> ("GEA Message"=w1596:T10, "Error Out"=w1591:errorcluster)  [unwired: 11 in]
        n583 = call "GEA2MessageFormatter.vi"("Prefix(Send/Recv)"="SEND", "GEA2 Data In"=w1596, "Error In"=w1591) -> ("Output String"=w1598:string, "Error Out"=w1599:errorcluster)  [unwired: 11 in]
        n584 = call "GExplorer_Queue_GEA2.vi"("Output String"=w1598, "error in (no error)"=w1599) -> ("error out"=w1593:errorcluster)  [unwired: 13 in]
        n585 = call "GEA2 Read ERD.vi"("GeaCommunication.GeaBus"=w1585, "GEA Inputs"=w1594, "Read ERD List"=w1595, "Error In"=w1593, "Verify ERD Response?"=FALSE) -> ("GeaCommunication.GeaBus"=w1584:refnum<k24>, "ERD Data Out"=w1601:T2[], "Error Out"=w1586:errorcluster)  [unwired: 7 in, 1 out]
        n586 = Index Array(array=w1601) -> (element=→"ERD Output":T2)  [unwired: 1 in]
        n587 = call "GEA2 Stop.vi"("GEA2 Reference In"=w1584, "Error In"=w1586) -> ("Error Out"=w1583:errorcluster)  [unwired: 13 in]
      }
      event "Test Mode.Exit Test Mode": Value Change {
        n588 = event-data() -> ()  [unwired: 1 in, 6 out]
        n589 = call "GEA2 Initialize.vi"("Board Index"=w1603, "Source Address"=u8 228, "error in"=w1609) -> ("GeaCommunication.GeaBus"=w1607:refnum<k24>, "error out"=w1608:errorcluster)  [unwired: 10 in, 1 out]
        n590 = Concatenate Strings("00" ("string")) -> (w1621:string)
        n591 = Bundle By Name(cluster=T40 {"ERD Number"=61442, "Data Type"=enum."string", "Data"=""} ("ERD Read Data In"), "Data"=w1621) -> (w1611:T40)
        n592 = Build Array(w1611) -> (w1613:T40[])
        n593 = call "Convert Write ERD List to Message.vi"("GEA Inputs"=w1602, "Write ERD List"=w1613, "Error In"=w1608) -> ("GEA Message"=w1615:T10, "Error Out"=w1616:errorcluster)  [unwired: 11 in]
        n594 = call "GEA2MessageFormatter.vi"("Prefix(Send/Recv)"="SEND", "GEA2 Data In"=w1615, "Error In"=w1616) -> ("Output String"=w1617:string, "Error Out"=w1618:errorcluster)  [unwired: 11 in]
        n595 = call "GExplorer_Queue_GEA2.vi"("Output String"=w1617, "error in (no error)"=w1618) -> ("error out"=w1614:errorcluster)  [unwired: 13 in]
        n596 = call "GEA2 Write ERD.vi"("GEA2 Reference In"=w1607, "GEA Inputs"=w1602, "Write ERD List"=w1613, "Error In"=w1614) -> ("GEA2 Reference Out"=w1604:refnum<k24>, "Error Out"=w1606:errorcluster)  [unwired: 9 in, 1 out]
        n597 = call "GEA2 Stop.vi"("GEA2 Reference In"=w1604, "Error In"=w1606) -> ("Error Out"=w1605:errorcluster)  [unwired: 13 in]
      }
      event Value Change {
        n598 = event-data() -> ()  [unwired: 1 in, 6 out]
        n599 = call "GEA2 Initialize.vi"("Board Index"=w1627, "Source Address"=u8 228, "error in"=w1629) -> ("GeaCommunication.GeaBus"=w1626:refnum<k24>, "error out"=w1628:errorcluster)  [unwired: 10 in, 1 out]
        n600 = property on="Profile Selection" class="DigNum (strict)"(error in=w1628) -> (error out=w1632:errorcluster, "Value"=w1631:u8)  [unwired: 1 in, 1 out]
        n601 = Number To Hexadecimal String(1:i16 2 ("width (-)"), 2:w1631) -> (0:w1633:string)
        n602 = Concatenate Strings("01" ("string"), w1633, "01" ("string")) -> (w1635:string)
        n603 = Bundle By Name(cluster=T40 {"ERD Number"=62234, "Data Type"=enum."string", "Data"=""} ("ERD Read Data In"), "Data"=w1635) -> (w1637:T40)
        n604 = Build Array(w1637) -> (w1645:T40[])
        n605 = call "Convert Write ERD List to Message.vi"("GEA Inputs"=w1622, "Write ERD List"=w1645, "Error In"=w1632) -> ("GEA Message"=w1639:T10, "Error Out"=w1643:errorcluster)  [unwired: 11 in]
        n606 = call "GEA2MessageFormatter.vi"("Prefix(Send/Recv)"="SEND", "GEA2 Data In"=w1639, "Error In"=w1643) -> ("Output String"=w1641:string, "Error Out"=w1642:errorcluster)  [unwired: 11 in]
        n607 = call "GExplorer_Queue_GEA2.vi"("Output String"=w1641, "error in (no error)"=w1642) -> ("error out"=w1644:errorcluster)  [unwired: 13 in]
        n608 = call "GEA2 Write ERD.vi"("GEA2 Reference In"=w1626, "GEA Inputs"=w1622, "Write ERD List"=w1645, "Error In"=w1644) -> ("GEA2 Reference Out"=w1624:refnum<k24>, "Error Out"=w1625:errorcluster)  [unwired: 9 in, 1 out]
        n609 = call "GEA2 Stop.vi"("GEA2 Reference In"=w1624, "Error In"=w1625) -> ("Error Out"=w1623:errorcluster)  [unwired: 13 in]
      }
      event Value Change {
        n610 = event-data() -> ()  [unwired: 1 in, 6 out]
        n611 = call "GEA2 Initialize.vi"("Board Index"=w1652, "Source Address"=u8 228, "error in"=w1655) -> ("GeaCommunication.GeaBus"=w1651:refnum<k24>, "error out"=w1654:errorcluster)  [unwired: 10 in, 1 out]
        n612 = property on="Profile Selection" class="DigNum (strict)"(error in=w1654) -> (error out=w1657:errorcluster, "Value"=w1656:u8)  [unwired: 1 in, 1 out]
        n613 = Number To Hexadecimal String(1:i16 2 ("width (-)"), 2:w1656) -> (0:w1671:string)
        n614 = Concatenate Strings("01" ("string"), w1671, "02" ("string")) -> (w1669:string)
        n615 = Bundle By Name(cluster=T40 {"ERD Number"=62234, "Data Type"=enum."string", "Data"=""} ("ERD Read Data In"), "Data"=w1669) -> (w1667:T40)
        n616 = Build Array(w1667) -> (w1659:T40[])
        n617 = call "Convert Write ERD List to Message.vi"("GEA Inputs"=w1647, "Write ERD List"=w1659, "Error In"=w1657) -> ("GEA Message"=w1665:T10, "Error Out"=w1661:errorcluster)  [unwired: 11 in]
        n618 = call "GEA2MessageFormatter.vi"("Prefix(Send/Recv)"="SEND", "GEA2 Data In"=w1665, "Error In"=w1661) -> ("Output String"=w1663:string, "Error Out"=w1662:errorcluster)  [unwired: 11 in]
        n619 = call "GExplorer_Queue_GEA2.vi"("Output String"=w1663, "error in (no error)"=w1662) -> ("error out"=w1660:errorcluster)  [unwired: 13 in]
        n620 = call "GEA2 Write ERD.vi"("GEA2 Reference In"=w1651, "GEA Inputs"=w1647, "Write ERD List"=w1659, "Error In"=w1660) -> ("GEA2 Reference Out"=w1648:refnum<k24>, "Error Out"=w1650:errorcluster)  [unwired: 9 in, 1 out]
        n621 = call "GEA2 Stop.vi"("GEA2 Reference In"=w1648, "Error In"=w1650) -> ("Error Out"=w1649:errorcluster)  [unwired: 13 in]
      }
      event Value Change {
        n622 = event-data() -> ()  [unwired: 1 in, 6 out]
        n623 = call "GEA2 Initialize.vi"("Board Index"=w1677, "Source Address"=u8 228, "error in"=w1679) -> ("GeaCommunication.GeaBus"=w1676:refnum<k24>, "error out"=w1678:errorcluster)  [unwired: 10 in, 1 out]
        n624 = property on="Profile Selection" class="DigNum (strict)"(error in=w1678) -> (error out=w1682:errorcluster, "Value"=w1681:u8)  [unwired: 1 in, 1 out]
        n625 = Number To Hexadecimal String(1:i16 2 ("width (-)"), 2:w1681) -> (0:w1696:string)
        n626 = Concatenate Strings("01" ("string"), w1696, "03" ("string")) -> (w1694:string)
        n627 = Bundle By Name(cluster=T40 {"ERD Number"=62234, "Data Type"=enum."string", "Data"=""} ("ERD Read Data In"), "Data"=w1694) -> (w1692:T40)
        n628 = Build Array(w1692) -> (w1684:T40[])
        n629 = call "Convert Write ERD List to Message.vi"("GEA Inputs"=w1672, "Write ERD List"=w1684, "Error In"=w1682) -> ("GEA Message"=w1690:T10, "Error Out"=w1686:errorcluster)  [unwired: 11 in]
        n630 = call "GEA2MessageFormatter.vi"("Prefix(Send/Recv)"="SEND", "GEA2 Data In"=w1690, "Error In"=w1686) -> ("Output String"=w1688:string, "Error Out"=w1687:errorcluster)  [unwired: 11 in]
        n631 = call "GExplorer_Queue_GEA2.vi"("Output String"=w1688, "error in (no error)"=w1687) -> ("error out"=w1685:errorcluster)  [unwired: 13 in]
        n632 = call "GEA2 Write ERD.vi"("GEA2 Reference In"=w1676, "GEA Inputs"=w1672, "Write ERD List"=w1684, "Error In"=w1685) -> ("GEA2 Reference Out"=w1673:refnum<k24>, "Error Out"=w1675:errorcluster)  [unwired: 9 in, 1 out]
        n633 = call "GEA2 Stop.vi"("GEA2 Reference In"=w1673, "Error In"=w1675) -> ("Error Out"=w1674:errorcluster)  [unwired: 13 in]
      }
      event Value Change {
        n634 = event-data() -> ()  [unwired: 1 in, 6 out]
        n635 = call "GEA2 Initialize.vi"("Board Index"=w1698, "Source Address"=u8 228, "error in"=w1704) -> ("GeaCommunication.GeaBus"=w1702:refnum<k24>, "error out"=w1703:errorcluster)  [unwired: 10 in, 1 out]
        n636 = property on="Profile Selection" class="DigNum (strict)"(error in=w1703) -> (error out=w1707:errorcluster, "Value"=w1706:u8)  [unwired: 1 in, 1 out]
        n637 = Number To Hexadecimal String(1:i16 2 ("width (-)"), 2:w1706) -> (0:w1708:string)
        n638 = Concatenate Strings("01" ("string"), w1708, "04" ("string")) -> (w1710:string)
        n639 = Bundle By Name(cluster=T40 {"ERD Number"=62234, "Data Type"=enum."string", "Data"=""} ("ERD Read Data In"), "Data"=w1710) -> (w1712:T40)
        n640 = Build Array(w1712) -> (w1720:T40[])
        n641 = call "Convert Write ERD List to Message.vi"("GEA Inputs"=w1697, "Write ERD List"=w1720, "Error In"=w1707) -> ("GEA Message"=w1714:T10, "Error Out"=w1718:errorcluster)  [unwired: 11 in]
        n642 = call "GEA2MessageFormatter.vi"("Prefix(Send/Recv)"="SEND", "GEA2 Data In"=w1714, "Error In"=w1718) -> ("Output String"=w1716:string, "Error Out"=w1717:errorcluster)  [unwired: 11 in]
        n643 = call "GExplorer_Queue_GEA2.vi"("Output String"=w1716, "error in (no error)"=w1717) -> ("error out"=w1719:errorcluster)  [unwired: 13 in]
        n644 = call "GEA2 Write ERD.vi"("GEA2 Reference In"=w1702, "GEA Inputs"=w1697, "Write ERD List"=w1720, "Error In"=w1719) -> ("GEA2 Reference Out"=w1699:refnum<k24>, "Error Out"=w1701:errorcluster)  [unwired: 9 in, 1 out]
        n645 = call "GEA2 Stop.vi"("GEA2 Reference In"=w1699, "Error In"=w1701) -> ("Error Out"=w1700:errorcluster)  [unwired: 13 in]
      }
      event Value Change {
        n646 = event-data() -> ()  [unwired: 1 in, 6 out]
        n647 = call "GEA2 Initialize.vi"("Board Index"=w1723, "Source Address"=u8 228, "error in"=w1729) -> ("GeaCommunication.GeaBus"=w1727:refnum<k24>, "error out"=w1728:errorcluster)  [unwired: 10 in, 1 out]
        n648 = property on="Profile Selection" class="DigNum (strict)"(error in=w1728) -> (error out=w1732:errorcluster, "Value"=w1731:u8)  [unwired: 1 in, 1 out]
        n649 = Number To Hexadecimal String(1:i16 2 ("width (-)"), 2:w1731) -> (0:w1746:string)
        n650 = Concatenate Strings("01" ("string"), w1746, "05" ("string")) -> (w1744:string)
        n651 = Bundle By Name(cluster=T40 {"ERD Number"=62234, "Data Type"=enum."string", "Data"=""} ("ERD Read Data In"), "Data"=w1744) -> (w1742:T40)
        n652 = Build Array(w1742) -> (w1734:T40[])
        n653 = call "Convert Write ERD List to Message.vi"("GEA Inputs"=w1722, "Write ERD List"=w1734, "Error In"=w1732) -> ("GEA Message"=w1740:T10, "Error Out"=w1736:errorcluster)  [unwired: 11 in]
        n654 = call "GEA2MessageFormatter.vi"("Prefix(Send/Recv)"="SEND", "GEA2 Data In"=w1740, "Error In"=w1736) -> ("Output String"=w1738:string, "Error Out"=w1737:errorcluster)  [unwired: 11 in]
        n655 = call "GExplorer_Queue_GEA2.vi"("Output String"=w1738, "error in (no error)"=w1737) -> ("error out"=w1735:errorcluster)  [unwired: 13 in]
        n656 = call "GEA2 Write ERD.vi"("GEA2 Reference In"=w1727, "GEA Inputs"=w1722, "Write ERD List"=w1734, "Error In"=w1735) -> ("GEA2 Reference Out"=w1724:refnum<k24>, "Error Out"=w1726:errorcluster)  [unwired: 9 in, 1 out]
        n657 = call "GEA2 Stop.vi"("GEA2 Reference In"=w1724, "Error In"=w1726) -> ("Error Out"=w1725:errorcluster)  [unwired: 13 in]
      }
      event "Open Lid": Value Change {
        n658 = event-data() -> ()  [unwired: 1 in, 6 out]
        n659 = call "GEA2 Initialize.vi"("Board Index"=w1751, "Source Address"=u8 228, "error in"=w1754) -> ("GeaCommunication.GeaBus"=w1752:refnum<k24>, "error out"=w1753:errorcluster)  [unwired: 10 in, 1 out]
        n660 = case shown="True" "Open Lid" {
          tunnel: w1753 -> [w1761 w1774]
          tunnel: [w1758 w1773] -> w1748
          tunnel: [w1759 w1772] -> w1750
          tunnel: w1752 -> [w1760 w1771]
          tunnel: w1747 -> [w1757 w1770]
          frame False {
            n661 = Build Array(T40 {"ERD Number"=61959, "Data Type"=enum."string", "Data"="01"} ("ERD Read Data In")) -> (w1768:T40[])
            n662 = call "Convert Write ERD List to Message.vi"("GEA Inputs"=w1757, "Write ERD List"=w1768, "Error In"=w1761) -> ("GEA Message"=w1766:T10, "Error Out"=w1765:errorcluster)  [unwired: 11 in]
            n663 = call "GEA2MessageFormatter.vi"("Prefix(Send/Recv)"="SEND", "GEA2 Data In"=w1766, "Error In"=w1765) -> ("Output String"=w1764:string, "Error Out"=w1763:errorcluster)  [unwired: 11 in]
            n664 = call "GExplorer_Queue_GEA2.vi"("Output String"=w1764, "error in (no error)"=w1763) -> ("error out"=w1767:errorcluster)  [unwired: 13 in]
            n665 = call "GEA2 Write ERD.vi"("GEA2 Reference In"=w1760, "GEA Inputs"=w1757, "Write ERD List"=w1768, "Error In"=w1767) -> ("GEA2 Reference Out"=w1758:refnum<k24>, "Error Out"=w1759:errorcluster)  [unwired: 9 in, 1 out]
          }
          frame True {
            n666 = Build Array(T40 {"ERD Number"=61959, "Data Type"=enum."string", "Data"="00"} ("ERD Read Data In")) -> (w1776:T40[])
            n667 = call "Convert Write ERD List to Message.vi"("GEA Inputs"=w1770, "Write ERD List"=w1776, "Error In"=w1774) -> ("GEA Message"=w1778:T10, "Error Out"=w1779:errorcluster)  [unwired: 11 in]
            n668 = call "GEA2MessageFormatter.vi"("Prefix(Send/Recv)"="SEND", "GEA2 Data In"=w1778, "Error In"=w1779) -> ("Output String"=w1780:string, "Error Out"=w1781:errorcluster)  [unwired: 11 in]
            n669 = call "GExplorer_Queue_GEA2.vi"("Output String"=w1780, "error in (no error)"=w1781) -> ("error out"=w1777:errorcluster)  [unwired: 13 in]
            n670 = call "GEA2 Write ERD.vi"("GEA2 Reference In"=w1771, "GEA Inputs"=w1770, "Write ERD List"=w1776, "Error In"=w1777) -> ("GEA2 Reference Out"=w1773:refnum<k24>, "Error Out"=w1772:errorcluster)  [unwired: 9 in, 1 out]
          }
        }
        n671 = call "GEA2 Stop.vi"("GEA2 Reference In"=w1748, "Error In"=w1750) -> ("Error Out"=w1749:errorcluster)  [unwired: 13 in]
      }
      event "Get Faults": Value Change {
        n672 = event-data() -> ()  [unwired: 1 in, 6 out]
        n673 = call "GEA2 Initialize.vi"("Board Index"=w1801, "Source Address"=u8 228, "error in"=w1802) -> ("GeaCommunication.GeaBus"=w1797:refnum<k24>, "error out"=w1796:errorcluster)  [unwired: 10 in, 1 out]
        n674 = call "GEA2 Read ERD Multiple Messages.vi"("GeaCommunication.GeaBus"=w1797, "GEA Inputs"=w1798, "Read ERD List"=T16[] [{"ERD Number"=62483, "Data Type"=enum."string"}, {"ERD Number"=62484, "Data Type"=enum."string"}, {"ERD Number"=62485, "Data Type"=enum."string"}, {"ERD Number"=62486, "Data Type"=enum."string"}, {"ERD Number"=62487, "Data Type"=enum."string"}], "Error In"=w1796, "#ERDs per message"=5) -> ("GeaCommunication.GeaBus"=w1786:refnum<k24>, "ERD Data Out"=w1795:T2[], "Error Out"=w1794:errorcluster)  [unwired: 7 in, 1 out]
        n675 = call "Fault_Table_Read.vi"("ERD Data Out"=w1795, "Error In"=w1794) -> ("Fault Table 0"=→"Fault Entry 0":T32, "Fault Table 1"=→"Fault Entry 1":T32, "Fault Table 2"=→"Fault Entry 2":T32, "Fault Table 3"=→"Fault Entry 3":T32, "Fault Table 4"=→"Fault Entry 4":T32, "Error Out"=w1787:errorcluster)  [unwired: 12 in]
        n676 = call "Fault_Seq_Read.vi"("GEA2 Reference In"=w1786, "Error In"=w1787) -> ("GEA2 Reference Out"=w1783:refnum<k24>, "String"=→"Fault Sequence Buffer":string, "Error Out 2"=w1785:errorcluster)  [unwired: 11 in]
        n677 = call "GEA2 Stop.vi"("GEA2 Reference In"=w1783, "Error In"=w1785) -> ("Error Out"=w1800:errorcluster)  [unwired: 13 in]
      }
      event "Clear Seq": Value Change {
        n678 = event-data() -> ()  [unwired: 1 in, 6 out]
        n679 = property on="Fault Sequence Buffer" class="Str"(error in=w1806, "Value"="") -> (error out=w1805:errorcluster)  [unwired: 1 in, 1 out]
      }
      event "Get Status": Value Change {
        (unwired) 2 ("length (rest)")
        (unwired) 2 ("length (rest)")
        w1846 = T16[] [{"ERD Number"=62468, "Data Type"=enum."string"}] ("Read ERD List")
        n680 = event-data() -> ()  [unwired: 1 in, 6 out]
        n681 = call "GEA2 Initialize.vi"("Board Index"=w1812, "Source Address"=u8 228, "error in"=w1814) -> ("GeaCommunication.GeaBus"=w1811:refnum<k24>, "error out"=w1813:errorcluster)  [unwired: 10 in, 1 out]
        n682 = call "Convert Read ERD List to Message.vi"("GEA Inputs"=w1807, "Read ERD List"=w1846, "Error In"=w1813) -> ("GEA Message"=w1849:T10, "Error Out"=w1850:errorcluster)  [unwired: 11 in]
        n683 = call "GEA2MessageFormatter.vi"("Prefix(Send/Recv)"="SEND", "GEA2 Data In"=w1849, "Error In"=w1850) -> ("Output String"=w1851:string, "Error Out"=w1852:errorcluster)  [unwired: 11 in]
        n684 = call "GExplorer_Queue_GEA2.vi"("Output String"=w1851, "error in (no error)"=w1852) -> ("error out"=w1848:errorcluster)  [unwired: 13 in]
        n685 = call "GEA2 Read ERD.vi"("GeaCommunication.GeaBus"=w1811, "GEA Inputs"=w1807, "Read ERD List"=w1846, "Error In"=w1848) -> ("GeaCommunication.GeaBus"=w1809:refnum<k24>, "ERD Data Out"=w1845:T2[], "Error Out"=w1810:errorcluster)  [unwired: 8 in, 1 out]
        n686 = Index Array(array=w1845) -> (element=w1844:T2)  [unwired: 1 in]
        n687 = call "GEA2 Stop.vi"("GEA2 Reference In"=w1809, "Error In"=w1810) -> ("Error Out"=w1808:errorcluster)  [unwired: 13 in]
        n688 = Unbundle By Name(w1844) -> ("Data"=w1833:string)
        n689 = String Subset(string=w1833, offset (0)=0, length (rest)=2 ("length (rest)")) -> (substring=w1832:string)
        n690 = String Subset(string=w1833, offset (0)=3, length (rest)=2 ("length (rest)")) -> (substring=w1831:string)
        n691 = String Subset(string=w1833, offset (0)=6, length (rest)=2 ("length (rest)")) -> (substring=w1830:string)
        n692 = String Subset(string=w1833, offset (0)=12, length (rest)=2 ("length (rest)")) -> (substring=w1828:string)
        n693 = String Subset(string=w1833, offset (0)=9) -> (substring=w1829:string)  [unwired: 1 in]
        n694 = String Subset(string=w1833, offset (0)=15) -> (substring=w1827:string)  [unwired: 1 in]
        n695 = Concatenate Strings(w1830, w1829) -> (w1825:string)
        n696 = Concatenate Strings(w1832, w1831) -> (w1826:string)
        n697 = Concatenate Strings(w1828, w1827) -> (w1824:string)
        n698 = Hexadecimal String To Number(string=w1826) -> (number=w1822:u32)  [unwired: 2 in, 1 out]
        n699 = Hexadecimal String To Number(string=w1825) -> (number=w1821:u32)  [unwired: 2 in, 1 out]
        n700 = Hexadecimal String To Number(string=w1824) -> (number=w1820:u32)  [unwired: 2 in, 1 out]
        n701 = To Unsigned Word Integer(number=w1822) -> (unsigned 16bit integer=w1818:u16)
        n702 = To Unsigned Word Integer(number=w1821) -> (unsigned 16bit integer=w1817:u16)
        n703 = To Unsigned Word Integer(number=w1820) -> (unsigned 16bit integer=w1816:u16)
        n704 = Bundle By Name(cluster=T31 {"Current Index"=0, "Count"=0, "Overwrite Count"=0} ("Buffer Status"), "Current Index"=w1818, "Count"=w1817, "Overwrite Count"=w1816) -> (→"Seq Buffer Status":T31)
      }
      event "Get Table Status": Value Change {
        w1853 = T16[] [{"ERD Number"=62471, "Data Type"=enum."string"}] ("Read ERD List")
        (unwired) 2 ("length (rest)")
        (unwired) 2 ("length (rest)")
        n705 = event-data() -> ()  [unwired: 1 in, 6 out]
        n706 = call "GEA2 Initialize.vi"("Board Index"=w1860, "Source Address"=u8 228, "error in"=w1862) -> ("GeaCommunication.GeaBus"=w1859:refnum<k24>, "error out"=w1861:errorcluster)  [unwired: 10 in, 1 out]
        n707 = call "Convert Read ERD List to Message.vi"("GEA Inputs"=w1855, "Read ERD List"=w1853, "Error In"=w1861) -> ("GEA Message"=w1895:T10, "Error Out"=w1896:errorcluster)  [unwired: 11 in]
        n708 = call "GEA2MessageFormatter.vi"("Prefix(Send/Recv)"="SEND", "GEA2 Data In"=w1895, "Error In"=w1896) -> ("Output String"=w1897:string, "Error Out"=w1898:errorcluster)  [unwired: 11 in]
        n709 = call "GExplorer_Queue_GEA2.vi"("Output String"=w1897, "error in (no error)"=w1898) -> ("error out"=w1894:errorcluster)  [unwired: 13 in]
        n710 = call "GEA2 Read ERD.vi"("GeaCommunication.GeaBus"=w1859, "GEA Inputs"=w1855, "Read ERD List"=w1853, "Error In"=w1894) -> ("GeaCommunication.GeaBus"=w1857:refnum<k24>, "ERD Data Out"=w1892:T2[], "Error Out"=w1858:errorcluster)  [unwired: 8 in, 1 out]
        n711 = Index Array(array=w1892) -> (element=w1891:T2)  [unwired: 1 in]
        n712 = call "GEA2 Stop.vi"("GEA2 Reference In"=w1857, "Error In"=w1858) -> ("Error Out"=w1856:errorcluster)  [unwired: 13 in]
        n713 = Unbundle By Name(w1891) -> ("Data"=w1880:string)
        n714 = String Subset(string=w1880, offset (0)=0, length (rest)=2 ("length (rest)")) -> (substring=w1879:string)
        n715 = String Subset(string=w1880, offset (0)=3, length (rest)=2 ("length (rest)")) -> (substring=w1878:string)
        n716 = String Subset(string=w1880, offset (0)=6, length (rest)=2 ("length (rest)")) -> (substring=w1877:string)
        n717 = String Subset(string=w1880, offset (0)=12, length (rest)=2 ("length (rest)")) -> (substring=w1875:string)
        n718 = String Subset(string=w1880, offset (0)=9) -> (substring=w1876:string)  [unwired: 1 in]
        n719 = String Subset(string=w1880, offset (0)=15) -> (substring=w1874:string)  [unwired: 1 in]
        n720 = Concatenate Strings(w1877, w1876) -> (w1872:string)
        n721 = Concatenate Strings(w1879, w1878) -> (w1873:string)
        n722 = Concatenate Strings(w1875, w1874) -> (w1871:string)
        n723 = Hexadecimal String To Number(string=w1873) -> (number=w1869:u32)  [unwired: 2 in, 1 out]
        n724 = Hexadecimal String To Number(string=w1872) -> (number=w1868:u32)  [unwired: 2 in, 1 out]
        n725 = Hexadecimal String To Number(string=w1871) -> (number=w1867:u32)  [unwired: 2 in, 1 out]
        n726 = To Unsigned Word Integer(number=w1869) -> (unsigned 16bit integer=w1866:u16)
        n727 = To Unsigned Word Integer(number=w1868) -> (unsigned 16bit integer=w1865:u16)
        n728 = To Unsigned Word Integer(number=w1867) -> (unsigned 16bit integer=w1864:u16)
        n729 = Bundle By Name(cluster=T31 {"Current Index"=0, "Count"=0, "Overwrite Count"=0} ("Buffer Status"), "Current Index"=w1866, "Count"=w1865, "Overwrite Count"=w1864) -> (→"Table Buffer Status":T31)
      }
      event "Clear Fault Buffer": Value Change {
        n730 = event-data() -> ()  [unwired: 1 in, 6 out]
        n731 = call "GEA2 Initialize.vi"("Board Index"=w1905, "Source Address"=u8 228, "error in"=w1906) -> ("GeaCommunication.GeaBus"=w1903:refnum<k24>, "error out"=w1904:errorcluster)  [unwired: 10 in, 1 out]
        n732 = Bundle By Name(cluster=T40 {"ERD Number"=62469, "Data Type"=enum."string", "Data"=""} ("ERD Read Data In"), "Data"="FF") -> (w1916:T40)
        n733 = Build Array(w1916) -> (w1910:T40[])
        n734 = call "Convert Write ERD List to Message.vi"("GEA Inputs"=w1899, "Write ERD List"=w1910, "Error In"=w1904) -> ("GEA Message"=w1912:T10, "Error Out"=w1913:errorcluster)  [unwired: 11 in]
        n735 = call "GEA2MessageFormatter.vi"("Prefix(Send/Recv)"="SEND", "GEA2 Data In"=w1912, "Error In"=w1913) -> ("Output String"=w1914:string, "Error Out"=w1915:errorcluster)  [unwired: 11 in]
        n736 = call "GExplorer_Queue_GEA2.vi"("Output String"=w1914, "error in (no error)"=w1915) -> ("error out"=w1911:errorcluster)  [unwired: 13 in]
        n737 = call "GEA2 Write ERD.vi"("GEA2 Reference In"=w1903, "GEA Inputs"=w1899, "Write ERD List"=w1910, "Error In"=w1911) -> ("GEA2 Reference Out"=w1901:refnum<k24>, "Error Out"=w1902:errorcluster)  [unwired: 9 in, 1 out]
        n738 = call "GEA2 Stop.vi"("GEA2 Reference In"=w1901, "Error In"=w1902) -> ("Error Out"=w1900:errorcluster)  [unwired: 13 in]
      }
      event "Clear Fault Table": Value Change {
        n739 = event-data() -> ()  [unwired: 1 in, 6 out]
        n740 = call "GEA2 Initialize.vi"("Board Index"=w1925, "Source Address"=u8 228, "error in"=w1926) -> ("GeaCommunication.GeaBus"=w1923:refnum<k24>, "error out"=w1924:errorcluster)  [unwired: 10 in, 1 out]
        n741 = Bundle By Name(cluster=T40 {"ERD Number"=62472, "Data Type"=enum."string", "Data"=""} ("ERD Read Data In"), "Data"="FF") -> (w1936:T40)
        n742 = Build Array(w1936) -> (w1930:T40[])
        n743 = call "Convert Write ERD List to Message.vi"("GEA Inputs"=w1919, "Write ERD List"=w1930, "Error In"=w1924) -> ("GEA Message"=w1932:T10, "Error Out"=w1933:errorcluster)  [unwired: 11 in]
        n744 = call "GEA2MessageFormatter.vi"("Prefix(Send/Recv)"="SEND", "GEA2 Data In"=w1932, "Error In"=w1933) -> ("Output String"=w1934:string, "Error Out"=w1935:errorcluster)  [unwired: 11 in]
        n745 = call "GExplorer_Queue_GEA2.vi"("Output String"=w1934, "error in (no error)"=w1935) -> ("error out"=w1931:errorcluster)  [unwired: 13 in]
        n746 = call "GEA2 Write ERD.vi"("GEA2 Reference In"=w1923, "GEA Inputs"=w1919, "Write ERD List"=w1930, "Error In"=w1931) -> ("GEA2 Reference Out"=w1921:refnum<k24>, "Error Out"=w1922:errorcluster)  [unwired: 9 in, 1 out]
        n747 = call "GEA2 Stop.vi"("GEA2 Reference In"=w1921, "Error In"=w1922) -> ("Error Out"=w1920:errorcluster)  [unwired: 13 in]
      }
      event Value Change {
        w1937 = T40[] [{"ERD Number"=62244, "Data Type"=enum."string", "Data"="01"}, {"ERD Number"=61976, "Data Type"=enum."string", "Data"="00 01"}] ("Write ERD List")
        n748 = event-data() -> ()  [unwired: 1 in, 6 out]
        n749 = call "GEA2 Initialize.vi"("Board Index"=w1944, "Source Address"=u8 228, "error in"=w1945) -> ("GeaCommunication.GeaBus"=w1942:refnum<k24>, "error out"=w1943:errorcluster)  [unwired: 10 in, 1 out]
        n750 = call "Convert Write ERD List to Message.vi"("GEA Inputs"=w1938, "Write ERD List"=w1937, "Error In"=w1943) -> ("GEA Message"=w1949:T10, "Error Out"=w1950:errorcluster)  [unwired: 11 in]
        n751 = call "GEA2MessageFormatter.vi"("Prefix(Send/Recv)"="SEND", "GEA2 Data In"=w1949, "Error In"=w1950) -> ("Output String"=w1951:string, "Error Out"=w1952:errorcluster)  [unwired: 11 in]
        n752 = call "GExplorer_Queue_GEA2.vi"("Output String"=w1951, "error in (no error)"=w1952) -> ("error out"=w1948:errorcluster)  [unwired: 13 in]
        n753 = call "GEA2 Write ERD.vi"("GEA2 Reference In"=w1942, "GEA Inputs"=w1938, "Write ERD List"=w1937, "Error In"=w1948) -> ("GEA2 Reference Out"=w1940:refnum<k24>, "Error Out"=w1941:errorcluster)  [unwired: 9 in, 1 out]
        n754 = call "GEA2 Stop.vi"("GEA2 Reference In"=w1940, "Error In"=w1941) -> ("Error Out"=w1939:errorcluster)  [unwired: 13 in]
      }
      event Value Change {
        w1953 = T40[] [{"ERD Number"=62244, "Data Type"=enum."string", "Data"="00"}, {"ERD Number"=61976, "Data Type"=enum."string", "Data"="00 00"}] ("Write ERD List")
        n755 = event-data() -> ()  [unwired: 1 in, 6 out]
        n756 = call "GEA2 Initialize.vi"("Board Index"=w1960, "Source Address"=u8 228, "error in"=w1961) -> ("GeaCommunication.GeaBus"=w1958:refnum<k24>, "error out"=w1959:errorcluster)  [unwired: 10 in, 1 out]
        n757 = call "Convert Write ERD List to Message.vi"("GEA Inputs"=w1954, "Write ERD List"=w1953, "Error In"=w1959) -> ("GEA Message"=w1965:T10, "Error Out"=w1966:errorcluster)  [unwired: 11 in]
        n758 = call "GEA2MessageFormatter.vi"("Prefix(Send/Recv)"="SEND", "GEA2 Data In"=w1965, "Error In"=w1966) -> ("Output String"=w1967:string, "Error Out"=w1968:errorcluster)  [unwired: 11 in]
        n759 = call "GExplorer_Queue_GEA2.vi"("Output String"=w1967, "error in (no error)"=w1968) -> ("error out"=w1964:errorcluster)  [unwired: 13 in]
        n760 = call "GEA2 Write ERD.vi"("GEA2 Reference In"=w1958, "GEA Inputs"=w1954, "Write ERD List"=w1953, "Error In"=w1964) -> ("GEA2 Reference Out"=w1956:refnum<k24>, "Error Out"=w1957:errorcluster)  [unwired: 9 in, 1 out]
        n761 = call "GEA2 Stop.vi"("GEA2 Reference In"=w1956, "Error In"=w1957) -> ("Error Out"=w1955:errorcluster)  [unwired: 13 in]
      }
      event "Stop": Value Change {
        n762 = event-data() -> ()  [unwired: 1 in, 1 out]
        n763 = local write "Exit from SLB"(TRUE ("Exit from SLB")) -> ()
        n764 = call "Control_ERD_Loop.vi"("Command (ERD Loop Control)"=ERD_Loop_Control_Command."Shutdown", "Error In"=w1978) -> ("Error Out"=w1975:errorcluster)  [unwired: 13 in]
        n765 = call "Control_GEA2_Loop.vi"("Command (ERD Loop Control)"=GEA2_Control_Command."Shutdown", "Error In"=w1975) -> ("Error Out"=w1973:errorcluster)  [unwired: 13 in]
        n766 = call "Control_DAQ_Loop.vi"("Command (DAQ Control)"=DAQ_Control_Command."Shutdown", "Error In"=w1973) -> ("Error Out"=w1972:errorcluster)  [unwired: 13 in]
        n767 = call "Control_Continuous_Send_Loop.vi"("Cont Send Loop Control Command"=Cont_Send_Loop_Control_Command."Shutdown", "Error In"=w1972) -> ("Error Out"=w1977:errorcluster)  [unwired: 13 in]
      }
    }
    "UI Loop" <- w680
  }
  n768 = case shown="False" w2 {
    tunnel: w3 -> [w1980 _]
    frame False {
      n769 = while {
        tunnel: w1980 -> [w1981]
        stop <- w1990 stop-if-true
        # "Supplies the updated location for current collection\nin the main caller program"
        n770 = flat-sequence {
          tunnel: ["Record Current Status"] -> w1985
          tunnel: [w1994] -> w1984
          tunnel: w1981 -> [w1992]
          frame #0 {
            n771 = local read "File Locations"() -> (w1994:T39)
            n772 = local read "Washer In"() -> (w1993:T4)
            n773 = call "2015 Filepath Network Variable.vi"("Washer In"=w1993, "Board Index"=w1992, "File Locations"=w1994) -> ()  [unwired: 7 in, 2 out]
          }
        }
        n774 = Unbundle By Name(w1984) -> ("Current (Amps) File"=w1983:path)
        n775 = Path To String(path=w1983) -> (string=w1982:string)
        n776 = shared-variable "My Computer\\Test Lib.lvlib\\Exit"() -> (w1991:bool)  [unwired: 1 in, 1 out]
        n777 = Equal?(x=w1982, y="") -> (x = y?=w1986:bool)
        n778 = And(x=w1986, y=w1985) -> (x .and. y?=w1987:bool)
        n779 = Or(x=w1991, y=w1987) -> (x .or. y?=w1990:bool)
        n780 = Wait Until Next ms Multiple(millisecond multiple="Network Variable Update Rate") -> ()  [unwired: 1 out]
      }
    }
    frame True {
    }
  }
  n781 = while {
    shift-right: [w2003] -> _
    shift-left: _ -> [w2002]
    shift-right: [w2006] -> w22
    shift-left: w12 -> [w2001]
    shift-right: [w2005] -> _
    shift-left: w28 -> [w2007]
    tunnel: w26 -> [w2000]
    tunnel: w25 -> [w1999]
    tunnel: w3 -> [w1998]
    tunnel: w23 -> [w1996]
    stop <- w2004 stop-if-true
    # "Save File Loop"
    n782 = local read "Sample Rate (ms)"() -> (w1997:u32)
    n783 = call <vilib>:"Parse State Queue__jki_lib_state_machine.vi"("State Queue"=w2007, "Error In (no error)"=w2001) -> ("Remaining States"=w2009:string, "Current State"=w2010:string, "Arguments"=w2008:string)  [unwired: 11 in]
    n784 = case shown="\"Check File Name\"" w2010 {
      selector: w2010 -> [_ _ w2050 _ _ _ _ _ _ _ _ _ _ _ _ _ _ _ _ _ _ _]
      tunnel: w2009 -> [w2017 w2049 w2054 w2072 w2078 w2083 w2087 w2099 w2108 w2112 w2121 w2127 w2138 w2181 w2186 w2196 w2200 w2224 w2240 w2263 w2274 w2305]
      tunnel: w2008 -> [_ _ _ _ _ _ _ _ _ _ _ w2122 w2132 _ _ _ _ _ _ _ _ _]
      tunnel: w2002 -> [w2015 w2046 w2052 w2063 w2075 w2081 w2084 _ w2103 w2109 w2117 w2125 w2136 w2178 w2183 w2193 w2197 w2216 w2233 w2254 w2282 w2302]
      tunnel: [w2014 w2047 w2056 w2069 errorcluster {"status"=FALSE, "code"=0, "source"=""} ("error out") w2080 w2085 w2092 w2104 w2110 w2113 w2123 w2134 w2179 w2184 w2194 w2198 w2217 w2237 w2258 w2281 w2303] -> w2006
      tunnel: w2001 -> [w2013 w2047 w2055 w2069 w2074 w2080 w2085 w2093 w2105 w2110 w2114 w2124 w2133 w2179 w2184 w2194 w2198 w2222 w2238 w2253 w2281 w2304]
      tunnel: [w2016 w2048 w2053 w2071 w2077 w2082 w2086 w2098 w2107 w2111 w2120 w2126 w2137 w2180 w2185 w2195 w2199 w2223 w2239 w2262 w2283 w2308] -> w2005
      tunnel: [_ _ _ _ _ TRUE _ _ _ _ _ _ _ _ _ _ _ _ _ _ _ _] -> w2004
      tunnel: [w2012 w2046 w2052 w2070 w2075 w2081 w2084 w2097 w2103 w2109 w2116 w2125 w2136 w2178 w2183 w2193 w2197 w2221 w2230 w2257 w2282 w2302] -> w2003
      tunnel: w1997 -> [w2011 _ _ _ _ _ _ _ _ _ _ _ _ _ _ _ _ _ _ _ _ _]
      tunnel: w2000 -> [_ _ _ _ _ _ _ w2095 _ _ _ _ _ _ _ _ _ _ _ _ _ _]
      tunnel: w1999 -> [_ _ _ _ _ _ _ w2094 _ _ _ _ _ _ _ _ _ _ _ _ _ _]
      tunnel: w1998 -> [_ _ _ _ _ _ _ _ _ _ _ _ _ _ _ _ _ _ _ w2261 _ _]
      tunnel: w1996 -> [_ _ _ _ _ _ _ _ _ _ _ _ _ _ _ _ _ _ _ w2251 _ _]
      frame "", "Idle" {
        n785 = event shown="[0] Timeout" {
          selector: _ -> [_ _ _]
          dyn-events: _ -> [_ _ _]
          timeout: w2011 -> [_ _ _]
          tunnel: w2017 -> [w2023 w2034 w2045]
          tunnel: [w2022 w2034 w2044] -> w2016
          tunnel: w2015 -> [w2020 w2026 w2042]
          tunnel: [w2021 w2027 w2036] -> w2014
          tunnel: w2013 -> [w2021 w2028 w2035]
          tunnel: [w2020 w2026 w2042] -> w2012
          event Timeout {
            n786 = event-data() -> ()  [unwired: 1 in, 1 out]
            n787 = case shown="False" "Disable Write" {
              tunnel: ["Check File Name\nWrite Data\nCheck Timer\nOpen Front Panel" ("State(s) in Front (\"\")") "Open Front Panel" ("State(s) in Front (\"\")")] -> w2019
              frame False {
              }
              frame True {
              }
            }
            n788 = call <vilib>:"Add State(s) to Queue__jki_lib_state_machine.vi"("State(s) in Front (\"\")"=w2019, "State(s) in (\"\")"=w2023) -> ("States Out"=w2022:string)  [unwired: 13 in]
          }
          event "Minimize": Value Change {
            n789 = event-data() -> ()  [unwired: 1 in, 6 out]
            n790 = Unbundle By Name(w2026) -> ("Core.Current VI Reference"=w2033:refnum<vi>)
            n791 = invoke class="VI" method="FP.Open"(reference=w2033, error in=w2028, "Activate"=TRUE ("Activate?"), "State"=T61."Hidden") -> (reference out=w2029:refnum<vi>, error out=w2030:errorcluster)  [unwired: 1 in, 3 out]
            n792 = Close Reference(reference=w2029, error in (no error)=w2030) -> (error out=w2027:errorcluster)
          }
          event Panel Close? {
            # "Close Panel button (pressed) Event\nThis minimizes the window"
            n793 = event-data() -> ()  [unwired: 1 in, 1 out]
            n794 = Unbundle By Name(w2042) -> ("Core.Current VI Reference"=w2041:refnum<vi>)
            n795 = invoke class="VI" method="FP.Open"(reference=w2041, error in=w2035, "Activate"=TRUE ("Activate?"), "State"=T61."Hidden") -> (reference out=w2037:refnum<vi>, error out=w2038:errorcluster)  [unwired: 1 in, 3 out]
            n796 = Close Reference(reference=w2037, error in (no error)=w2038) -> (error out=w2036:errorcluster)
            n797 = event-data() -> ()  [unwired: 2 in, 1 out]
            n798 = call <vilib>:"Add State(s) to Queue__jki_lib_state_machine.vi"("State(s) in Front (\"\")"="", "State(s) in (\"\")"=w2045) -> ("States Out"=w2044:string)  [unwired: 13 in]
          }
        }
      }
      frame "---------- Core ----------" {
        # "Do not put any code in this frame.\n(it is a separator no-op)"
        n799 = call <vilib>:"Add State(s) to Queue__jki_lib_state_machine.vi"("State(s) in (\"\")"=w2049) -> ("States Out"=w2048:string)  [unwired: 14 in]
      }
      frame Default {
        w2059 = 42 items=["No error", "Argument error", "Memory is full", "Out of zone", "End of file", "File already open", "Generic file I/O error", "File not found", "File permission error", "Disk is full", "Duplicate path", "Too many files open", "System feature not enabled", "Resource file not found", "Cannot add resource", "Resource not found", "Image not found", "Image memory error", "Pen does not exist", "Config type invalid", "Config token not found", "Config parse error", "Config memory error", "Bad external code format", "Bad external code offset", "External code not present", "Null window", "Destroy window error", "Null menu", "Print aborted", "Bad print record", "Print driver error", "Windows error during printing", "Memory error during printing", "Print dialog error", "Generic print error", "Invalid device refnum", "Device not found", "Device parameter error", "Device unit error", "Cannot open device", "Device call aborted", "Generic error", "Cancelled by user", "Object ID too low", "Object ID too high", "Object not in heap", "Unknown heap", "Unknown object (invalid DefProc)", "Unknown object (DefProc not in table)", "Message out of range", "Invalid (null) method", "Unknown message", "Manager call not supported", "Bad address", "Network operation in progress", "Network operation timed out", "Connection is busy", "Network attribute not supported", "Network error", "Address in use", "System out of memory", "Connection aborted", "Connection refused", "Not connected", "Already connected", "Connection closed", "Initialization error (interapplication manager)", "Bad occurrence", "Wait on unbound occurrence handler", "Occurrence queue overflow", "Datalog type conflict", "Unused", "Unrecognized type (interapplication manager)", "Memory corrupt", "Failed to make temporary DLL", "Old CIN version", "Drag socket not found", "Failed to load drop-object", "Failed to register OLE object", "Failed to release OLE object", "Format specifier type mismatch", "Unknown format specifier", "Too few format specifiers", "Too many format specifiers", "Scan failed", "Newer CIN version", "Error converting to variant", "Runtime menu error", "Password tampered", "Variant attribute not found", "Incompatible variant data type", "Event data is not available", "Event Store is not present", "Occurrence is not found", "Event Queue is not created", "Event info is not available", "Refnum passed is NULL", "Error retrieving Class GUID", "Error retrieving CoClass GUID", "Error retrieving TypeLib GUID.", "Bad built application magic bytes.", "Specific driver is different from the specific driver associated with the Logical Name.", "There is no session opened to the class driver.", "Max Error", "MAX - Error with config objects", "MAX - Error loading configuration", "MAX - Group not supported"]
        # "Current State"
        # "Do not delete, rename, or modify this frame.\n(this is used to capture unhandled states and typos)"
        # "Handle mistyped state name (developer tool)"
        n800 = Format Into String(format string="Software Exception: Unhandled State \"%s\"." ("message"), error in=w2055, w2050) -> (resulting string=w2058:string, error out=w2057:errorcluster)  [unwired: 1 in]
        n801 = call <vilib>:"Error Cluster From Error Code.vi"("show call chain? (False)"=TRUE, "error in (no error)"=w2057, "error message (\"\")"=w2058, "error code (0)"=w2059) -> ("error out"=w2056:errorcluster)  [unwired: 5 in]
        n802 = call <vilib>:"Add State(s) to Queue__jki_lib_state_machine.vi"("State(s) in (\"\")"=w2054) -> ("States Out"=w2053:string)  [unwired: 14 in]
      }
      frame "Initialize Core Data" {
        # "Do not delete, rename, or modify this frame.\n(this is used to determine panel behavior on exit)"
        # "originally closed?"
        # "exe?"
        # "If panel starts closed or is an EXE, then close it when we exit"
        n803 = property class="VI"() -> ("Front Panel.Open"=w2068:bool)  [unwired: 2 in, 2 out]
        n804 = property class="App"() -> ("App.Kind"=w2067:T62)  [unwired: 2 in, 2 out]
        n805 = control-ref of="Current VI Reference"() -> (w2061:refnum<vi>)
        n806 = Not(x=w2068) -> (.not. x?=w2065:bool)
        n807 = Equal?(x=w2067, y=T62."Run Time System" ("Application:Kind")) -> (x = y?=w2064:bool)
        n808 = Or(x=w2065, y=w2064) -> (x .or. y?=w2062:bool)
        n809 = Bundle By Name(cluster=w2063, "Core.Current VI Reference"=w2061, "Core.Close Panel on Exit?"=w2062) -> (w2070:T64)
        n810 = call <vilib>:"Add State(s) to Queue__jki_lib_state_machine.vi"("State(s) in (\"\")"=w2072) -> ("States Out"=w2071:string)  [unwired: 14 in]
      }
      frame "Error Handler" {
        # "Unhandled Error -- Display it"
        # "Handle any errors here.\nYou can also output any states to clean-up after errors occur"
        # "Clear error"
        n811 = call <vilib>:"General Error Handler.vi"("error in (no error)"=w2074) -> ()  [unwired: 10 in, 5 out]
        n812 = call <vilib>:"Add State(s) to Queue__jki_lib_state_machine.vi"("State(s) in Front (\"\")"="/* Post Error States", "State(s) in (\"\")"=w2078) -> ("States Out"=w2077:string)  [unwired: 13 in]
      }
      frame "Exit" {
        # "Do not put any code in this frame.\n(No errors that occur here will be handled.)"
        n813 = call <vilib>:"Add State(s) to Queue__jki_lib_state_machine.vi"("State(s) in (\"\")"=w2083) -> ("States Out"=w2082:string)  [unwired: 14 in]
      }
      frame "---------- Data ----------" {
        # "Do not put any code in this frame.\n(It is a separator no-op. You can make a copy of this frame to create a new Data frame)"
        n814 = call <vilib>:"Add State(s) to Queue__jki_lib_state_machine.vi"("State(s) in (\"\")"=w2087) -> ("States Out"=w2086:string)  [unwired: 14 in]
      }
      frame "Data: Initialize" {
        w2088 = T1 {"Basket Speed (RPM)"=0, "Machine State"="", "Tub Volume (Gal)"=0.0, "Pressure (inches H20)"=0.0, "Lid Switch "=FALSE, "Current RMS (Amps)"=0.0, "Cycle Selected"="", "Lid Lock Status"="", "Mode Shift Status"="", "Spray/Rinse Valve"=FALSE, "Fabric Soft Valve"=FALSE, "Drain Pump"=FALSE, "Recirc. Pump"=FALSE, "Cycle Engine State"="", "Hot  Water Valve"=FALSE, "Cold Water Valve"=FALSE, "Motor Profile"="", "Motor Profile Status"="", "Motor Mode"="", "ME Relay"=FALSE, "Cycle Count"=0, "Deep Rinse / FS"=FALSE, "My Cycle"=FALSE, "Soil Level"="", "Spin Level"="", "Stain"="", "Temp Level"="", "Load Size"="", "Delay Time"=0, "Soak Time"=0, "Deep Fill"=FALSE, "Warm Rinse"=FALSE, "Auto Soak Level"="", "Extra Rinse"=FALSE, "Wet Load Gallons"=0.0, "Target Galllons"=0.0, "Sub-Cycle"="", "Load Type"="", "Target Level (inches)"=0, "Valve Relay"=FALSE, "Dry Load Size"=0.0, "Shaft Speed (RPM) "=0, "MS Motor"=FALSE, "Mode Shift FB"=FALSE, "Target Bath Temp (F)"=0.0, "Temperature (F)"=0.0, "Current Bath Temp (F)"=0.0, "Lid Lock FB"="", "Lid Lock Req State"="", "Remaining Cycle Time (s)"=0.0, "Serial Number"=""}  # ERD Data Save
        w2091 = refnum<file> refnum  # File Refnum
        w2096 = T65 {"Current VI Reference"=refnum, "Close Panel on Exit?"=FALSE}  # Core
        # "Wait until everything initializes and the GEA2 is running"
        n815 = while {
          tunnel: w2093 -> [w2100]
          tunnel: [w2100] -> w2092
          stop <- w2102 stop-if-true
          n816 = local read "Start Save Routine"() -> (w2102:bool)
          n817 = Wait Until Next ms Multiple(millisecond multiple=u32 100) -> ()  [unwired: 1 out]
        }
        n818 = Bundle("Core"=w2096, "File Locations"=w2094, "Washer In"=w2095, "File Refnum"=w2091, "FileVersionInfo"="FileVersionInfo", "2015 Cycle Stats"="2015 Cycle Stats", "ERD Data Save"=w2088) -> (w2097:T64)  [unwired: 1 in]
        n819 = call <vilib>:"Add State(s) to Queue__jki_lib_state_machine.vi"("State(s) in (\"\")"=w2099) -> ("States Out"=w2098:string)  [unwired: 14 in]
      }
      frame "Data: Cleanup" {
        # "Cleanup any data and references, here.\n(this is called automatically, by the Macro: Exit)"
        n820 = Unbundle By Name(w2103) -> ("Core.Current VI Reference"=w2106:refnum<vi>)
        n821 = Close Reference(reference=w2106, error in (no error)=w2105) -> (error out=w2104:errorcluster)
        n822 = call <vilib>:"Add State(s) to Queue__jki_lib_state_machine.vi"("State(s) in (\"\")"=w2108) -> ("States Out"=w2107:string)  [unwired: 14 in]
      }
      frame "---------- UI ----------" {
        # "Do not put any code in this frame.\n(It is a separator no-op. You can make a copy of this frame to create a new UI frame)"
        n823 = call <vilib>:"Add State(s) to Queue__jki_lib_state_machine.vi"("State(s) in (\"\")"=w2112) -> ("States Out"=w2111:string)  [unwired: 14 in]
      }
      frame "UI: Initialize" {
        # "Initialize the User Interface, here.\n(this is called automatically, by the Macro: Init)"
        n824 = Current VI's Path() -> (path=w2118:path)
        "Exe Path" <- w2118
        n825 = call "UTILITY This VIs Path.vi"("path"=w2118, "error in (no error)"=w2114) -> ("FileVersionInfo Out"=w2115:T6, "error out"=w2113:errorcluster)  [unwired: 7 in, 5 out]
        "FileVersionInfo Out" <- w2115
        n826 = Unbundle By Name(w2115) -> ("FileVersion"=→"Description 4":string)
        n827 = Bundle By Name(cluster=w2117, "FileVersionInfo"=w2115) -> (w2116:T64)
        n828 = call <vilib>:"Add State(s) to Queue__jki_lib_state_machine.vi"("State(s) in (\"\")"=w2121) -> ("States Out"=w2120:string)  [unwired: 14 in]
      }
      frame "UI: Cursor Set" {
        # "Argument"
        # "Set and Unset Cursor Busy.\n(Usage: \"UI: Cursor Set >> Busy|Idle\")"
        n829 = case shown="\"Idle\", Default" w2122 {
          tunnel: w2124 -> [w2129 w2131]
          tunnel: [w2128 w2130] -> w2123
          frame "Idle", Default {
            n830 = call <vilib>:"Unset Busy.vi"("error in (no error)"=w2129) -> ("error out"=w2128:errorcluster)  [unwired: 10 in]
          }
          frame "Busy" {
            n831 = call <vilib>:"Set Busy.vi"("error in (no error)"=w2131) -> ("error out"=w2130:errorcluster)  [unwired: 9 in, 1 out]
          }
        }
        n832 = call <vilib>:"Add State(s) to Queue__jki_lib_state_machine.vi"("State(s) in (\"\")"=w2127) -> ("States Out"=w2126:string)  [unwired: 14 in]
      }
      frame "UI: Front Panel State" {
        # "Argument"
        # "Set Front Panel Open or Closed\n(Usage: \"UI: Front Panel State >> Open|Close\")"
        n833 = Unbundle By Name(w2136) -> ("Core.Current VI Reference"=w2135:refnum<vi>)
        n834 = case shown="\"Open\", Default" w2132 {
          tunnel: w2133 -> [w2142 w2172]
          tunnel: [w2144 w2173] -> w2134
          tunnel: w2135 -> [w2143 w2170]
          frame "Open", Default {
            n835 = property class="VI"(reference=w2143, error in=w2142) -> (reference out=w2140:refnum<vi>, error out=w2141:errorcluster, "Front Panel.Open"=w2139:bool)
            n836 = case shown="False" w2139 {
              tunnel: [w2154 w2161] -> w2144
              tunnel: w2141 -> [w2159 w2165]
              tunnel: w2140 -> [w2160 w2164]
              frame False {
                w2151 = 0 items=["NULL"]
                # "Windows API to bring the LaundrySLB.vi screen\nto the front. It also allows you to rename the vi, therefore\nbeing a dynamic file name. (You have to rename for\nit to work)"
                n837 = Current VI's Path() -> (path=w2150:path)
                n838 = Open VI Reference(vi path=w2150) -> (vi reference=w2149:refnum<vi>, error out=w2146:errorcluster)  [unwired: 5 in]
                n839 = property class="VI"(reference=w2149, error in=w2146) -> (reference out=w2148:refnum<vi>, error out=w2147:errorcluster, "Name"=w2145:string)
                n840 = Close Reference(reference=w2148, error in (no error)=w2147) -> ()  [unwired: 1 out]
                n841 = dll-call lib="user32.dll" fn="FindWindowA" label="FindWindow"("lpszClassName"=w2151, "lpszWindowName"=w2145) -> ("hWnd"=w2152:u32)  [unwired: 4 in, 3 out]
                "Handle" <- w2152
                n842 = dll-call lib="user32.dll" fn="SetForegroundWindow"("Handle"=w2152) -> (→"Error":i32)  [unwired: 4 in, 2 out]
                n843 = invoke class="VI" method="FP.Open"(reference=w2160, error in=w2159, "Activate"=TRUE ("Activate?"), "State"=T61."Maximized") -> (reference out=w2157:refnum<vi>, error out=w2158:errorcluster)  [unwired: 1 in, 3 out]
                n844 = Close Reference(reference=w2157, error in (no error)=w2158) -> (error out=w2154:errorcluster)
              }
              frame True {
                n845 = invoke class="VI" method="FP.Open"(reference=w2164, error in=w2165, "Activate"=TRUE, "State"=T61."Maximized") -> (reference out=w2163:refnum<vi>, error out=w2162:errorcluster)  [unwired: 1 in, 3 out]
                n846 = Close Reference(reference=w2163, error in (no error)=w2162) -> (error out=w2161:errorcluster)
              }
            }
          }
          frame "Close" {
            n847 = property class="VI"(reference=w2170, error in=w2172) -> (reference out=w2169:refnum<vi>, error out=w2171:errorcluster, "Front Panel.Open"=w2168:bool)
            n848 = case shown="True" w2168 {
              tunnel: [w2174 w2177] -> w2173
              tunnel: w2171 -> [w2174 w2176]
              tunnel: w2169 -> [_ w2175]
              frame False {
              }
              frame True {
                n849 = invoke class="VI" method="FP.Close"(reference=w2175, error in=w2176) -> (error out=w2177:errorcluster)  [unwired: 1 in, 2 out]
              }
            }
          }
        }
        n850 = call <vilib>:"Add State(s) to Queue__jki_lib_state_machine.vi"("State(s) in (\"\")"=w2138) -> ("States Out"=w2137:string)  [unwired: 14 in]
      }
      frame "---------- Macro ----------" {
        # "Do not put any code in this frame.\n(It is a separator no-op. You can make a copy of this frame to create a new Macro frame)"
        n851 = call <vilib>:"Add State(s) to Queue__jki_lib_state_machine.vi"("State(s) in (\"\")"=w2181) -> ("States Out"=w2180:string)  [unwired: 14 in]
      }
      frame "Macro: Initialize" {
        w2182 = "Data: Initialize\nInitialize Core Data\nUI: Initialize\nUI: Front Panel State >> Open"  # Data: Initialize Initialize Core Data UI: Initialize UI: Front Panel State >> Open
        # "Initialization Macro\n(This is called once, when the VI starts)"
        n852 = call <vilib>:"Add State(s) to Queue__jki_lib_state_machine.vi"("State(s) in Front (\"\")"=w2182, "State(s) in (\"\")"=w2186) -> ("States Out"=w2185:string)  [unwired: 13 in]
      }
      frame "Macro: Exit" {
        # "Exit Macro\n(This is called once, when the VI exits)"
        n853 = Unbundle By Name(w2193) -> ("Core.Close Panel on Exit?"=w2192:bool)
        n854 = Select(t="UI: Front Panel State >> Close", s=w2192, f="") -> (s? t:f=w2189:string)
        n855 = call <vilib>:"Add State(s) to Queue__jki_lib_state_machine.vi"("State(s) in (\"\")"=w2189, "State(s) at Back (\"\")"="Data: Cleanup\nExit") -> ("States Out"=w2187:string)  [unwired: 13 in]
        n856 = call <vilib>:"Add State(s) to Queue__jki_lib_state_machine.vi"("State(s) in Front (\"\")"=w2187, "State(s) in (\"\")"=w2196) -> ("States Out"=w2195:string)  [unwired: 13 in]
      }
      frame "---------- New Category ----------" {
        # "Template Separator\n(You can make a copy of, or modify, this frame)"
        n857 = call <vilib>:"Add State(s) to Queue__jki_lib_state_machine.vi"("State(s) in (\"\")"=w2200) -> ("States Out"=w2199:string)  [unwired: 14 in]
      }
      frame "Check File Name" {
        # "Write the summary stats"
        # "Only publish a new filename if\nnecessary"
        n858 = Unbundle By Name(w2216) -> ("File Refnum"=w2207:refnum<file>, "2015 Cycle Stats"=w2205:T3, "File Locations"=w2213:T39, "Washer In"=w2211:T4)
        n859 = Unbundle By Name(w2211) -> ("Washer Details.Serial Number:"=→"Washer Details.Serial Number:":string, "Washer Details.TR Number:"=→"Washer Details.TR Number:":string, "Washer Details.Lab ID:"=→"Washer Details.Lab ID:":string)
        n860 = local read "ERD Data"() -> (w2201:T1)
        n861 = Unbundle By Name(w2201) -> ("Cycle Count"=w2219:u32)
        n862 = call "Save File Format All Folders.vi"("Total Cycle Count"=w2219, "Number of Cycles/ File"="Number of Cycles/ File", "error in (no error)"=w2222, "Initialize.Washer In"=w2211, "File Locations Old"=w2213) -> ("error out"=w2215:errorcluster, "New File?"=w2206:bool, "File Path Output New"=w2212:T39)  [unwired: 3 in, 1 out]
        "New File?" <- w2206
        n863 = local read "Cycle Timer"() -> (w2204:dbl)
        n864 = call "2015 RunTime Summary.vi"("Cycle Timer"=w2204, "ERD Data"=w2201, "2015 Cycle Stats"=w2205, "error in (no error)"=w2215, "New File?"=w2206, "File Locations"=w2213) -> ("error out"=w2214:errorcluster, "New File?Out"=w2203:bool, "2015 Cycle Stats Out"=w2202:T3)  [unwired: 3 in]
        n865 = Bundle By Name(cluster=w2216, "File Locations"=w2212, "2015 Cycle Stats"=w2202, "ERD Data Save"=w2201) -> (w2221:T64)
        n866 = local write "2015 Cycle Stats"(w2202) -> ()
        n867 = call "2015 Open Close Reference.vi"("Byte Stream File in"=w2207, "error in (no error)"=w2214, "New File?"=w2203) -> ("error out"=w2217:errorcluster, "String"=w2218:string)  [unwired: 7 in]
        n868 = call <vilib>:"Add State(s) to Queue__jki_lib_state_machine.vi"("State(s) in Front (\"\")"=w2218, "State(s) in (\"\")"=w2224) -> ("States Out"=w2223:string)  [unwired: 13 in]
      }
      frame "Write Data" {
        # "Save the data to file"
        n869 = local read "Redundant Micro"() -> (w2235:T33)
        n870 = Unbundle By Name(w2233) -> ("ERD Data Save"=w2225:T1, "File Refnum"=w2234:refnum<file>)
        n871 = local read "Version"() -> (w2236:T11)
        n872 = Unbundle By Name(w2225) -> ("Cycle Count"=w2232:u32, "Basket Speed (RPM)"=w2231:u16, "Machine State"=w2228:string)
        n873 = call "Write_ERD_Data_to_File.vi"("refnum in"=w2234, "ERD_Always Show"=w2225, "Redundant Micro"=w2235, "Version"=w2236, "Error In"=w2238) -> ("refnum out"=w2226:refnum<file>, "Error Out"=w2237:errorcluster)  [unwired: 9 in]
        n874 = case shown="\"STANDBY\"" w2228 {
          tunnel: [u32 14927872 ("Pause 2") u32 14927872 ("Pause 2") u32 14927872 ("Pause 2") u32 6334743 ("Run 2") u32 14927872 ("Pause 2") u32 14927872 ("Pause 2") u32 20719 ("EOC")] -> w2227
          frame "IDLE", Default {
          }
          frame "STANDBY" {
          }
          frame "DELAY" {
          }
          frame "RUN" {
          }
          frame "PAUSE" {
          }
          frame "DELAY PAUSE" {
          }
          frame "EOC" {
          }
        }
        n875 = Bundle By Name(cluster=w2233, "Washer In.Day Cycle Count"=w2232, "Washer In.RPM"=w2231, "File Refnum"=w2226, "Washer In.Status Color"=w2227) -> (w2230:T64)
        n876 = Unbundle By Name(w2230) -> ("Washer In"=→"Washer In":T4)
        n877 = call <vilib>:"Add State(s) to Queue__jki_lib_state_machine.vi"("State(s) in (\"\")"=w2240) -> ("States Out"=w2239:string)  [unwired: 14 in]
      }
      frame "Publish Filename" {
        # "Get the latest ref"
        # "Publish the filenames to the network variable. Only need\nto do when there is a new file name."
        n878 = Unbundle By Name(w2254) -> ("File Locations"=w2249:T39, "Washer In"=w2250:T4)
        n879 = case shown="False" "Disable Read Previous" {
          tunnel: w2253 -> [w2268 w2269]
          tunnel: [w2267 w2269] -> w2252
          tunnel: w2251 -> [w2266 _]
          tunnel: w2250 -> [w2264 _]
          frame False {
            n880 = call "HCC Read Write Display.vi"("Read Write Control"=T63."Write 2015", "error in (no error)"=w2268, "Washer Input"=w2264, "Configuration File Path in"=w2266) -> ("error out"=w2267:errorcluster)  [unwired: 6 in, 1 out]
          }
          frame True {
          }
        }
        n881 = local write "File Locations"(w2249) -> ()
        n882 = call "2015 Filepath Network Variable.vi"("Washer In"=w2250, "error in (no error)"=w2252, "Board Index"=w2261, "File Locations"=w2249) -> ("error out"=w2259:errorcluster, "File Locations Output"=w2255:T39)  [unwired: 6 in]
        n883 = Unbundle By Name(w2255) -> ("Log Inverter File"=w2260:path)
        n884 = call "Write Header.vi"("File Path Control"=w2260, "Error In"=w2259) -> ("refnum out"=w2256:refnum<file>, "Error Out"=w2258:errorcluster)  [unwired: 12 in]
        n885 = call <vilib>:"Add State(s) to Queue__jki_lib_state_machine.vi"("State(s) in (\"\")"=w2263) -> ("States Out"=w2262:string)  [unwired: 14 in]
        n886 = Bundle By Name(cluster=w2254, "File Refnum"=w2256) -> (w2257:T64)
      }
      frame "Open Front Panel" {
        # "If the exit button is pressed\nin the SLB program. Go ahead\nand shut down"
        # "Checks the network variable to see if the user wants to open or exit the\napplication."
        n887 = local read "Exit from SLB"() -> (w2271:bool)
        n888 = Unbundle By Name(w2282) -> ("Washer In.Board ID"=w2276:string)
        n889 = shared-variable ".\\Test Lib.lvlib\\Board ID"() -> (w2279:string)  [unwired: 1 in, 1 out]
        n890 = shared-variable "My Computer\\Test Lib.lvlib\\Exit"() -> (w2272:bool)  [unwired: 1 in, 1 out]
        n891 = Or(x=w2272, y=w2271) -> (x .or. y?=w2270:bool)
        n892 = call <vilib>:"Trim Whitespace.vi"("string"=w2279) -> ("trimmed string"=w2278:string)  [unwired: 1 in]
        n893 = Equal?(x=w2276, y=w2278) -> (x = y?=w2277:bool)
        n894 = case shown="True" w2270 {
          selector: w2270 -> [_ w2285]
          tunnel: ["" "Macro: Exit"] -> w2280
          frame False {
          }
          frame True {
            n895 = property on="Stop" class="Bool (strict)"("Val(Sgnl)"=w2285) -> ()  [unwired: 2 in, 2 out]
          }
        }
        n896 = case shown="True" w2277 {
          tunnel: ["" w2289] -> w2275
          frame False {
          }
          frame True {
            w2289 = "UI: Front Panel State >> Open"  # UI: Front Panel State >> Open
            n897 = shared-variable ".\\Test Lib.lvlib\\Board ID"("") -> ()  [unwired: 1 in, 1 out]
          }
        }
        n898 = call <vilib>:"Add State(s) to Queue__jki_lib_state_machine.vi"("State(s) in Front (\"\")"=w2280, "State(s) in (\"\")"=w2274) -> ("States Out"=w2273:string)  [unwired: 13 in]
        n899 = call <vilib>:"Add State(s) to Queue__jki_lib_state_machine.vi"("State(s) in Front (\"\")"=w2275, "State(s) in (\"\")"=w2273) -> ("States Out"=w2283:string)  [unwired: 13 in]
      }
      frame "Check Timer" {
        n900 = Unbundle By Name(w2302) -> ("2015 Cycle Stats.Cycle Time (Minutes)"=w2301:dbl, "2015 Cycle Stats.Max Temp"=w2300:dbl, "2015 Cycle Stats.Max Basket Speed"=w2299:dbl, "2015 Cycle Stats.Max Motor Current"=w2298:dbl, "2015 Cycle Stats.Max Tub Volume"=w2297:dbl, "2015 Cycle Stats.Max Pressure (H2O)"=w2296:dbl, "2015 Cycle Stats.Cycle Count"=w2295:dbl, "2015 Cycle Stats.Max Shaft Speed"=w2294:dbl, "2015 Cycle Stats.Max Red. Pressure"=w2293:dbl)
        n901 = Build Array(w2301, w2300, w2299, w2298, w2297, w2296, w2295, w2294, w2293) -> (w2292:dbl[])
        n902 = Add Array Elements(numeric array=w2292) -> (sum=w2291:dbl)
        n903 = Equal To 0?(x=w2291) -> (x = 0?=w2290:bool)
        n904 = case shown="False" w2290 {
          tunnel: [0.0 ("Set Start Time (s)") 0.0 ("Set Start Time (s)")] -> w2307
          frame False {
          }
          frame True {
          }
        }
        n905 = call "UTILITY E-Time.vi"("Set Start Time (s)"=w2307, "error in (no error)"=w2304, "Reset"=w2290) -> ("error out"=w2303:errorcluster, "Elapsed Time (sec)"=→"Cycle Timer":dbl)  [unwired: 6 in, 1 out]
        n906 = call <vilib>:"Add State(s) to Queue__jki_lib_state_machine.vi"("State(s) in (\"\")"=w2305) -> ("States Out"=w2308:string)  [unwired: 14 in]
      }
    }
  }
  n907 = while "ERD Data Loop" {
    shift-right: [w2311] -> w17
    shift-left: w11 -> [w2312]
    tunnel: w60 -> [w2335]
    shift-right: [w2328] -> _
    shift-left: w63 -> [w2331]
    tunnel: [w2327] -> w55
    tunnel: T16[] [{"ERD Number"=61706, "Data Type"=enum."uint8_t"}, {"ERD Number"=62233, "Data Type"=enum."string"}, {"ERD Number"=61967, "Data Type"=enum."uint16_t"}, {"ERD Number"=61959, "Data Type"=enum."string"}, {"ERD Number"=62219, "Data Type"=enum."uint16_t"}, {"ERD Number"=62221, "Data Type"=enum."uint16_t"}, {"ERD Number"=61953, "Data Type"=enum."uint16_t"}, {"ERD Number"=61954, "Data Type"=enum."uint32_t"}, {"ERD Number"=61708, "Data Type"=enum."uint8_t"}, {"ERD Number"=61963, "Data Type"=enum."uint8_t"}, {"ERD Number"=62237, "Data Type"=enum."uint8_t"}, {"ERD Number"=61961, "Data Type"=enum."uint8_t"}, {"ERD Number"=61968, "Data Type"=enum."string"}, {"ERD Number"=61969, "Data Type"=enum."string"}, {"ERD Number"=61964, "Data Type"=enum."string"}, {"ERD Number"=62227, "Data Type"=enum."uint8_t"}, {"ERD Number"=61971, "Data Type"=enum."string"}, {"ERD Number"=8195, "Data Type"=enum."uint32_t"}, {"ERD Number"=62218, "Data Type"=enum."uint16_t"}, {"ERD Number"=62241, "Data Type"=enum."string"}, {"ERD Number"=61976, "Data Type"=enum."string"}, {"ERD Number"=62243, "Data Type"=enum."string"}, {"ERD Number"=61731, "Data Type"=enum."string"}, {"ERD Number"=61732, "Data Type"=enum."string"}, {"ERD Number"=61698, "Data Type"=enum."string"}, {"ERD Number"=61699, "Data Type"=enum."string"}, {"ERD Number"=61697, "Data Type"=enum."string"}, {"ERD Number"=61704, "Data Type"=enum."string"}, {"ERD Number"=61701, "Data Type"=enum."string"}, {"ERD Number"=61702, "Data Type"=enum."string"}, {"ERD Number"=61705, "Data Type"=enum."string"}, {"ERD Number"=61703, "Data Type"=enum."string"}, {"ERD Number"=61709, "Data Type"=enum."uint16_t"}, {"ERD Number"=61710, "Data Type"=enum."uint16_t"}, {"ERD Number"=61726, "Data Type"=enum."string"}, {"ERD Number"=62213, "Data Type"=enum."uint16_t"}, {"ERD Number"=61952, "Data Type"=enum."uint16_t"}, {"ERD Number"=61957, "Data Type"=enum."uint16_t"}, {"ERD Number"=61958, "Data Type"=enum."uint8_t"}, {"ERD Number"=61973, "Data Type"=enum."uint32_t"}, {"ERD Number"=62242, "Data Type"=enum."string"}, {"ERD Number"=256, "Data Type"=enum."string"}, {"ERD Number"=61441, "Data Type"=enum."string"}, {"ERD Number"=61457, "Data Type"=enum."string"}, {"ERD Number"=61995, "Data Type"=enum."uint16_t"}, {"ERD Number"=61985, "Data Type"=enum."uint16_t"}, {"ERD Number"=61986, "Data Type"=enum."uint16_t"}, {"ERD Number"=65535, "Data Type"=enum."string"}, {"ERD Number"=65535, "Data Type"=enum."string"}, {"ERD Number"=65535, "Data Type"=enum."string"}, {"ERD Number"=61977, "Data Type"=enum."string"}, {"ERD Number"=61990, "Data Type"=enum."string"}, {"ERD Number"=61988, "Data Type"=enum."uint16_t"}, {"ERD Number"=61987, "Data Type"=enum."uint16_t"}, {"ERD Number"=61989, "Data Type"=enum."uint16_t"}, {"ERD Number"=61991, "Data Type"=enum."string"}, {"ERD Number"=62212, "Data Type"=enum."uint16_t"}, {"ERD Number"=62211, "Data Type"=enum."uint16_t"}, {"ERD Number"=62210, "Data Type"=enum."uint16_t"}, {"ERD Number"=62208, "Data Type"=enum."uint16_t"}, {"ERD Number"=62253, "Data Type"=enum."uint16_t"}, {"ERD Number"=62213, "Data Type"=enum."uint16_t"}, {"ERD Number"=62254, "Data Type"=enum."uint16_t"}, {"ERD Number"=62209, "Data Type"=enum."uint16_t"}, {"ERD Number"=61962, "Data Type"=enum."string"}, {"ERD Number"=62229, "Data Type"=enum."string"}, {"ERD Number"=62214, "Data Type"=enum."string"}, {"ERD Number"=62215, "Data Type"=enum."string"}, {"ERD Number"=62230, "Data Type"=enum."string"}, {"ERD Number"=62216, "Data Type"=enum."string"}, {"ERD Number"=62231, "Data Type"=enum."string"}, {"ERD Number"=61760, "Data Type"=enum."uint32_t"}] ("Read ERD List") -> [w2317]
    tunnel: w14 -> [w2336]
    shift-right: [w2325] -> _
    shift-left: _ -> [w2324]
    tunnel: w32 -> [w2322]
    tunnel: [w2321] -> w20
    tunnel: "GEA Inputs" -> [w2314]
    stop <- w2326 stop-if-true
    n908 = Dequeue Element(queue=w2335, timeout in ms (-1)=10, error in (no error)=w2312) -> (queue out=w2334:refnum<queue>, element=w2332:T44, timed out?=w2320:bool, error out=w2313:errorcluster)
    n909 = Unbundle By Name(w2332) -> ("State"=w2330:enum16{"Run", "Shutdown"})
    "State" <- w2330
    n910 = call "Graph ERD Read List.vi"("ERD Graph Cntrl"="ERD Graph Cntrl") -> ("Array"=w2316:T16[])  [unwired: 10 in]
    n911 = Select(t=w2331, s=w2320, f=w2330) -> (s? t:f=w2329:enum16{"Run", "Shutdown"})
    n912 = Replace Array Subset(array=w2317, new element=w2316, index=47) -> (w2315:T16[])
    n913 = case shown="\"Run\", Default" w2329 {
      selector: w2329 -> [w2346 w2433]
      tunnel: w2313 -> [w2352 w2427]
      tunnel: w2336 -> [w2345 w2422]
      tunnel: [w2350 w2423] -> w2311
      tunnel: w2334 -> [w2349 w2434]
      tunnel: [w2348 w2434] -> w2327
      tunnel: [w2347 w2433] -> w2328
      tunnel: w2315 -> [w2344 _]
      tunnel: [FALSE TRUE] -> w2326
      tunnel: [w2342 w2421] -> w2325
      tunnel: w2324 -> [w2341 w2421]
      tunnel: w2322 -> [w2339 _]
      tunnel: [w2338 w2422] -> w2321
      tunnel: w2314 -> [w2337 _]
      frame "Run", Default {
        n914 = local write "Start Save Routine"(TRUE ("Start Save Routine")) -> ()
        n915 = case shown="True" "Data ON" {
          tunnel: w2352 -> [w2357 w2387]
          tunnel: w2345 -> [w2353 w2376]
          tunnel: [w2357 w2386] -> w2350
          tunnel: w2349 -> [w2356 w2385]
          tunnel: [w2356 w2385] -> w2348
          tunnel: [w2355 w2384] -> w2347
          tunnel: w2346 -> [w2355 w2384]
          tunnel: w2344 -> [_ w2377]
          tunnel: [w2354 w2370] -> w2342
          tunnel: w2341 -> [w2354 w2383]
          tunnel: w2339 -> [_ w2380]
          tunnel: [w2353 w2373] -> w2338
          tunnel: w2337 -> [_ w2363]
          frame False {
          }
          frame True {
            # "Add the serial number to the data"
            n916 = disable-structure shown="Enabled" {
              disable-tunnel: w2387 -> [w2396 w2397]
              disable-tunnel: w2377 -> [w2395 _]
              disable-tunnel: [w2389 w2397] -> w2369
              disable-tunnel: w2363 -> [w2388 _]
              frame Disabled {
                n917 = call "Convert Read ERD List to Message.vi"("GEA Inputs"=w2388, "Read ERD List"=w2395, "Error In"=w2396) -> ("GEA Message"=w2391:T10, "Error Out"=w2390:errorcluster)  [unwired: 11 in]
                n918 = call "GEA2MessageFormatter.vi"("Prefix(Send/Recv)"="SEND", "GEA2 Data In"=w2391, "Error In"=w2390) -> ("Output String"=w2392:string, "Error Out"=w2393:errorcluster)  [unwired: 11 in]
                n919 = call "GExplorer_Queue_GEA2.vi"("Output String"=w2392, "error in (no error)"=w2393) -> ("error out"=w2389:errorcluster)  [unwired: 13 in]
              }
              frame Enabled {
              }
            }
            n920 = call "GEA2 Read ERD Multiple Messages.vi"("GeaCommunication.GeaBus"=w2376, "Read Timeout (ms)"="Read Timeout (ms)", "GEA Inputs"=w2363, "Read ERD List"=w2377, "Expected Command 2"="Expected Command 2", "Expected Data 2"="Expected Data 2", "Error In"=w2369, "#ERDs per message"=12, "Verify ERD Response?"="Verify ERD Response?", "Disable Expected Data"="Disable Expected Data") -> ("GeaCommunication.GeaBus"=w2373:refnum<k24>, "Raw Data Out"=w2371:string[], "ERD Data Out"=w2372:T2[], "Error Out"=w2364:errorcluster)  [unwired: 2 in]
            "ERD Data Out" <- w2372
            "Raw Data Out" <- w2371
            n921 = call "Convert_Always_Show_Info.vi"("Array"=w2372, "Raw Data Out"=w2371, "Previous ERD Info"=w2383, "Error In"=w2364) -> ("Version"=→"Version":T11, "ERD_Always Show"=w2370:T1, "Redundant Micro"=→"Redundant Micro":T33, "ATC Data"=→"ATC Data":T37, "ERD Graph  Ind"=w2365:T20, "Algorithm Data 2"=→"Algorithm Data":T36, "Error Out"=w2379:errorcluster)  [unwired: 4 in, 1 out]
            "ERD Graph  Ind" <- w2365
            n922 = case shown="True" "Disable Graphs" {
              tunnel: [w2419 w2420] -> w2386
              tunnel: w2379 -> [w2418 w2420]
              tunnel: w2370 -> [w2417 _]
              tunnel: w2365 -> [w2407 _]
              frame False {
                n923 = control-ref of="Temp"() -> (w2398:refnum<vi>)
                n924 = control-ref of="Basket Speed"() -> (w2406:refnum<vi>)
                n925 = control-ref of="Tub Gallons"() -> (w2405:refnum<vi>)
                n926 = control-ref of="Pressure 2"() -> (w2404:refnum<vi>)
                n927 = control-ref of="Motor Current"() -> (w2403:refnum<vi>)
                n928 = control-ref of="ERD 1"() -> (w2402:refnum<vi>)
                n929 = control-ref of="ERD 2"() -> (w2401:refnum<vi>)
                n930 = control-ref of="ERD 3"() -> (w2400:refnum<vi>)
                n931 = Build Array(w2398, w2406, w2405, w2404, w2403, w2402, w2401, w2400) -> (w2399:refnum<vi>[])
                n932 = call "Update Graphs.vi"("ERD_Always Show"=w2417, "Select Graph"="Select Graph", "appended array"=w2399, "ERD Graph  Ind 2"=w2407, "Error In"=w2418) -> ("ERD 1"=→"ERD 1":dbl, "Motor Current"=→"Motor Current":dbl, "ERD 2"=→"ERD 2":dbl, "Temp"=→"Temp":dbl, "Basket Speed"=→"Basket Speed":u16, "ERD 3"=→"ERD 3":dbl, "Tub Gallons"=→"Tub Gallons":dbl, "Pressure 3"=→"Pressure 2":dbl, "Error Out"=w2419:errorcluster)  [unwired: 6 in]
              }
              frame True {
              }
            }
            n933 = Bundle By Name(cluster=w2370, "Serial Number"=w2380) -> (→"ERD Data":T1)
            n934 = call "UTILITY E-Time.vi"() -> ("Elapsed Time (sec)"=→"Timer 2":dbl)  [unwired: 9 in, 2 out]
          }
        }
      }
      frame "Shutdown" {
        w2430 = FALSE ("Blinking")
        n935 = property on="Filter Data" class="Bool (strict)"(error in=w2427, "Value"=TRUE) -> (error out=w2426:errorcluster)  [unwired: 1 in, 1 out]
        n936 = property on="Data ON" class="Bool (strict)"(error in=w2426, "Value"=FALSE ("Data ON")) -> (error out=w2425:errorcluster)  [unwired: 1 in, 1 out]
        n937 = property on="Open Lid" class="Bool (strict)"(error in=w2425, "Value"=FALSE) -> (error out=w2424:errorcluster)  [unwired: 1 in, 1 out]
        n938 = property on="Program Ind" class="Bool (strict)"(error in=w2424, "Blinking"=w2430, "Value"=w2430) -> (error out=w2423:errorcluster)  [unwired: 1 in, 1 out]
      }
    }
    n939 = Wait Until Next ms Multiple(millisecond multiple="Sample Rate (ms)") -> ()  [unwired: 1 out]
  }
  n940 = disable-structure shown="Disabled" {
    disable-tunnel: [w2437 w2473] -> w84
    disable-tunnel: w74 -> [w2436 _]
    disable-tunnel: w12 -> [w2435 w2473]
    frame Disabled {
      n941 = while "GEA2 Receive Event Loop" {
        tunnel: w2436 -> [w2442]
        shift-right: [w2438] -> w2437
        shift-left: w2435 -> [w2441]
        stop <- w2440 stop-if-true
        n942 = event shown="[1] <Receive Loop Error>: User Event" {
          selector: w2442 -> [w2451 _ _]
          dyn-events: _ -> [_ _ _]
          timeout: _ -> [_ _ _]
          tunnel: w2441 -> [w2448 w2469 w2472]
          tunnel: [w2458 w2469 w2472] -> w2439
          tunnel: [_ w2470 TRUE] -> w2440
          event User Event {
            n943 = event-data() -> ("Source"=w2454:u8, "Destination"=w2455:u8, "Command"=w2463:u8, "Message"=w2462:string)  [unwired: 1 in]
            n944 = Bundle By Name(cluster=T10 {"Source"=0, "Destination"=0, "Command"=0, "Message"=""} ("GEA2 Data In"), "Source"=w2454, "Destination"=w2455, "Command"=w2463, "Message"=w2462) -> (w2460:T10)
            n945 = Flush Event Queue(0:w2451, 2:lveventtype."User Event" ("event type or object"), 3:w2448, 5:10 ("keep most recent")) -> (11:w2447:errorcluster)  [unwired: 2 in, 2 out]
            n946 = call "GEA2MessageFormatter.vi"("Prefix(Send/Recv)"="RECV", "GEA2 Data In"=w2460) -> ("Output String"=w2459:string)  [unwired: 12 in, 1 out]
            n947 = Equal?(x=w2455, y=u8 240) -> (x = y?=w2452:bool)
            n948 = And(x="Filter Data", y=w2452) -> (x .and. y?=w2456:bool)
            n949 = case shown="True" w2456 {
              tunnel: w2459 -> [w2465 _]
              tunnel: w2447 -> [w2467 w2468]
              tunnel: [w2466 w2468] -> w2458
              frame False {
                n950 = call "GExplorer_Queue_GEA2.vi"("Output String"=w2465, "error in (no error)"=w2467) -> ("error out"=w2466:errorcluster)  [unwired: 13 in]
              }
              frame True {
              }
            }
          }
          event User Event {
            n951 = event-data() -> ("status"=w2470:bool)  [unwired: 1 in]
          }
          event "Stop": Value Change {
            n952 = event-data() -> ()  [unwired: 1 in, 1 out]
          }
        }
        n953 = disable-structure shown="Enabled" {
          disable-tunnel: w2439 -> [w2444 w2445]
          disable-tunnel: [w2443 w2446] -> w2438
          frame Disabled {
            n954 = call "Error_Control.vi"("Error In"=w2444) -> ("Error Out"=w2443:errorcluster)  [unwired: 14 in]
          }
          frame Enabled {
            n955 = call <vilib>:"Clear Errors.vi"("error in (no error)"=w2445) -> ("error out"=w2446:errorcluster)  [unwired: 5 in, 1 out]
          }
        }
      }
    }
    frame Enabled {
    }
  }
  n956 = disable-structure shown="Disabled" {
    disable-tunnel: [w2477 w2516] -> w81
    disable-tunnel: [w2476 w2517] -> w79
    disable-tunnel: w59 -> [w2475 w2517]
    disable-tunnel: w12 -> [w2474 w2516]
    frame Disabled {
      n957 = while "GEA2 Display Loop" {
        tunnel: w2475 -> [w2482]
        shift-right: [w2481] -> _
        shift-left: _ -> [w2484]
        shift-right: [w2478] -> w2477
        shift-left: w2474 -> [w2488]
        tunnel: [w2482] -> w2476
        stop <- w2480 stop-if-true
        n958 = Dequeue Element(queue=w2482, error in (no error)=w2488) -> (element=w2487:T46, error out=w2483:errorcluster)  [unwired: 1 in, 2 out]
        n959 = Unbundle By Name(w2487) -> ("Data"=w2485:variant, "State"=w2486:enum16{"Add to Log", "Clear", "Shutdown"})
        n960 = case shown="\"Add to Log\", Default" w2486 {
          tunnel: w2485 -> [w2503 _ _]
          tunnel: w2484 -> [w2506 w2511 _]
          tunnel: [w2505 w2511 ""] -> w2481
          tunnel: w2483 -> [w2504 w2512 w2515]
          tunnel: [w2501 w2512 w2515] -> w2479
          tunnel: [_ TRUE _] -> w2480
          frame "Add to Log", Default {
            n961 = Variant To Data(error in=w2504, type="", Variant=w2503) -> (data=w2493:string, error out=w2501:errorcluster)
            n962 = local read "Filter Data"() -> (w2494:bool)
            n963 = String Subset(string=w2493, offset (0)=22, length (rest)=7 ("length (rest)")) -> (substring=w2497:string)
            n964 = Equal?(x="SEND F0", y=w2497) -> (x = y?=w2495:bool)
            n965 = And(x=w2494, y=w2495) -> (x .and. y?=w2496:bool)
            n966 = case shown="False" w2496 {
              tunnel: w2506 -> [w2508 w2510]
              tunnel: [w2507 w2510] -> w2505
              tunnel: w2493 -> [w2509 _]
              frame False {
                n967 = Concatenate Strings(w2509, w2508) -> (w2507:string)
              }
              frame True {
              }
            }
          }
          frame "Shutdown" {
          }
          frame "Clear" {
          }
        }
        "GEA2 Msg Log" <- w2481
        n968 = disable-structure shown="Enabled" {
          disable-tunnel: w2479 -> [w2490 w2492]
          disable-tunnel: [w2489 w2491] -> w2478
          frame Disabled {
            n969 = call "Error_Control.vi"("Error In"=w2490) -> ("Error Out"=w2489:errorcluster)  [unwired: 14 in]
          }
          frame Enabled {
            n970 = call <vilib>:"Clear Errors.vi"("error in (no error)"=w2492) -> ("error out"=w2491:errorcluster)  [unwired: 5 in, 1 out]
          }
        }
      }
    }
    frame Enabled {
    }
  }
  n971 = call "GEA2 Stop.vi"("GEA2 Reference In"=w20, "Error In"=w17) -> ("Error Out"=w21:errorcluster)  [unwired: 13 in]
  n972 = Merge Errors(w22, w21, w81, w84, w18, w44, w53) -> (w87:errorcluster)
  n973 = Release Queue(queue=w55, error in (no error)=w87) -> (error out=w86:errorcluster)  [unwired: 1 in, 2 out]
  n974 = Release Queue(queue=w56, error in (no error)=w86) -> (error out=w80:errorcluster)  [unwired: 1 in, 2 out]
  n975 = Release Queue(queue=w79, error in (no error)=w80) -> (error out=w49:errorcluster)  [unwired: 1 in, 2 out]
  n976 = disable-structure shown="Disabled" {
    frame Disabled {
      n977 = call "Error_Control.vi"() -> ()  [unwired: 15 in, 1 out]
      n978 = call <vilib>:"Clear Errors.vi"() -> ()  [unwired: 6 in, 2 out]
    }
    frame Enabled {
    }
  }
  n979 = disable-structure shown="Disabled" {
    frame Disabled {
      n980 = call <vilib>:"Clear Errors.vi"() -> ()  [unwired: 6 in, 2 out]
      n981 = call "Error_Control.vi"() -> ()  [unwired: 15 in, 1 out]
    }
    frame Enabled {
    }
  }
  n982 = Release Queue(queue=w48, error in (no error)=w49) -> (error out=w47:errorcluster)  [unwired: 1 in, 2 out]
  n983 = disable-structure shown="Disabled" {
    disable-tunnel: [w2519 w2521] -> w54
    disable-tunnel: w47 -> [w2518 w2521]
    frame Disabled {
      n984 = call "Error_Control.vi"("Command (Handle Errors)"=Error_Command."Report Errors", "Error In"=w2518) -> ("Error Out"=w2519:errorcluster)  [unwired: 13 in]
    }
    frame Enabled {
    }
  }
  "Error Out" <- w54
